vi "DL-SMART-MS-Modify-05-25-6.0.vi"() -> ()   [LabVIEW 2013]
uses:
  <vilib>/Utility/file.llb/Read From Spreadsheet File (DBL).vi
  <userlib>/caLab/Private/CaLabEvent_PV-1D.vi
  <vilib>/Utility/file.llb/Write To Spreadsheet File (DBL).vi
  <userlib>/caLab/Private/Put_DBL-1D_PV.vi
  <userlib>/caLab/Private/Put_I32_PV.vi
  cal_p.vi
  <userlib>/caLab/Private/Get_PV.vi
  <vilib>/vision/driver/NI_Vision_Acquisition_Software.lvlib
  <resource>/objmgr/imaqdx.rc
  <vilib>/Analysis/NI_AALPro.lvlib
panel:
  out "idn status":string
  out "MS":cluster{dbl[], "filtered data":dbl[]}(graph)
  out "std sample":T1(array[cluster])
  in  "Set Laser":bool
  out "Image":T2(plugin-control)
  out "selected id":i32
  out "selected row":i32
  out "currentNO":string
  out "commet":string
  out "sampleID":string
  in  "Shots/Point":i32=100
  in  "chamber in":bool caption="TakeMS"
  in  "chamber out":bool caption="TakeMS"
  in  "Laser parameter":T4
  in  "ADC parameter":T5
  in  "ShutDownSystem":bool
  in  "ADC reference":refnum<vi>
  in  "SetLaserEnergy":dbl(slide) min=0.0 max=50.0 scale=0.0..10.0
  in  "LaserHV":u8=50 min=1 max=100
  in  "频率/Hz":u8=60
  out "Pul.HV-Real":dbl
  out "Identify Spcetrum":cluster{"ID1:X":dbl[], "ID1:Y":dbl[]}[](graph)
  in  "测试记录":i32(listbox)=6
  in  "Identification Results (单靶鉴定结果)":i32(listbox)=2
  in  "HVEnable":bool
  out "GateClose":bool
  out "LaserOK":bool
  out "HV-OK":bool
  out "Vacuum-OK":bool
  in  "Tab Control":T6(tab)
  in  "helix-Zeta-Step":dbl=100.0
  in  "helix-b":dbl=0.2
  in  "AcquireMS-Methods":u8(ring) items=["SinglePoint", "Multipoints", "MultiTar"]
  in  "Thresh":dbl=-0.005 format="%#_13g"
  in  "right rank":i32=2
  in  "left rank":i32=2
  in  "deBaseline":bool
  in  "MCPHV-Set":dbl=1400.0 min=0.0 max=1600.0
  in  "LensHV-Set":dbl=8000.0 min=0.0 max=10000.0
  in  "Tar.HV-Set":dbl=18010.0 min=0.0 max=20000.0
  in  "Pul.HV-Set":dbl=1400.0 min=0.0 max=2000.0
  in  "PulseDelay":dbl
  in  "ADCFreq":dbl
  in  "CH1_Coupling":u64(ring)=2 items=["Volt DC"=1, "Volt AC"=2, "Ampere DC"=4, "Ampere AC"=8, "Ohm"=16]
  in  "Channel 1_Range":dbl(ring)=4.0 items=["80 V"=80.0, "40 V"=40.0, "20 V"=20.0, "8 V"=8.0, "4 V"=4.0, "2 V"=2.0, "800 mV"=0.8, "400 mV"=0.4, "200 mV"=0.2]
  in  "Anal. Setting File":string="High Mass"
  in  "SettingFileSave":bool caption="TakeMS"
  in  "SettingFileAppl":bool caption="TakeMS"
  in  "SettingDel":bool caption="TakeMS"
  in  "RunADC":bool caption="TakeMS"
  out "ADCstatus":bool
  in  "Vac_Prot.":bool
  in  "Turbo_Fore":bool
  in  "Main_Samp":bool
  in  "Samp_Atmos":bool
  in  "Fore_Samp":bool
  in  "StartPump":bool
  in  "SopPump":bool
  out "TurboSpeed":dbl(knob) scale=0.0..100.0
  out "PumpKW":dbl
  out "PumpAmps":dbl
  out "PumpTemp":u16
  out "PumpVolts":dbl
  in  "laser OFF":bool
  in  "laser ON":bool
  out "cluster":T7
  out "A1-position-Y":dbl=45.0 caption="Y" min=0.0 max=55.0
  out "A1-position-X":dbl=53.4 caption="X" min=0.0 max=55.0
  in  "GO":bool
  in  "Y":dbl min=0.0 max=55.0
  in  "X":dbl min=0.0 max=55.0
  in  "A1-Position":bool caption="X-"
  in  "Plat_To_Zero":bool caption="TakeMS"
  in  "Plat_Cal":bool caption="TakeMS"
  out "Y当前":dbl
  out "X当前":dbl
  out "移动":bool
  out "Y满":bool
  out "Y标":bool
  out "X满":bool
  out "Y0":bool
  out "X0":bool
  out "靶位In/Out":bool
  out "仓门":bool
  out "Y过热":bool
  out "X过热":bool
  out "通讯":bool
  in  "Operation Record":i32(listbox)
  in  "OptionRecordLoad 2":bool caption="TakeMS"
  in  "OptionRecordClear":bool caption="TakeMS"
  out "c:":dbl
  out "b:":dbl
  out "a:":dbl
  in  "cancel cal":bool
  in  "cal save":bool
  in  "peak cal":bool
  in  "peak detect":bool
  in  "标准样品":u16(ring) items=["肺炎克雷伯菌", "铜绿假单胞菌"]
  in  "定标参数":i32(listbox)
  out "Tar.HV-Real":dbl
  out "LensHV-Real":dbl
  out "MCPHV-Real":dbl
  out "Lvaccum":dbl=0.83 format="%#_2e"
  out "Hvaccum":dbl=3.4e-05 format="%#_2e"
  in  "H12":bool
  in  "G12":bool
  in  "F12":bool
  in  "E12":bool
  in  "D12":bool
  in  "C12":bool
  in  "B12":bool
  in  "A12":bool
  in  "H11":bool
  in  "G11":bool
  in  "F11":bool
  in  "E11":bool
  in  "D11":bool
  in  "C11":bool
  in  "B11":bool
  in  "A11":bool
  in  "H10":bool
  in  "G10":bool
  in  "F10":bool
  in  "E10":bool
  in  "D10":bool
  in  "C10":bool
  in  "B10":bool
  in  "A10":bool
  in  "H9":bool
  in  "G9":bool
  in  "F9":bool
  in  "E9":bool
  in  "D9":bool
  in  "C9":bool
  in  "B9":bool
  in  "A9":bool
  in  "H8":bool
  in  "G8":bool
  in  "F8":bool
  in  "E8":bool
  in  "D8":bool
  in  "C8":bool
  in  "B8":bool
  in  "A8":bool
  in  "H7":bool
  in  "G7":bool
  in  "F7":bool
  in  "E7":bool
  in  "D7":bool
  in  "C7":bool
  in  "B7":bool
  in  "A7":bool
  in  "H6":bool
  in  "G6":bool
  in  "F6":bool
  in  "E6":bool
  in  "D6":bool
  in  "C6":bool
  in  "B6":bool
  in  "A6":bool
  in  "H5":bool
  in  "G5":bool
  in  "F5":bool
  in  "E5":bool
  in  "D5":bool
  in  "C5":bool
  in  "B5":bool
  in  "A5":bool
  in  "H4":bool
  in  "G4":bool
  in  "F4":bool
  in  "E4":bool
  in  "D4":bool
  in  "C4":bool
  in  "B4":bool
  in  "A4":bool
  in  "H3":bool
  in  "G3":bool
  in  "F3":bool
  in  "E3":bool
  in  "D3":bool
  in  "C3":bool
  in  "B3":bool
  in  "A3":bool
  in  "H2":bool
  in  "G2":bool
  in  "F2":bool
  in  "E2":bool
  in  "D2":bool
  in  "C2":bool
  in  "B2":bool
  in  "A2":bool
  in  "H1":bool
  in  "G1":bool
  in  "F1":bool
  in  "E1":bool
  in  "D1":bool
  in  "C1":bool
  in  "B1":bool
  in  "A1":bool
  in  "Clear":bool caption="TakeMS"
  in  "Add":bool caption="TakeMS"
  in  "TakeMS-Stop":bool caption="TakeMS"
  in  "TakeMS-Run":bool caption="TakeMS"
  # "Laser (激光)"
  # "Acq.(采谱)"
  # "Vacuum(真空)"
  # "Pa"
  # "High"
  # "1"
  # "2"
  # "3"
  # "4"
  # "5"
  # "6"
  # "7"
  # "8"
  # "9"
  # "10"
  # "11"
  # "12"
  # "A"
  # "Low"
  # "Pa"
  # "B"
  # "H.V.(高压)"
  # "C"
  # "D"
  # "MCP"
  # "V"
  # "E"
  # "Tar."
  # "V"
  # "F"
  # "Pul."
  # "V"
  # "G"
  # "Lens"
  # "V"
  # "H"
  # "Vauum (真空)"
  # "H.V. (高压)"
  # "Laser (激光)"
  # "Gate (仓门)"
  # "mm"
  # "Radian"
  # "H.V. (高压参数)"
  # "ADC(采集卡设置)"
  # "ADCFreq(采样)"
  # "MCP (探测器)"
  # "V"
  # "Hz"
  # "Tar. (靶)"
  # "V"
  # "Setting File(设置文件)"
  # "Coupling"
  # "Pulse (脉冲)"
  # "V"
  # "IntRange"
  # "V"
  # "Lens (透镜)"
  # "Delay (延时)"
  # "ns"
  # "Sole. Valves"
  # "Turbo Pump"
  # "自锁保护"
  # "机械/分子"
  # "主仓/样仓"
  # "样仓/大气"
  # "机械/样仓"
  # "激光器状态"
  # "mm"
  # "mm"
  # "mm"
  # "mm"
  # "mm"
  # "mm"
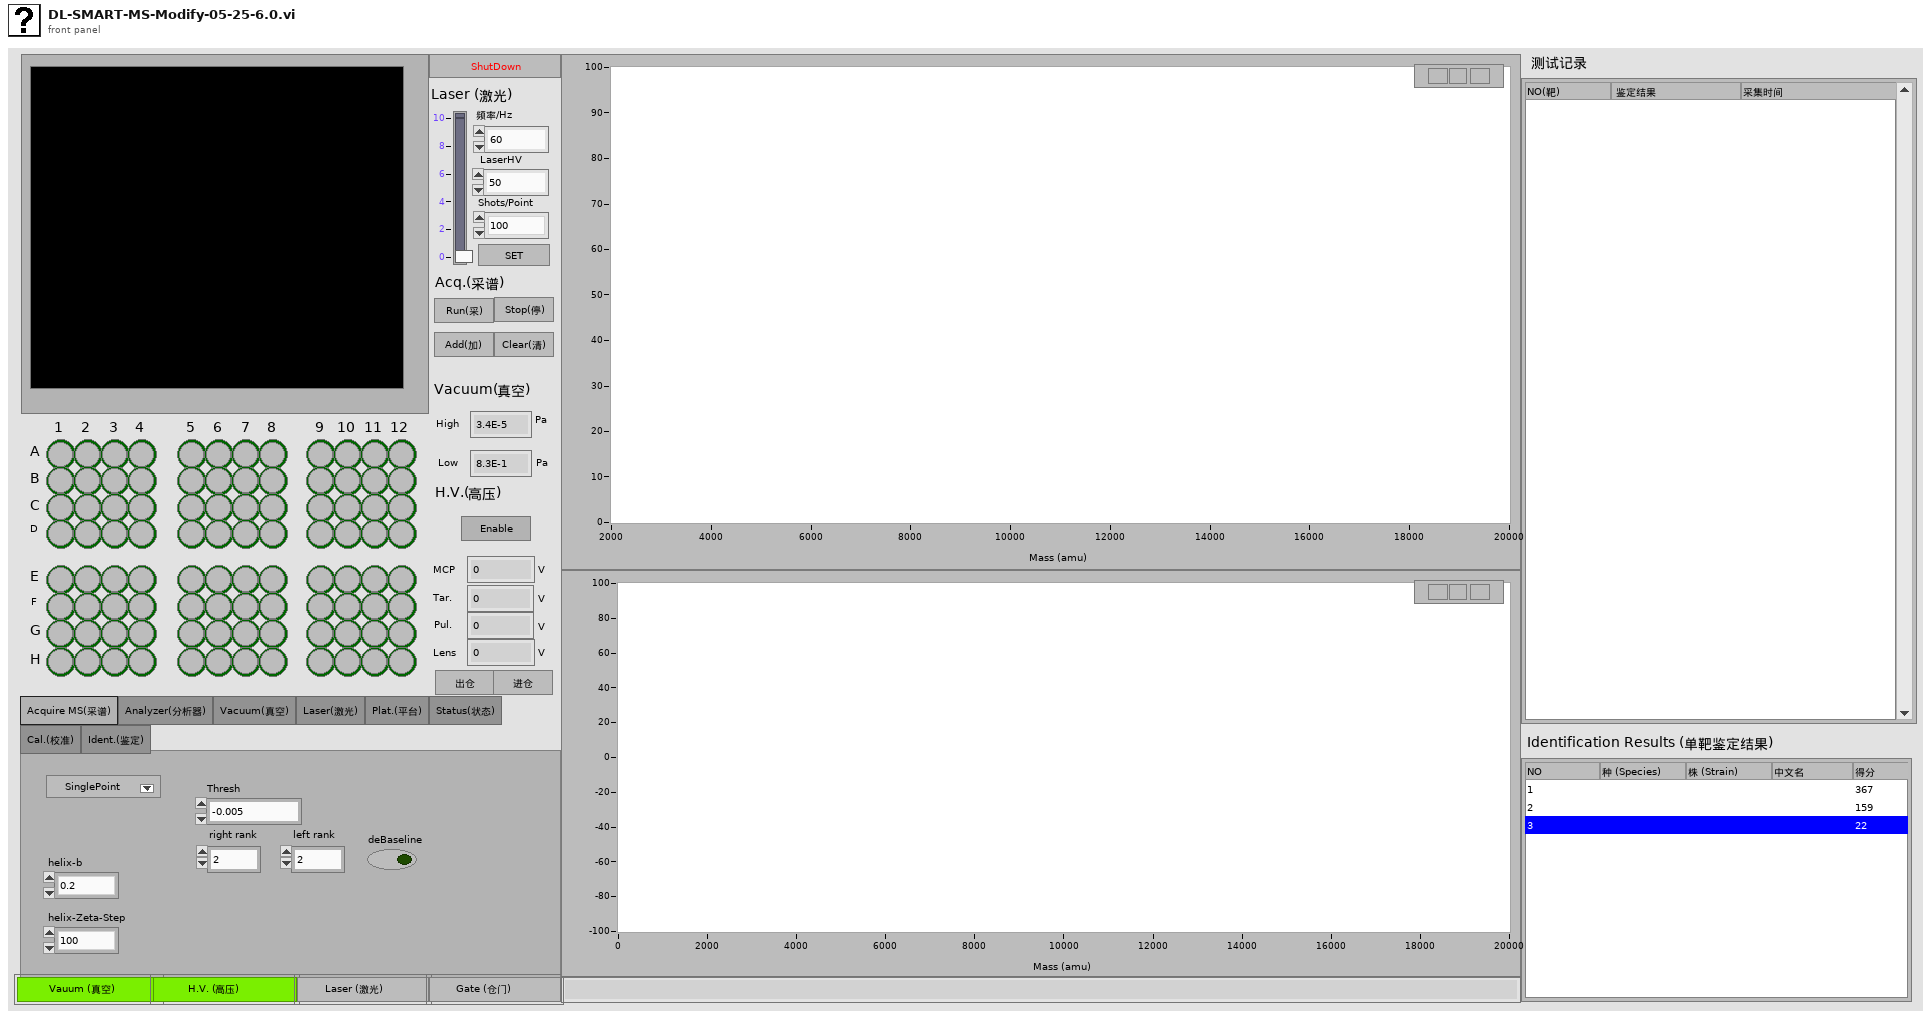
[diagram p1: front panel]
types:
  T1 = cluster{"name":string, "mz":dbl[], "time":dbl[]}[]
  T2 = typedef "IMAQ Image.ctl" = refnum<image>
  T3 = typedef "Semaphore RefNum" = refnum<k1>
  T4 = cluster{"VISA resource name":refnum<visa-resource-name>, "standby":bool, "semaphore in":T3, "SetLaserEnergy":dbl}
  T5 = cluster{"TpDeviceHandle_t":u32, "Record Length/Samples":u64, "ShotsPerPoint":u16}
  T6 = enum32{"Acquire MS(采谱)", "Analyzer(分析器)", "Vacuum(真空)", "Laser(激光)", "Plat.(平台)", "Status(状态)", "Cal.(校准)", "Ident.(鉴定)"}
  T7 = cluster{"链接":bool, "待机":bool, "发射":bool, "[3]":bool, "内存":bool, "测能":bool, "温警":bool, "静态":bool, "操作":bool}
  T8 = cluster{"tag1":string, "tag2":string, "x":dbl[], "y":dbl[], "ID1:X":dbl[], "ID1:Y":dbl[], "ID1:REF:X":dbl[], "ID1:REF:Y":dbl[], "ID2:X":dbl[], "ID2:Y":dbl[], "ID2:REF:X":dbl[], "ID2:REF:Y":dbl[], "ID3:X":dbl[], "ID3:Y":dbl[], "ID3:REF:X":dbl[], "ID3:REF:Y":dbl[], "ID1:TAG1":string, "ID1:TAG2":string, "ID2:TAG1":string, "ID2:TAG2":string, "ID3:TAG1":string, "ID3:TAG2":string, "ID1:NAME":string, "ID2:NAME":string, "ID3:NAME":string, "ID1:SCORE":string, "ID2:SCORE":string, "ID3:SCORE":string, "NO":string}[]
  T9 = cluster{"laser semaphore":T3, "pump semaphore":T3}
  T10 = enum8{"Enabled", "Disabled", "Disabled and Grayed Out"}
  T11 = cluster{"tag1":string, "tag2":string, "x":dbl[], "y":dbl[], "ID1:X":dbl[], "ID1:Y":dbl[], "ID1:REF:X":dbl[], "ID1:REF:Y":dbl[], "ID2:X":dbl[], "ID2:Y":dbl[], "ID2:REF:X":dbl[], "ID2:REF:Y":dbl[], "ID3:X":dbl[], "ID3:Y":dbl[], "ID3:REF:X":dbl[], "ID3:REF:Y":dbl[], "ID1:TAG1":string, "ID1:TAG2":string, "ID2:TAG1":string, "ID2:TAG2":string, "ID3:TAG1":string, "ID3:TAG2":string, "ID1:NAME":string, "ID2:NAME":string, "ID3:NAME":string, "ID1:SCORE":string, "ID2:SCORE":string, "ID3:SCORE":string, "NO":string}
  T12 = cluster{"monitor":refnum<user-event>, "motor status":refnum<user-event>, "motor":refnum<user-event>, "notifier out":refnum<notifier>, "queue out":refnum<queue>, "AI":T3, "DI":T3, "CX":T3, "CY":T3}
  T13 = cluster{"AI Task":refnum<k21>, "AO Task":refnum<k21>, "DO Task":refnum<k21>, "DI Task":refnum<k21>, "PWM x":refnum<k21>, "PWM y":refnum<k21>, "counter x":refnum<k21>, "counter y":refnum<k21>}
  T14 = cluster{"tasks":cluster{"AI Task":refnum<k21>, "AO Task":refnum<k21>, "DO Task":refnum<k21>, "DI Task":refnum<k21>, "PWM x":refnum<k21>, "PWM y":refnum<k21>, "counter x":refnum<k21>, "counter y":refnum<k21>}, "interface":cluster{"monitor":refnum<user-event>, "motor status":refnum<user-event>, "motor":refnum<user-event>, "notifier out":refnum<notifier>, "queue out":refnum<queue>, "AI":T3, "DI":T3, "CX":T3, "CY":T3}, "error out":errorcluster}
  T15 = cluster{"ConfiguredPumpCom":refnum<visa-resource-name>, "ConfiguredLaserCom":refnum<visa-resource-name>}
  T16 = typedef "LVPoint32TypeDef.ctl" = cluster{"Horizontal":i32, "Vertical":i32}
  T17 = typedef "LVRowAndColumnTypeDef.ctl" = cluster{"Row":i32, "Column":i32}
  T18 = cluster{"Type":u32, "Version":u32, "Flags":u32, "SerialNumberHigh":u32, "SerialNumberLow":u32, "BusType":u32, "InterfaceName":string, "VendorName":string, "ModelName":string, "CameraFileName":string, "CameraAttributeURL":string}[]
  T19 = cluster{"Type":u32, "Version":u32, "Flags":u32, "SerialNumberHigh":u32, "SerialNumberLow":u32, "BusType":u32, "InterfaceName":string, "VendorName":string, "ModelName":string, "CameraFileName":string, "CameraAttributeURL":string}
  T20 = typedef "IMAQdx.ctl" = refnum<k21>
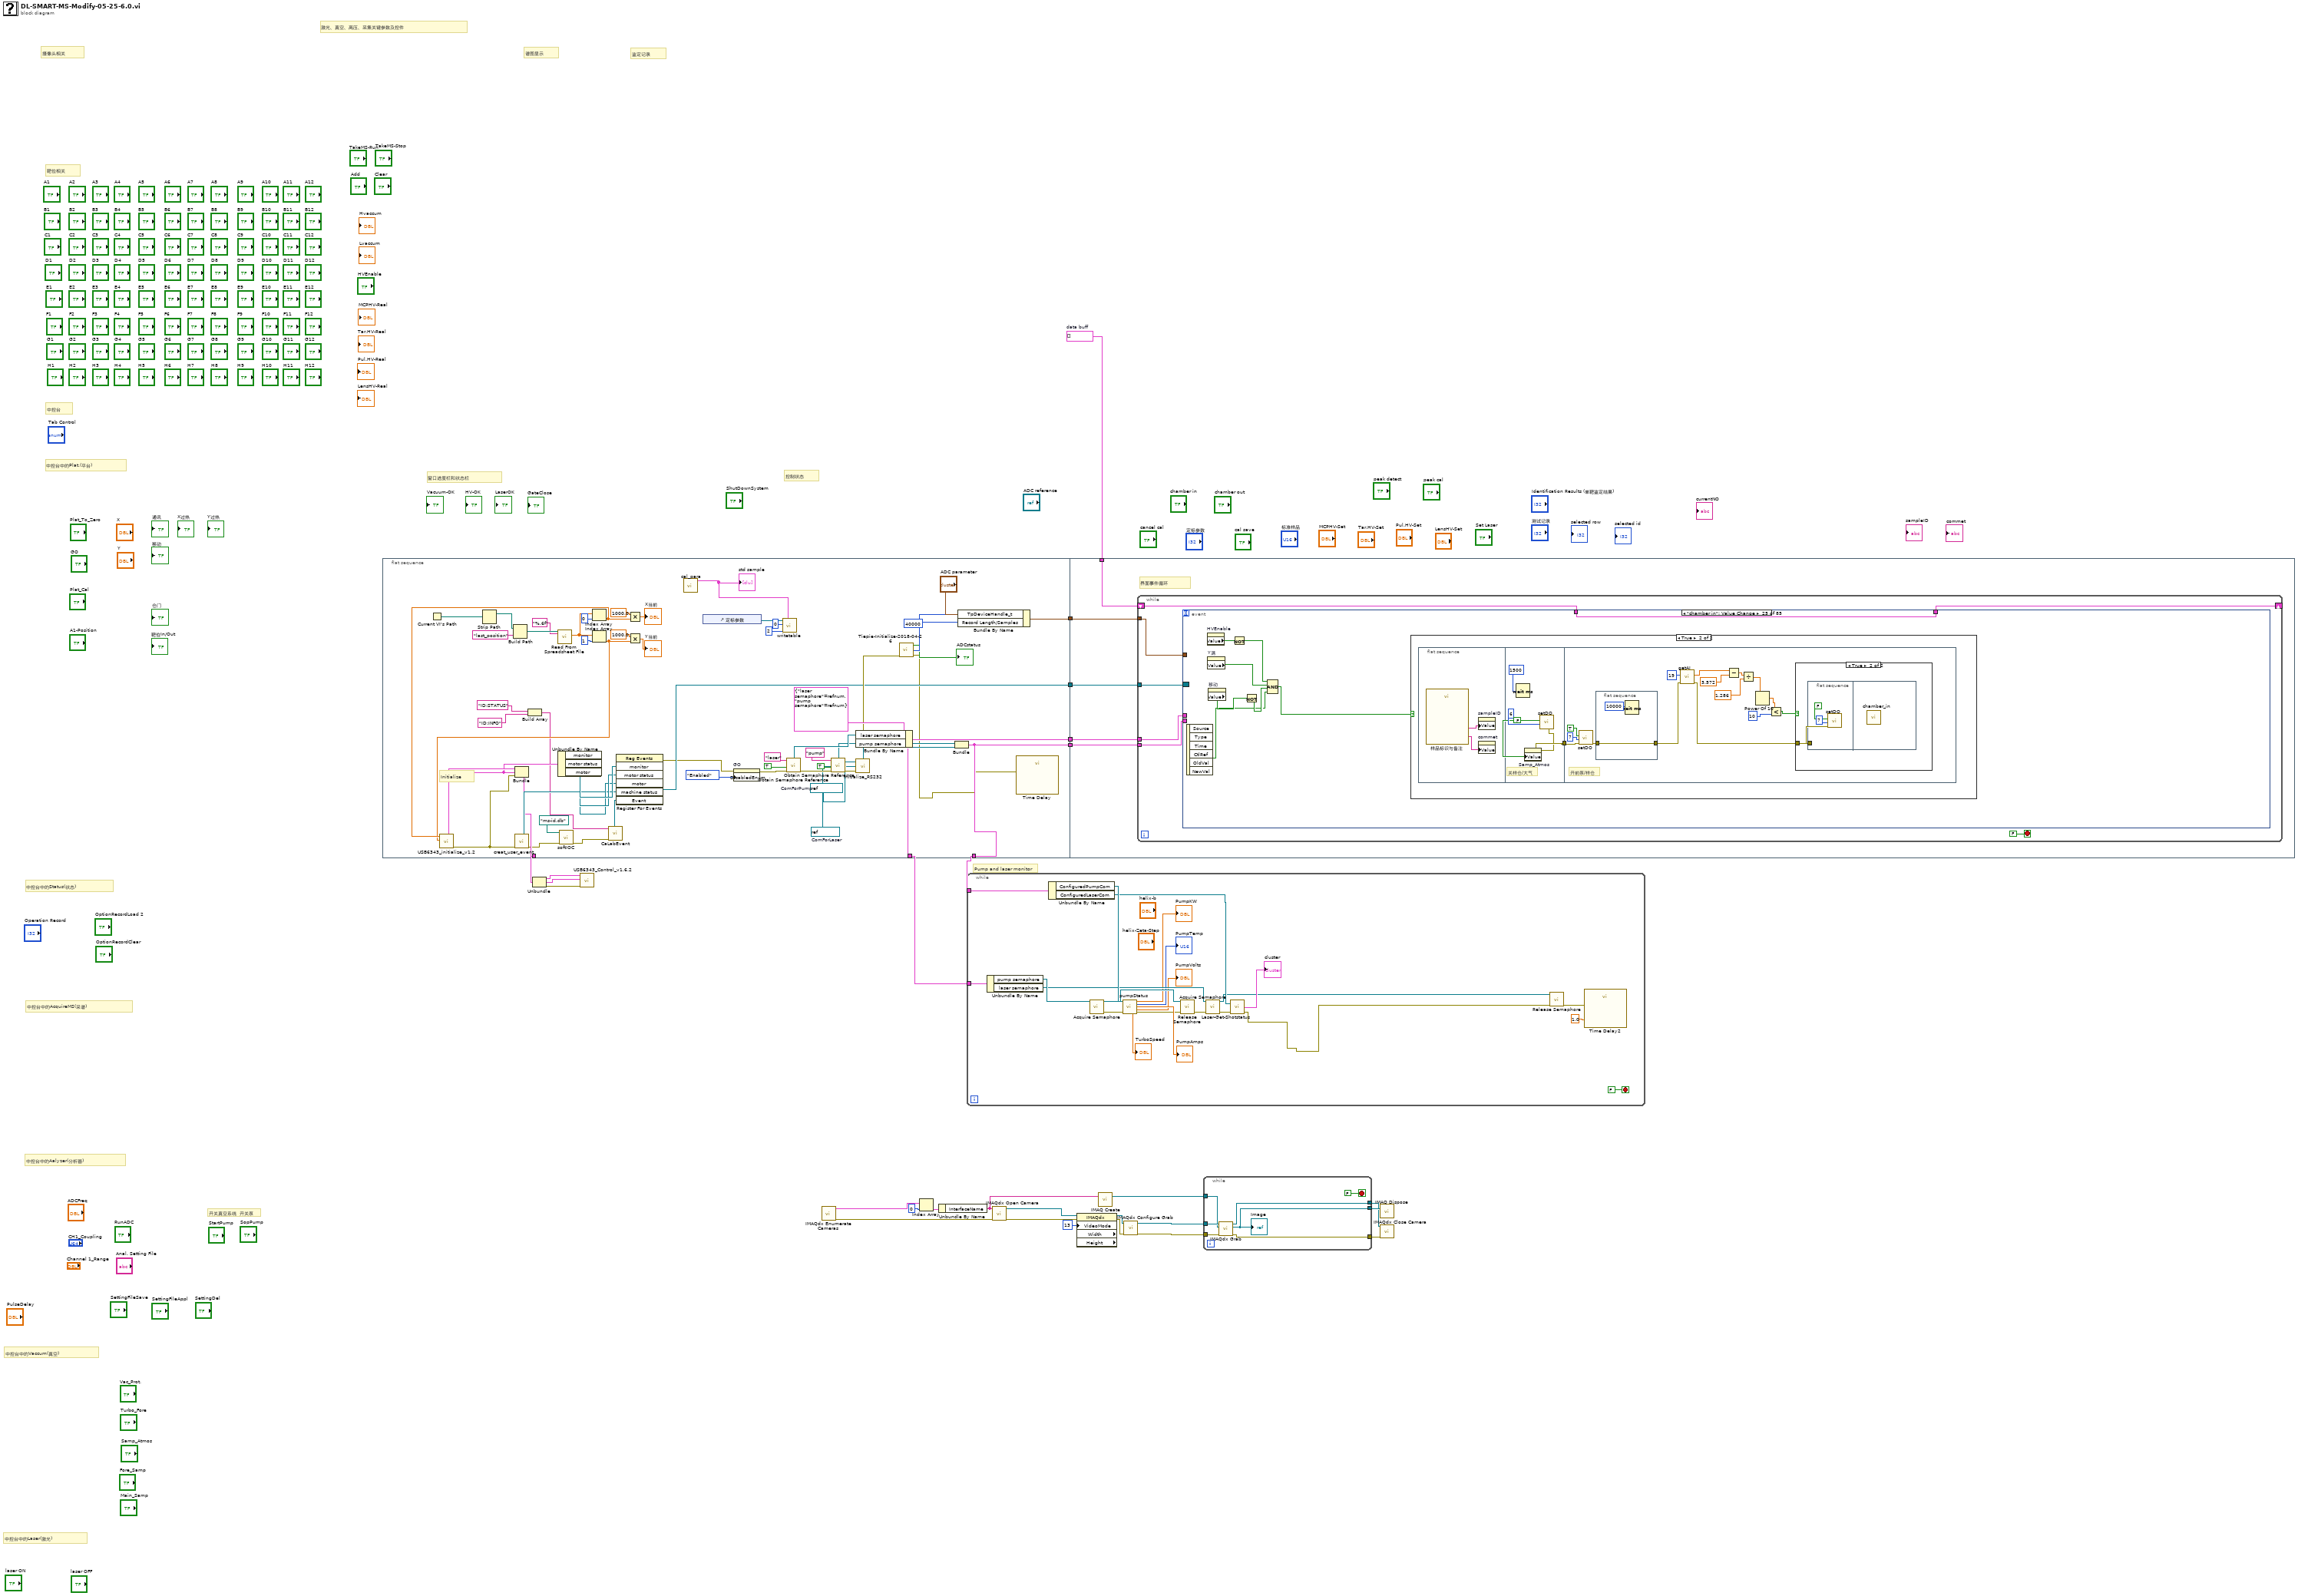
[diagram p0: block diagram]
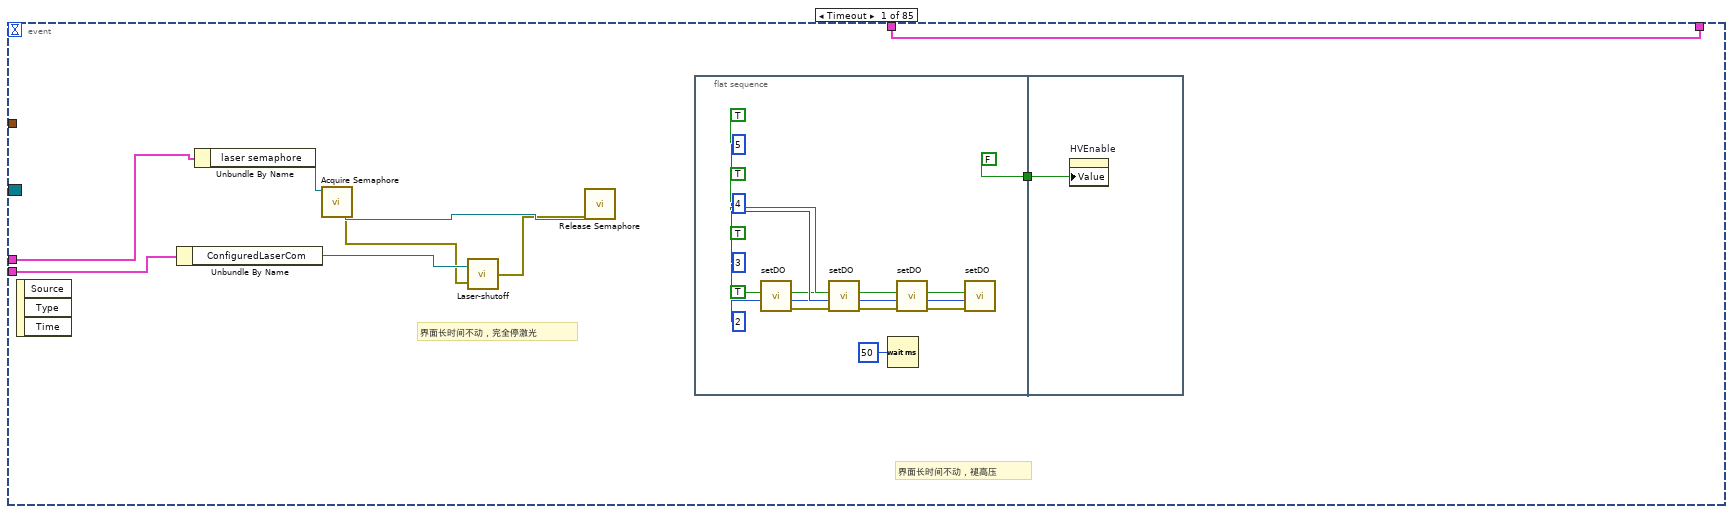
[diagram p2: hidden frame]
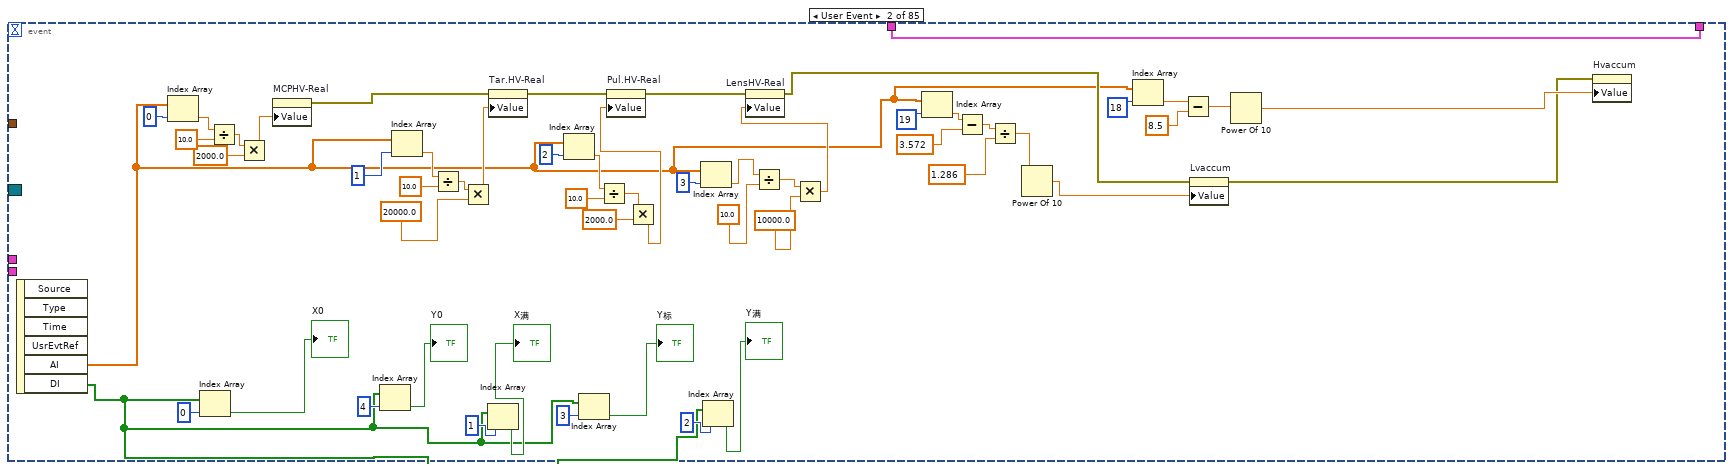
[diagram p3: hidden frame]
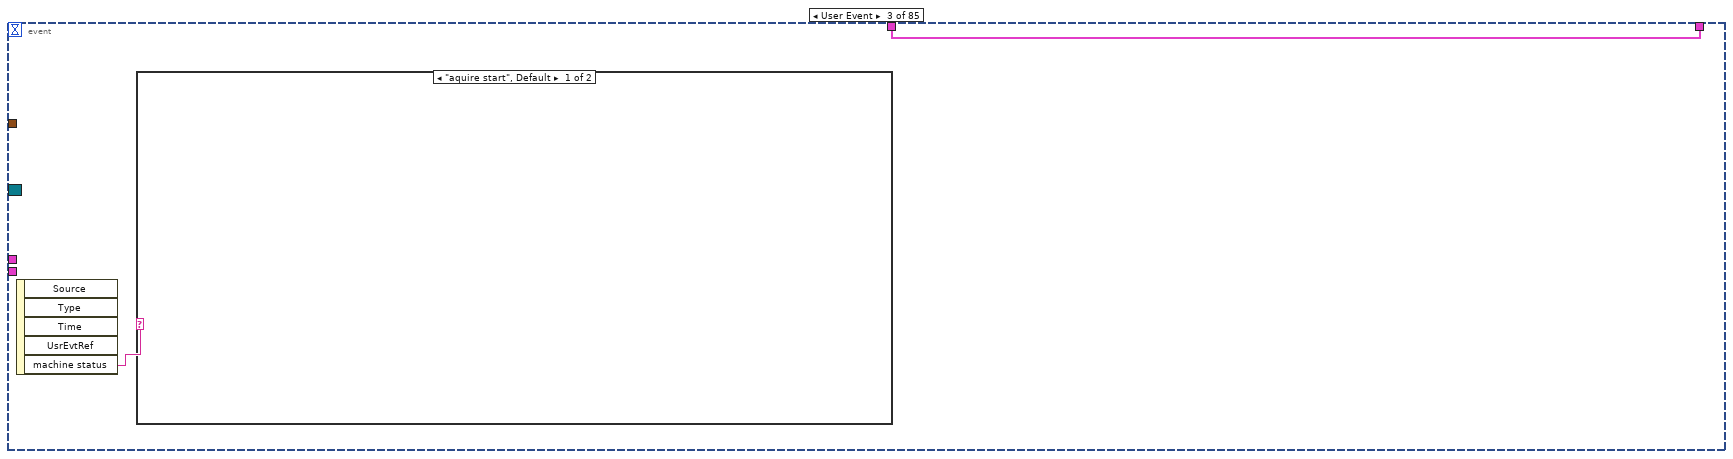
[diagram p4: hidden frame]
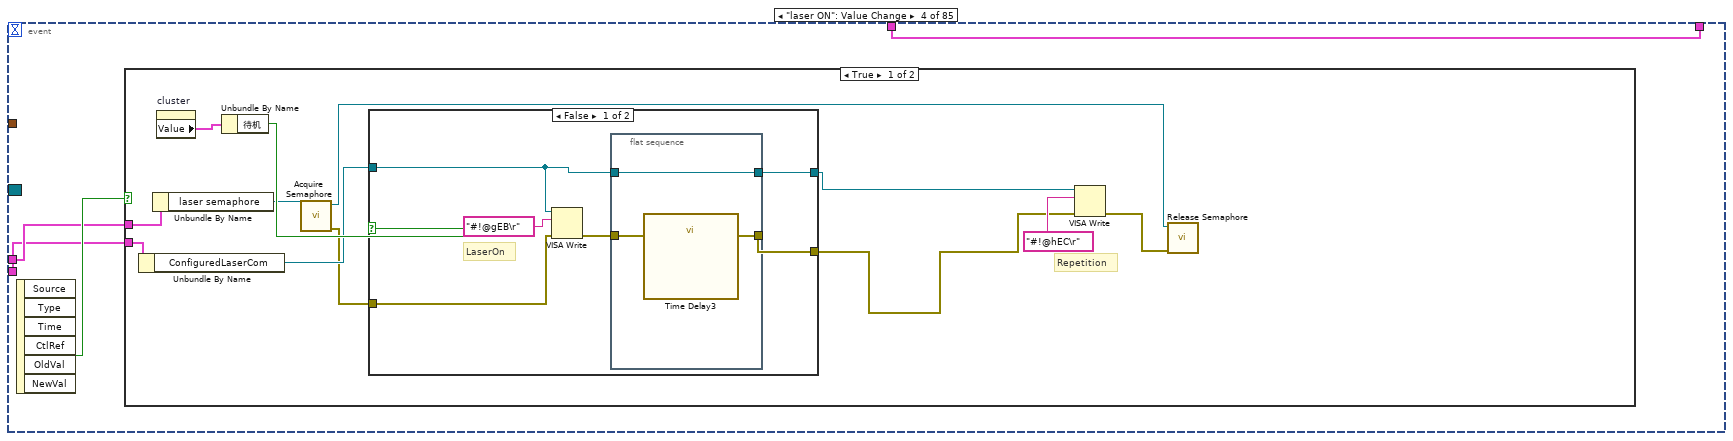
[diagram p6: hidden frame]
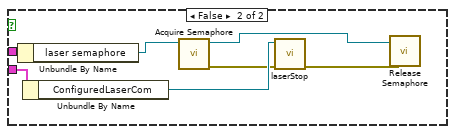
[diagram p8: hidden frame]
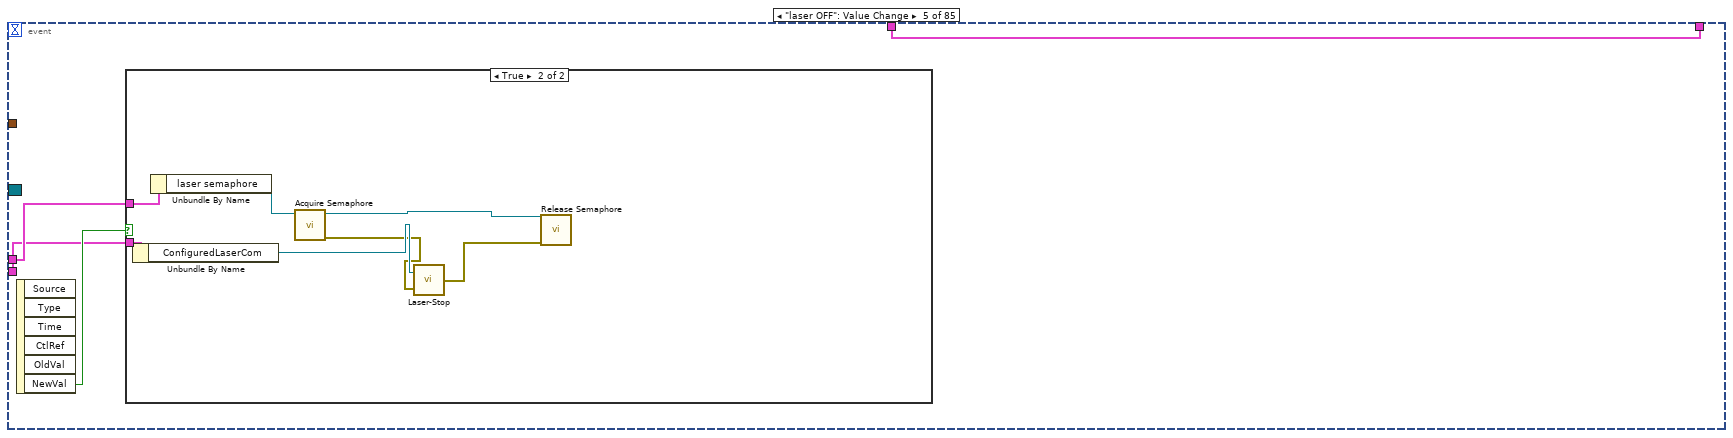
[diagram p9: hidden frame]
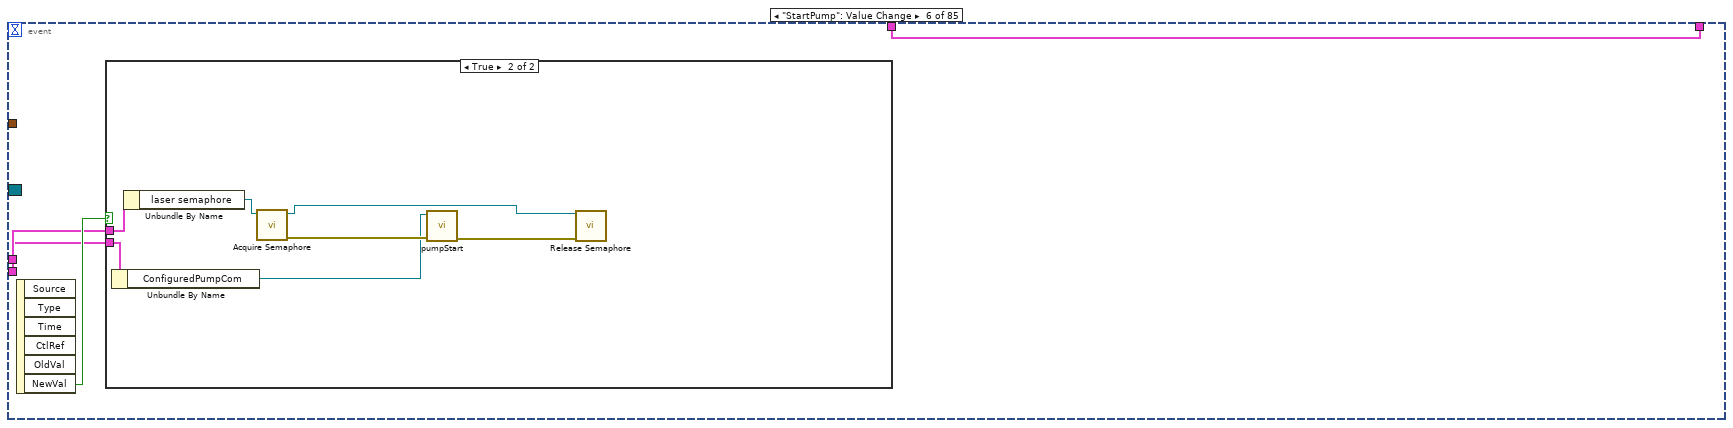
[diagram p11: hidden frame]
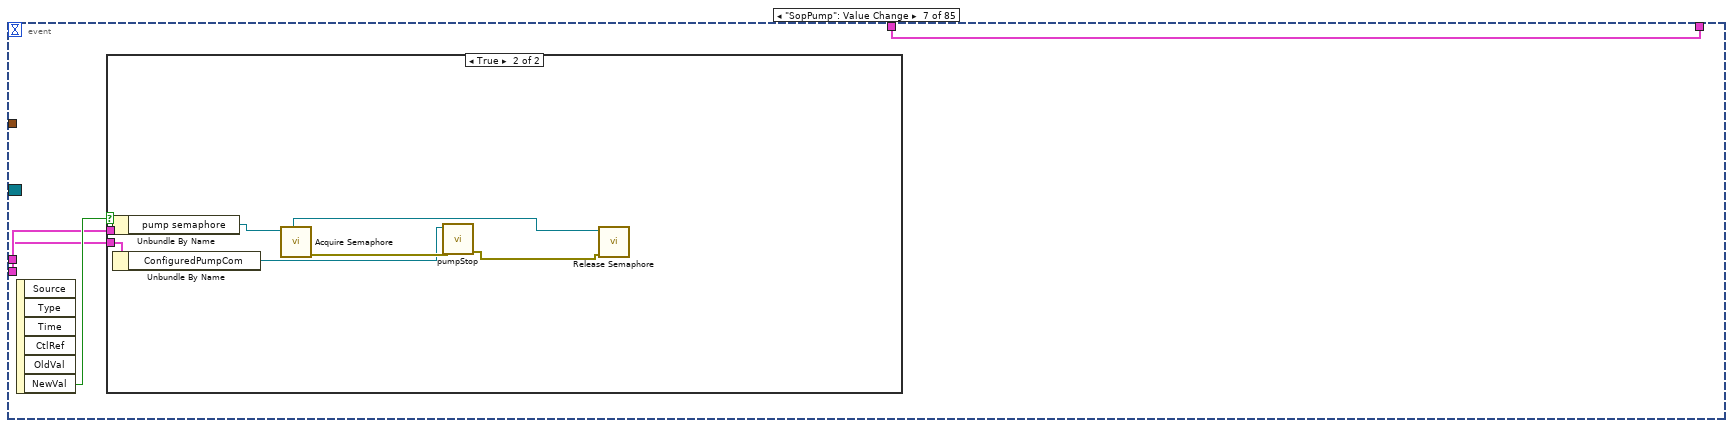
[diagram p13: hidden frame]
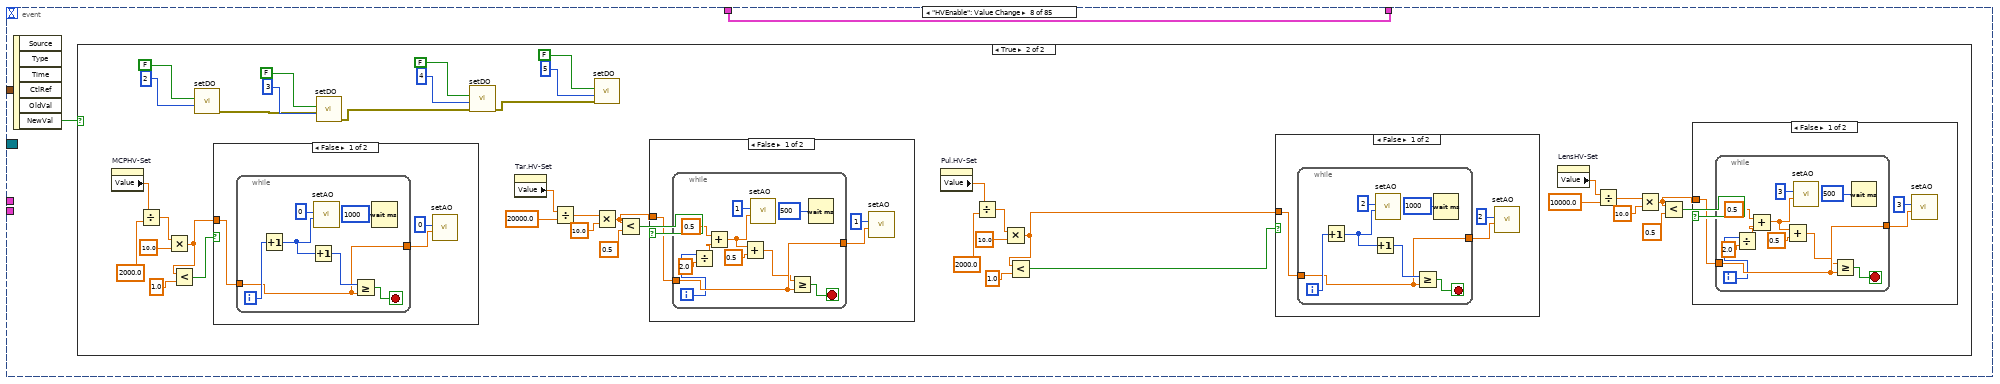
[diagram p15: hidden frame]
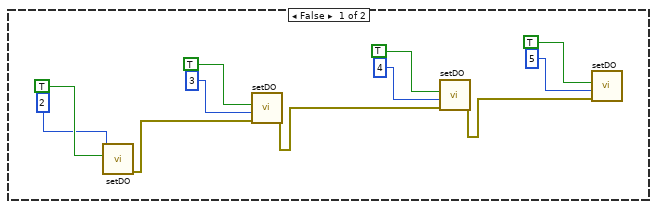
[diagram p16: hidden frame]
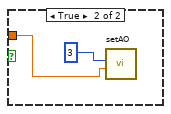
[diagram p17: hidden frame]
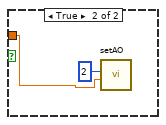
[diagram p18: hidden frame]
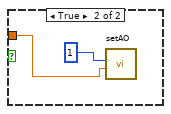
[diagram p19: hidden frame]
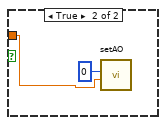
[diagram p20: hidden frame]
diagram:
  w20 = T8 []  # data buff
  # "Pump and laser monitor"
  # "开关真空系统  开关泵"
  # "控制状态"
  # "鉴定记录"
  # "谱图显示"
  # "激光、真空、高压、采集关键参数及控件"
  # "窗口进度栏和状态栏"
  # "中控台中的Laser(激光)"
  # "中控台中的Vaccum(真空)"
  # "中控台中的Aalyzer(分析器)"
  # "中控台中的AcquireMS(采谱)"
  # "中控台中的Status(状态)"
  # "中控台中的Plat.(平台)"
  # "中控台"
  # "靶位相关"
  # "摄像头相关"
  n1 = flat-sequence {
    tunnel: [w40] -> w27
    tunnel: [w65] -> w26
    tunnel: [w65] -> w24
    tunnel: [w64] -> w25
    tunnel: [w64] -> w23
    tunnel: [w68] -> w22
    tunnel: [w57] -> w21
    tunnel: w27 -> [w91]
    tunnel: w26 -> [w90]
    tunnel: w25 -> [w89]
    tunnel: w21 -> [w88]
    tunnel: w20 -> [w87]
    frame #0 {
      w62 = refnum<visa-resource-name> "COM9"  # ComForLaser
      w63 = refnum<visa-resource-name> "COM10"  # ComForPump
      # "Initialize"
      n2 = Current VI's Path() -> (path=w55:path)
      n3 = Strip Path(path=w55) -> (stripped path=w54:path)  [unwired: 1 out]
      n4 = Build Path(base path=w54, name or relative path="last_position") -> (appended path=w52:path)
      n5 = Build Array("ID:STATUS", "ID:INFO") -> (w28:string[])
      n6 = call-poly <vilib>:"Read From Spreadsheet File.vi"("format (%.3f)"="%.6f", "file path (dialog if empty)"=w52) -> ("first row"=w50:dbl[])  [unwired: 5 in, 4 out]
      n7 = Index Array(array=w50, index=0) -> (element=w47:dbl)
      n8 = Index Array(array=w50, index=1) -> (element=w44:dbl)
      n9 = call "USB6343_initialize_v1.2.vi"("Y initial position"=w44, "X initial position"=w47) -> ("error out"=w69:errorcluster, "interface"=w70:T12, "tasks"=w71:T13)  [unwired: 7 in]
      n10 = Bundle("tasks"=w71, "interface"=w70, "error out"=w69) -> (w68:T14)  [unwired: 1 in]
      n11 = call "creat_user_event.vi"("error in (no error)"=w69) -> ("error out"=w36:errorcluster, "machine status"=w79:refnum<user-event>)  [unwired: 9 in]
      n12 = Unbundle By Name(w70) -> ("monitor"=w86:refnum<user-event>, "motor status"=w85:refnum<user-event>, "motor"=w84:refnum<user-event>)
      n13 = call "softIOC.vi"("error in (no error)"=w36, "路径"=path "ms-id.db") -> ("error out"=w37:errorcluster)  [unwired: 8 in, 1 out]
      n14 = call-poly <userlib>:"CaLabEvent.vi"("error in (no error)"=w37, "PV Names"=w28) -> ("Event"=w39:refnum<user-event>)  [unwired: 7 in, 2 out]
      n15 = register-events(w86, w85, w84, w79, w39) -> (reference out=w40:refnum<event-registration>, error out=w35:errorcluster)  [unwired: 2 in]
      n16 = Multiply(x=1000.0, y=w47) -> (x*y=→"X当前":dbl)
      n17 = Multiply(x=1000.0, y=w44) -> (x*y=→"Y当前":dbl)
      n18 = call "cal_para.vi"() -> ("std sample"=w32:T1)  [unwired: 11 in]
      "std sample" <- w32
      n19 = control-ref of="定标参数"() -> (w34:refnum<vi>)
      n20 = property on="GO" class="Bool (strict)"(error in=w35, "DisabledEnum"=T10."Enabled" ("Disabled")) -> (error out=w80:errorcluster)  [unwired: 1 in, 1 out]
      n21 = call "writetable.vi"("std sample"=w32, "col"=2, "type"=0, "reference"=w34) -> ()  [unwired: 8 in]
      n22 = call <vilib>:"Obtain Semaphore Reference.vi"("error in (no error)"=w80, "create if not found (T)"=TRUE, "name (unnamed)"="laser") -> ("error out"=w75:errorcluster, "semaphore"=w72:T3)  [unwired: 2 in, 1 out]
      n23 = call <vilib>:"Obtain Semaphore Reference.vi"("error in (no error)"=w75, "create if not found (T)"=TRUE, "name (unnamed)"="pump") -> ("error out"=w74:errorcluster, "semaphore"=w66:T3)  [unwired: 2 in, 1 out]
      n24 = Bundle By Name(cluster=T9 {"laser semaphore"=refnum, "pump semaphore"=refnum}, "laser semaphore"=w72, "pump semaphore"=w66) -> (w65:T9)
      n25 = call "Initialize_RS232.vi"("error in (no error)"=w74, "ComForLaser"=w62, "ComForPump"=w63) -> ("error out"=w61:errorcluster, "ConfiguredLaserCom"=w77:refnum<visa-resource-name>, "ConfiguredPumpCom"=w78:refnum<visa-resource-name>)
      n26 = call "Tiepie-Initialize-2018-04-26.vi"("error in (no error)"=w61) -> ("error out"=w38:errorcluster, "TpDeviceHandle_t"=w59:u32, "Card-OK"=→"ADCstatus":bool)  [unwired: 3 in]
      n27 = Bundle("ConfiguredPumpCom"=w78, "ConfiguredLaserCom"=w77) -> (w64:T15)  [unwired: 1 in]
      n28 = Bundle By Name(cluster="ADC parameter", "TpDeviceHandle_t"=w59, "Record Length/Samples"=u64 40000) -> (w57:T5)
      n29 = call "Time Delay"("error in (no error)"=w38) -> ()  [unwired: 10 in, 1 out]
    }
    frame #1 {
      # "界面事件循环"
      n30 = while {
        tunnel: w91 -> [w98]
        tunnel: w89 -> [w97]
        tunnel: w90 -> [w96]
        tunnel: w88 -> [w94]
        shift-right: [w92] -> _
        shift-left: w87 -> [w93]
        stop <- FALSE stop-if-true
        n31 = event shown="[24] \"chamber in\": Value Change" {
          selector: w98 -> [_ _ _ _ _ _ _ _ _ _ _ _ _ _ _ _ _ _ _ _ _ _ _ _ _ _ _ _ _ _ _ _ _ _ _ _ _ _ _ _ _ _ _ _ _ _ _ _ _ _ _ _ _ _ _ _ _ _ _ _ _ _ _ _ _ _ _ _ _ _ _ _ _ _ _ _ _ _ _ _ _ _ _ _ _]
          dyn-events: _ -> [_ _ _ _ _ _ _ _ _ _ _ _ _ _ _ _ _ _ _ _ _ _ _ _ _ _ _ _ _ _ _ _ _ _ _ _ _ _ _ _ _ _ _ _ _ _ _ _ _ _ _ _ _ _ _ _ _ _ _ _ _ _ _ _ _ _ _ _ _ _ _ _ _ _ _ _ _ _ _ _ _ _ _ _ _]
          timeout: _ -> [_ _ _ _ _ _ _ _ _ _ _ _ _ _ _ _ _ _ _ _ _ _ _ _ _ _ _ _ _ _ _ _ _ _ _ _ _ _ _ _ _ _ _ _ _ _ _ _ _ _ _ _ _ _ _ _ _ _ _ _ _ _ _ _ _ _ _ _ _ _ _ _ _ _ _ _ _ _ _ _ _ _ _ _ _]
          tunnel: w97 -> [w101 _ _ w179 w212 w223 w234 _ _ _ _ _ _ _ _ _ _ w460 w511 _ _ _ _ _ _ _ _ _ _ _ _ _ _ _ _ _ _ _ _ _ _ _ _ _ _ _ _ _ _ _ _ _ _ _ _ _ _ _ _ _ _ _ _ _ _ _ _ _ _ _ _ _ _ _ _ _ _ _ _ _ _ _ _ _ w1759]
          tunnel: w96 -> [w102 _ _ w180 w213 w224 w235 _ _ _ _ _ _ _ _ _ _ w461 w512 _ _ _ _ _ _ _ _ _ _ _ _ _ _ _ _ _ _ _ _ _ _ _ _ _ _ _ _ _ _ _ _ _ _ _ _ _ _ _ _ _ _ _ _ _ _ _ _ _ _ _ _ _ _ _ _ _ _ _ _ _ _ _ _ _ _]
          tunnel: w94 -> [_ _ _ _ _ _ _ _ _ _ _ _ _ _ _ _ _ w462 _ _ _ _ _ _ _ _ _ _ _ _ _ _ _ _ _ _ _ _ _ _ _ _ _ _ _ _ _ _ _ _ _ _ _ _ _ _ _ _ _ _ _ _ _ _ _ _ _ _ _ _ _ _ _ _ _ _ _ _ _ _ _ _ _ _ _]
          tunnel: w93 -> [w99 w122 w176 w178 w211 w222 w233 w244 w352 w367 w382 w389 w396 w403 w410 w418 w443 w459 w514 w526 w556 w591 w630 w632 w646 w686 w720 w722 w761 w766 w782 w800 w817 w834 w851 w868 w887 w912 w929 w946 w963 w980 w997 w1016 w1035 w1054 w1073 w1092 w1110 w1128 w1146 w1164 w1182 w1200 w1218 w1236 w1254 w1272 w1290 w1308 w1326 w1344 w1362 w1380 w1398 w1416 w1434 w1452 w1470 w1488 w1506 w1524 w1542 w1564 w1582 w1600 w1618 w1636 w1654 w1672 w1690 w1708 w1726 w1744 w1758]
          tunnel: [w99 w122 w176 w178 w211 w222 w233 w244 w352 w367 w382 w389 w396 w403 w410 w418 w443 w458 w514 w525 w556 w591 w630 w632 w646 w686 w720 w722 w761 w766 w782 w800 w817 w834 w851 w868 w886 w912 w929 w946 w963 w980 w997 w1016 w1035 w1054 w1073 w1092 w1110 w1128 w1146 w1164 w1182 w1200 w1218 w1236 w1254 w1272 w1290 w1308 w1326 w1344 w1362 w1380 w1398 w1416 w1434 w1452 w1470 w1488 w1506 w1524 w1542 w1564 w1582 w1600 w1618 w1636 w1654 w1672 w1690 w1708 w1726 w1744 w1758] -> w92
          event Timeout {
            # "界面长时间不动，褪高压"
            # "界面长时间不动，完全停激光"
            n32 = event-data() -> ()  [unwired: 1 in, 3 out]
            n33 = Unbundle By Name(w101) -> ("ConfiguredLaserCom"=w105:refnum<visa-resource-name>)
            n34 = Unbundle By Name(w102) -> ("laser semaphore"=w107:T3)
            n35 = call <vilib>:"Acquire Semaphore.vi"("semaphore"=w107) -> ("error out"=w104:errorcluster, "semaphore out"=w106:T3)  [unwired: 4 in, 1 out]
            n36 = call "Laser-shutoff.vi"("error in (no error)"=w104, "VISA resource name"=w105) -> ("error out"=w103:errorcluster)
            n37 = call <vilib>:"Release Semaphore.vi"("error in (no error)"=w103, "semaphore"=w106) -> ()  [unwired: 4 in, 2 out]
            n38 = flat-sequence {
              tunnel: [FALSE ("HVEnable")] -> w100
              tunnel: w100 -> [w121]
              frame #0 {
                n39 = call "setDO.vi"("channel"=2, "on/off"=TRUE) -> ("错误输出"=w118:errorcluster)  [unwired: 9 in]
                n40 = call "setDO.vi"("错误输入（无错误）"=w118, "channel"=3, "on/off"=TRUE) -> ("错误输出"=w119:errorcluster)  [unwired: 8 in]
                n41 = Wait (ms)(milliseconds to wait=u32 50) -> ()  [unwired: 1 out]
                n42 = call "setDO.vi"("错误输入（无错误）"=w119, "channel"=4, "on/off"=TRUE) -> ("错误输出"=w120:errorcluster)  [unwired: 8 in]
                n43 = call "setDO.vi"("错误输入（无错误）"=w120, "channel"=5, "on/off"=TRUE) -> ()  [unwired: 8 in, 1 out]
              }
              frame #1 {
                n44 = property on="HVEnable" class="Bool (strict)"("Value"=w121) -> ()  [unwired: 2 in, 2 out]
              }
            }
          }
          event User Event {
            n45 = event-data() -> ("AI"=w134:dbl[], "DI"=w159:bool[])  [unwired: 1 in, 4 out]
            n46 = Index Array(array=w134, index=0) -> (element=w157:dbl)
            n47 = Index Array(array=w159, index=0) -> (element=→"X0":bool)
            n48 = Divide(x=w157, y=10.0) -> (x/y=w155:dbl)
            n49 = Multiply(x=w155, y=2000.0) -> (x*y=w153:dbl)
            n50 = property on="MCPHV-Real" class="DigNum (strict)"("Value"=w153) -> (error out=w175:errorcluster)  [unwired: 2 in, 1 out]
            n51 = Index Array(array=w159, index=4) -> (element=→"Y0":bool)
            n52 = Index Array(array=w134, index=1) -> (element=w152:dbl)
            n53 = Divide(x=w152, y=10.0) -> (x/y=w150:dbl)
            n54 = Multiply(x=w150, y=20000.0) -> (x*y=w148:dbl)
            n55 = Index Array(array=w159, index=1) -> (element=→"X满":bool)
            n56 = property on="Tar.HV-Real" class="DigNum (strict)"(error in=w175, "Value"=w148) -> (error out=w174:errorcluster)  [unwired: 1 in, 1 out]
            n57 = Index Array(array=w134, index=2) -> (element=w147:dbl)
            n58 = Index Array(array=w159, index=3) -> (element=→"Y标":bool)
            n59 = Divide(x=w147, y=10.0) -> (x/y=w145:dbl)
            n60 = Multiply(x=w145, y=2000.0) -> (x*y=w143:dbl)
            n61 = property on="Pul.HV-Real" class="DigNum (strict)"(error in=w174, "Value"=w143) -> (error out=w173:errorcluster)  [unwired: 1 in, 1 out]
            n62 = Index Array(array=w134, index=3) -> (element=w142:dbl)
            n63 = Index Array(array=w159, index=2) -> (element=→"Y满":bool)
            n64 = Divide(x=w142, y=10.0) -> (x/y=w140:dbl)
            n65 = Multiply(x=w140, y=10000.0) -> (x*y=w138:dbl)
            n66 = property on="LensHV-Real" class="DigNum (strict)"(error in=w173, "Value"=w138) -> (error out=w136:errorcluster)  [unwired: 1 in, 1 out]
            n67 = Index Array(array=w134, index=19) -> (element=w133:dbl)
            n68 = Subtract(x=w133, y=3.572) -> (x-y=w131:dbl)
            n69 = Divide(x=w131, y=1.286) -> (x/y=w129:dbl)
            n70 = Power Of 10(x=w129) -> (10^x=w128:dbl)
            n71 = Index Array(array=w134, index=18) -> (element=w127:dbl)
            n72 = Subtract(x=w127, y=8.5) -> (x-y=w125:dbl)
            n73 = property on="Lvaccum" class="DigNum (strict)"(error in=w136, "Value"=w128) -> (error out=w123:errorcluster)  [unwired: 1 in, 1 out]
            n74 = Power Of 10(x=w125) -> (10^x=w124:dbl)
            n75 = property on="Hvaccum" class="DigNum (strict)"(error in=w123, "Value"=w124) -> ()  [unwired: 1 in, 2 out]
          }
          event User Event {
            n76 = event-data() -> ("machine status"=w177:string)  [unwired: 1 in, 4 out]
            n77 = case shown="\"aquire start\", Default" w177 {
              frame "aquire start", Default {
              }
              frame "aquire stop" {
              }
            }
          }
          event "laser ON": Value Change {
            n78 = event-data() -> ("NewVal"=w181:bool)  [unwired: 1 in, 5 out]
            n79 = case shown="True" w181 {
              tunnel: w180 -> [w193 w210]
              tunnel: w179 -> [w192 w208]
              frame True {
                # "Repetition"
                n80 = Unbundle By Name(w192) -> ("ConfiguredLaserCom"=w189:refnum<visa-resource-name>)
                n81 = Unbundle By Name(w193) -> ("laser semaphore"=w184:T3)
                n82 = property on="cluster" class="Clust (strict)"() -> ("Value"=w191:T7)  [unwired: 2 in, 2 out]
                n83 = Unbundle By Name(w191) -> ("待机"=w190:bool)
                n84 = call <vilib>:"Acquire Semaphore.vi"("semaphore"=w184) -> ("error out"=w182:errorcluster, "semaphore out"=w183:T3)  [unwired: 4 in, 1 out]
                n85 = case shown="False" w190 {
                  tunnel: w189 -> [w198 w203]
                  tunnel: [w197 w203] -> w186
                  tunnel: [w195 w202] -> w185
                  tunnel: w182 -> [w194 w202]
                  frame False {
                    # "LaserOn"
                    n86 = VISA Write(VISA resource name=w198, write buffer="#!@gEB\r", error in (no error)=w194) -> (error out=w196:errorcluster)  [unwired: 2 out]
                    n87 = flat-sequence {
                      tunnel: w196 -> [w201]
                      tunnel: [w201] -> w195
                      tunnel: w198 -> [w200]
                      tunnel: [w200] -> w197
                      frame #0 {
                        n88 = call "Time Delay3"() -> ()  [unwired: 11 in, 1 out]
                      }
                    }
                  }
                  frame True {
                  }
                }
                n89 = VISA Write(VISA resource name=w186, write buffer="#!@hEC\r", error in (no error)=w185) -> (error out=w187:errorcluster)  [unwired: 2 out]
                n90 = call <vilib>:"Release Semaphore.vi"("error in (no error)"=w187, "semaphore"=w183) -> ()  [unwired: 4 in, 2 out]
              }
              frame False {
                n91 = Unbundle By Name(w210) -> ("laser semaphore"=w209:T3)
                n92 = Unbundle By Name(w208) -> ("ConfiguredLaserCom"=w207:refnum<visa-resource-name>)
                n93 = call <vilib>:"Acquire Semaphore.vi"("semaphore"=w209) -> ("error out"=w206:errorcluster, "semaphore out"=w204:T3)  [unwired: 4 in, 1 out]
                n94 = call "laserStop.vi"("error in (no error)"=w206, "VISA resource name"=w207) -> ("error out"=w205:errorcluster)  [unwired: 9 in]
                n95 = call <vilib>:"Release Semaphore.vi"("error in (no error)"=w205, "semaphore"=w204) -> ()  [unwired: 4 in, 2 out]
              }
            }
          }
          event "laser OFF": Value Change {
            n96 = event-data() -> ("NewVal"=w214:bool)  [unwired: 1 in, 5 out]
            n97 = case shown="True" w214 {
              tunnel: w213 -> [_ w221]
              tunnel: w212 -> [_ w219]
              frame False {
              }
              frame True {
                n98 = Unbundle By Name(w219) -> ("ConfiguredLaserCom"=w217:refnum<visa-resource-name>)
                n99 = Unbundle By Name(w221) -> ("laser semaphore"=w220:T3)
                n100 = call <vilib>:"Acquire Semaphore.vi"("semaphore"=w220) -> ("error out"=w216:errorcluster, "semaphore out"=w218:T3)  [unwired: 4 in, 1 out]
                n101 = call "Laser-Stop.vi"("error in (no error)"=w216, "VISA resource name"=w217) -> ("error out"=w215:errorcluster)
                n102 = call <vilib>:"Release Semaphore.vi"("error in (no error)"=w215, "semaphore"=w218) -> ()  [unwired: 4 in, 2 out]
              }
            }
          }
          event "StartPump": Value Change {
            n103 = event-data() -> ("NewVal"=w225:bool)  [unwired: 1 in, 5 out]
            n104 = case shown="True" w225 {
              tunnel: w224 -> [_ w230]
              tunnel: w223 -> [_ w229]
              frame False {
              }
              frame True {
                n105 = Unbundle By Name(w229) -> ("ConfiguredPumpCom"=w228:refnum<visa-resource-name>)
                n106 = Unbundle By Name(w230) -> ("laser semaphore"=w227:T3)
                n107 = call <vilib>:"Acquire Semaphore.vi"("semaphore"=w227) -> ("error out"=w232:errorcluster, "semaphore out"=w226:T3)  [unwired: 4 in, 1 out]
                n108 = call "pumpStart.vi"("error in (no error)"=w232, "VISA resource name"=w228) -> ("error out"=w231:errorcluster)  [unwired: 9 in]
                n109 = call <vilib>:"Release Semaphore.vi"("error in (no error)"=w231, "semaphore"=w226) -> ()  [unwired: 4 in, 2 out]
              }
            }
          }
          event "SopPump": Value Change {
            n110 = event-data() -> ("NewVal"=w236:bool)  [unwired: 1 in, 5 out]
            n111 = case shown="True" w236 {
              tunnel: w235 -> [_ w240]
              tunnel: w234 -> [_ w238]
              frame False {
              }
              frame True {
                n112 = Unbundle By Name(w240) -> ("pump semaphore"=w239:T3)
                n113 = Unbundle By Name(w238) -> ("ConfiguredPumpCom"=w237:refnum<visa-resource-name>)
                n114 = call <vilib>:"Acquire Semaphore.vi"("semaphore"=w239) -> ("error out"=w243:errorcluster, "semaphore out"=w241:T3)  [unwired: 4 in, 1 out]
                n115 = call "pumpStop.vi"("error in (no error)"=w243, "VISA resource name"=w237) -> ("error out"=w242:errorcluster)  [unwired: 9 in]
                n116 = call <vilib>:"Release Semaphore.vi"("error in (no error)"=w242, "semaphore"=w241) -> ()  [unwired: 4 in, 2 out]
              }
            }
          }
          event "HVEnable": Value Change {
            n117 = event-data() -> ("NewVal"=w245:bool)  [unwired: 1 in, 5 out]
            n118 = case shown="True" w245 {
              frame False {
                n119 = call "setDO.vi"("channel"=2, "on/off"=TRUE) -> ("错误输出"=w248:errorcluster)  [unwired: 9 in]
                n120 = call "setDO.vi"("错误输入（无错误）"=w248, "channel"=3, "on/off"=TRUE) -> ("错误输出"=w247:errorcluster)  [unwired: 8 in]
                n121 = call "setDO.vi"("错误输入（无错误）"=w247, "channel"=4, "on/off"=TRUE) -> ("错误输出"=w246:errorcluster)  [unwired: 8 in]
                n122 = call "setDO.vi"("错误输入（无错误）"=w246, "channel"=5, "on/off"=TRUE) -> ()  [unwired: 8 in, 1 out]
              }
              frame True {
                n123 = property on="MCPHV-Set" class="DigNum (strict)"() -> ("Value"=w281:dbl)  [unwired: 2 in, 2 out]
                n124 = Divide(x=w281, y=2000.0) -> (x/y=w283:dbl)
                n125 = Multiply(x=w283, y=10.0) -> (x*y=w274:dbl)
                n126 = Less?(x=w274, y=1.0) -> (x < y?=w275:bool)
                n127 = call "setDO.vi"("channel"=2, "on/off"=FALSE) -> ("错误输出"=w287:errorcluster)  [unwired: 9 in]
                n128 = case shown="False" w275 {
                  tunnel: w274 -> [w342 w350]
                  frame False {
                    n129 = while {
                      tunnel: w342 -> [w344]
                      tunnel: [w344] -> w340
                      i -> [w348]
                      stop <- w345 stop-if-true
                      n130 = Increment(x=w348) -> (x+1=w347:i32)
                      n131 = Increment(x=w347) -> (x+1=w346:i32)
                      n132 = call "setAO.vi"("value"=w347, "channel"=0) -> ()  [unwired: 9 in, 1 out]
                      n133 = Greater Or Equal?(x=w346, y=w344) -> (x >= y?=w345:bool)
                      n134 = Wait (ms)(milliseconds to wait=1000) -> ()  [unwired: 1 out]
                    }
                    n135 = call "setAO.vi"("value"=w340, "channel"=0) -> ()  [unwired: 9 in, 1 out]
                  }
                  frame True {
                    n136 = call "setAO.vi"("value"=w350, "channel"=0) -> ()  [unwired: 9 in, 1 out]
                  }
                }
                n137 = call "setDO.vi"("错误输入（无错误）"=w287, "channel"=3, "on/off"=FALSE) -> ("错误输出"=w286:errorcluster)  [unwired: 8 in]
                n138 = call "setDO.vi"("错误输入（无错误）"=w286, "channel"=4, "on/off"=FALSE) -> ("错误输出"=w285:errorcluster)  [unwired: 8 in]
                n139 = property on="Tar.HV-Set" class="DigNum (strict)"() -> ("Value"=w277:dbl)  [unwired: 2 in, 2 out]
                n140 = Divide(x=w277, y=20000.0) -> (x/y=w279:dbl)
                n141 = call "setDO.vi"("错误输入（无错误）"=w285, "channel"=5, "on/off"=FALSE) -> ()  [unwired: 8 in, 1 out]
                n142 = Multiply(x=w279, y=10.0) -> (x*y=w271:dbl)
                n143 = Less?(x=w271, y=0.5) -> (x < y?=w272:bool)
                n144 = case shown="False" w272 {
                  tunnel: w271 -> [w326 w338]
                  frame False {
                    n145 = while {
                      tunnel: w326 -> [w335]
                      tunnel: [w335] -> w324
                      i -> [w331]
                      stop <- w336 stop-if-true
                      n146 = Divide(x=w331, y=2.0) -> (x/y=w332:dbl)
                      n147 = Add(x=0.5, y=w332) -> (x+y=w329:dbl)
                      n148 = Add(x=w329, y=0.5) -> (x+y=w327:dbl)
                      n149 = call "setAO.vi"("value"=w329, "channel"=1) -> ()  [unwired: 9 in, 1 out]
                      n150 = Greater Or Equal?(x=w327, y=w335) -> (x >= y?=w336:bool)
                      n151 = Wait (ms)(milliseconds to wait=500) -> ()  [unwired: 1 out]
                    }
                    n152 = call "setAO.vi"("value"=w324, "channel"=1) -> ()  [unwired: 9 in, 1 out]
                  }
                  frame True {
                    n153 = call "setAO.vi"("value"=w338, "channel"=1) -> ()  [unwired: 9 in, 1 out]
                  }
                }
                n154 = property on="Pul.HV-Set" class="DigNum (strict)"() -> ("Value"=w270:dbl)  [unwired: 2 in, 2 out]
                n155 = Divide(x=w270, y=2000.0) -> (x/y=w265:dbl)
                n156 = Multiply(x=w265, y=10.0) -> (x*y=w269:dbl)
                n157 = Less?(x=w269, y=1.0) -> (x < y?=w268:bool)
                n158 = case shown="False" w268 {
                  tunnel: w269 -> [w314 w322]
                  frame False {
                    n159 = while {
                      tunnel: w314 -> [w316]
                      tunnel: [w316] -> w312
                      i -> [w320]
                      stop <- w317 stop-if-true
                      n160 = Increment(x=w320) -> (x+1=w319:i32)
                      n161 = Increment(x=w319) -> (x+1=w318:i32)
                      n162 = call "setAO.vi"("value"=w319, "channel"=2) -> ()  [unwired: 9 in, 1 out]
                      n163 = Greater Or Equal?(x=w318, y=w316) -> (x >= y?=w317:bool)
                      n164 = Wait (ms)(milliseconds to wait=1000) -> ()  [unwired: 1 out]
                    }
                    n165 = call "setAO.vi"("value"=w312, "channel"=2) -> ()  [unwired: 9 in, 1 out]
                  }
                  frame True {
                    n166 = call "setAO.vi"("value"=w322, "channel"=2) -> ()  [unwired: 9 in, 1 out]
                  }
                }
                n167 = property on="LensHV-Set" class="DigNum (strict)"() -> ("Value"=w263:dbl)  [unwired: 2 in, 2 out]
                n168 = Divide(x=w263, y=10000.0) -> (x/y=w258:dbl)
                n169 = Multiply(x=w258, y=10.0) -> (x*y=w262:dbl)
                n170 = Less?(x=w262, y=0.5) -> (x < y?=w261:bool)
                n171 = case shown="False" w261 {
                  tunnel: w262 -> [w298 w310]
                  frame False {
                    n172 = while {
                      tunnel: w298 -> [w307]
                      tunnel: [w307] -> w296
                      i -> [w303]
                      stop <- w308 stop-if-true
                      n173 = Divide(x=w303, y=2.0) -> (x/y=w304:dbl)
                      n174 = Add(x=0.5, y=w304) -> (x+y=w301:dbl)
                      n175 = Add(x=w301, y=0.5) -> (x+y=w299:dbl)
                      n176 = call "setAO.vi"("value"=w301, "channel"=3) -> ()  [unwired: 9 in, 1 out]
                      n177 = Greater Or Equal?(x=w299, y=w307) -> (x >= y?=w308:bool)
                      n178 = Wait (ms)(milliseconds to wait=500) -> ()  [unwired: 1 out]
                    }
                    n179 = call "setAO.vi"("value"=w296, "channel"=3) -> ()  [unwired: 9 in, 1 out]
                  }
                  frame True {
                    n180 = call "setAO.vi"("value"=w310, "channel"=3) -> ()  [unwired: 9 in, 1 out]
                  }
                }
              }
            }
          }
          event "Samp_Atmos": Value Change {
            n181 = event-data() -> ("OldVal"=w353:bool, "NewVal"=w357:bool)  [unwired: 1 in, 4 out]
            n182 = property on="Fore_Samp" class="Bool (strict)"() -> ("Value"=w356:bool)  [unwired: 2 in, 2 out]
            n183 = And(x=w357, y=w356) -> (x .and. y?=w355:bool)
            n184 = Not(x=w355) -> (.not. x?=w354:bool)
            n185 = case shown="True" w354 {
              tunnel: w357 -> [_ w360]
              tunnel: w353 -> [w359 _]
              frame False {
                n186 = property on="Samp_Atmos" class="Bool (strict)"("Value"=w359) -> (error out=w358:errorcluster)  [unwired: 2 in, 1 out]
                n187 = call "Display Message to User7"("error in (no error)"=w358) -> ()  [unwired: 9 in, 2 out]
              }
              frame True {
                n188 = case shown="False" w360 {
                  frame False {
                    n189 = call "setDO.vi"("channel"=6, "on/off"=FALSE) -> ()  [unwired: 9 in, 1 out]
                  }
                  frame True {
                    n190 = property on="Y满" class="Bool (strict)"() -> ("Value"=w364:bool)  [unwired: 2 in, 2 out]
                    n191 = Not(x=w364) -> (.not. x?=w363:bool)
                    n192 = case shown="False" w363 {
                      frame False {
                        n193 = call "setDO.vi"("channel"=6, "on/off"=TRUE) -> ()  [unwired: 9 in, 1 out]
                      }
                      frame True {
                        n194 = call "Display Message to User6"() -> ()  [unwired: 10 in, 2 out]
                      }
                    }
                  }
                }
              }
            }
          }
          event "Fore_Samp": Value Change {
            n195 = event-data() -> ("OldVal"=w368:bool, "NewVal"=w372:bool)  [unwired: 1 in, 4 out]
            n196 = property on="Samp_Atmos" class="Bool (strict)"() -> ("Value"=w371:bool)  [unwired: 2 in, 2 out]
            n197 = And(x=w372, y=w371) -> (x .and. y?=w370:bool)
            n198 = Not(x=w370) -> (.not. x?=w369:bool)
            n199 = case shown="True" w369 {
              tunnel: w372 -> [_ w375]
              tunnel: w368 -> [w374 _]
              frame False {
                n200 = property on="Fore_Samp" class="Bool (strict)"("Value"=w374) -> (error out=w373:errorcluster)  [unwired: 2 in, 1 out]
                n201 = call "Display Message to User8"("error in (no error)"=w373) -> ()  [unwired: 9 in, 2 out]
              }
              frame True {
                n202 = case shown="True" w375 {
                  frame False {
                    n203 = call "setDO.vi"("channel"=7, "on/off"=FALSE) -> ()  [unwired: 9 in, 1 out]
                  }
                  frame True {
                    n204 = property on="Y满" class="Bool (strict)"() -> ("Value"=w379:bool)  [unwired: 2 in, 2 out]
                    n205 = Not(x=w379) -> (.not. x?=w378:bool)
                    n206 = case shown="True" w378 {
                      frame False {
                        n207 = call "setDO.vi"("channel"=7, "on/off"=TRUE) -> ()  [unwired: 9 in, 1 out]
                      }
                      frame True {
                        n208 = call "Display Message to User"() -> ()  [unwired: 10 in, 2 out]
                      }
                    }
                  }
                }
              }
            }
          }
          event "MCPHV-Set": Value Change {
            n209 = event-data() -> ("NewVal"=w383:dbl)  [unwired: 1 in, 5 out]
            n210 = Divide(x=w383, y=2000.0) -> (x/y=w386:dbl)
            n211 = Multiply(x=w386, y=10.0) -> (x*y=w384:dbl)
            n212 = call "setAO.vi"("value"=w384, "channel"=0) -> ()  [unwired: 9 in, 1 out]
          }
          event "Tar.HV-Set": Value Change {
            n213 = event-data() -> ("NewVal"=w395:dbl)  [unwired: 1 in, 5 out]
            n214 = Divide(x=w395, y=20000.0) -> (x/y=w392:dbl)
            n215 = Multiply(x=w392, y=10.0) -> (x*y=w390:dbl)
            n216 = call "setAO.vi"("value"=w390, "channel"=1) -> ()  [unwired: 9 in, 1 out]
          }
          event "Pul.HV-Set": Value Change {
            n217 = event-data() -> ("NewVal"=w402:dbl)  [unwired: 1 in, 5 out]
            n218 = Divide(x=w402, y=2000.0) -> (x/y=w399:dbl)
            n219 = Multiply(x=w399, y=10.0) -> (x*y=w397:dbl)
            n220 = call "setAO.vi"("value"=w397, "channel"=2) -> ()  [unwired: 9 in, 1 out]
          }
          event "LensHV-Set": Value Change {
            n221 = event-data() -> ("NewVal"=w409:dbl)  [unwired: 1 in, 5 out]
            n222 = Divide(x=w409, y=10000.0) -> (x/y=w406:dbl)
            n223 = Multiply(x=w406, y=10.0) -> (x*y=w405:dbl)
            n224 = call "setAO.vi"("value"=w405, "channel"=3) -> ()  [unwired: 9 in, 1 out]
          }
          event User Event {
            n225 = event-data() -> ("status"=w411:string)  [unwired: 1 in, 5 out]
            n226 = case shown="\"stop\", Default" w411 {
              frame "stop", Default {
                n227 = property on="GO" class="Bool (strict)"("DisabledEnum"=T10."Enabled" ("Disabled")) -> (error out=w413:errorcluster)  [unwired: 2 in, 1 out]
                n228 = property on="移动" class="Bool (strict)"(error in=w413, "Value"=FALSE ("移动")) -> ()  [unwired: 1 in, 2 out]
              }
              frame "moving" {
                n229 = property on="GO" class="Bool (strict)"("DisabledEnum"=T10."Disabled and Grayed Out" ("Disabled")) -> (error out=w416:errorcluster)  [unwired: 2 in, 1 out]
                n230 = property on="移动" class="Bool (strict)"(error in=w416, "Value"=TRUE ("移动")) -> ()  [unwired: 1 in, 2 out]
              }
            }
          }
          event User Event {
            n231 = event-data() -> ("source"=w426:string, "value"=w425:dbl)  [unwired: 1 in, 4 out]
            n232 = case shown="\"X\"" w426 {
              tunnel: w425 -> [w427 w435]
              tunnel: [w429 w436] -> w419
              frame "Y", Default {
                n233 = property on="X当前" class="DigNum (strict)"() -> ("Value"=w431:dbl)  [unwired: 2 in, 2 out]
                n234 = Multiply(x=w427, y=1000.0) -> (x*y=w432:dbl)
                n235 = Divide(x=w431, y=1000.0) -> (x/y=w428:dbl)
                n236 = Build Array "Build Array"(w428, w427) -> (w429:dbl[])
                n237 = property on="Y当前" class="DigNum (strict)"("Value"=w432) -> ()  [unwired: 2 in, 2 out]
              }
              frame "X" {
                n238 = property on="Y当前" class="DigNum (strict)"() -> ("Value"=w438:dbl)  [unwired: 2 in, 2 out]
                n239 = Multiply(x=w435, y=1000.0) -> (x*y=w439:dbl)
                n240 = Divide(x=w438, y=1000.0) -> (x/y=w434:dbl)
                n241 = property on="X当前" class="DigNum (strict)"("Value"=w439) -> ()  [unwired: 2 in, 2 out]
                n242 = Build Array(w435, w434) -> (w436:dbl[])
              }
            }
            n243 = Current VI's Path() -> (path=w422:path)
            n244 = Strip Path(path=w422) -> (stripped path=w421:path)  [unwired: 1 out]
            n245 = Build Path(base path=w421, name or relative path="last_position") -> (appended path=w423:path)
            n246 = call-poly <vilib>:"Write To Spreadsheet File.vi"("format (%.3f)"="%.9f", "1D data"=w419, "file path (dialog if empty)"=w423) -> ()  [unwired: 5 in, 1 out]
          }
          event "Image": Mouse Down {
            n247 = event-data() -> ("Coords"=w441:T16)  [unwired: 1 in, 7 out]
            n248 = property on="移动" class="Bool (strict)"() -> ("Value"=w442:bool)  [unwired: 2 in, 2 out]
            n249 = case shown="False" w442 {
              tunnel: w441 -> [w453 _]
              frame False {
                w450 = -0.008 ("x")
                n250 = Unbundle(w453) -> ("Horizontal"=w452:i32, "Vertical"=w451:i32)
                n251 = property on="X当前" class="DigNum (strict)"() -> ("Value"=w449:dbl)  [unwired: 2 in, 2 out]
                n252 = property on="Y当前" class="DigNum (strict)"() -> ("Value"=w445:dbl)  [unwired: 2 in, 2 out]
                n253 = Subtract(x=w452, y=210.0) -> (x-y=w455:dbl)
                n254 = Subtract(x=w451, y=198.0) -> (x-y=w454:dbl)
                n255 = Multiply(x=w450, y=w455) -> (x*y=w448:dbl)
                n256 = Multiply(x=w450, y=w454) -> (x*y=w446:dbl)
                n257 = Add(x=w449, y=w448) -> (x+y=w447:dbl)
                n258 = Add(x=w446, y=w445) -> (x+y=w444:dbl)
                n259 = call "goto.vi"("Y(mm)"=w444, "X(mm)"=w447) -> ()  [unwired: 9 in, 1 out]
              }
              frame True {
              }
            }
          }
          event "TakeMS-Run": Value Change {
            n260 = event-data() -> ("NewVal"=w463:bool)  [unwired: 1 in, 5 out]
            n261 = case shown="True" w463 {
              tunnel: w462 -> [_ w479]
              tunnel: w461 -> [_ w476]
              tunnel: w460 -> [_ w475]
              tunnel: w459 -> [w464 w466]
              tunnel: [w464 w465] -> w458
              frame False {
              }
              frame True {
                n262 = Unbundle By Name(w475) -> ("ConfiguredLaserCom"=w472:refnum<visa-resource-name>)
                n263 = Unbundle By Name(w476) -> ("laser semaphore"=w470:T3)
                n264 = property on="cluster" class="Clust (strict)"() -> ("Value"=w474:T7)  [unwired: 2 in, 2 out]
                n265 = Bundle By Name(cluster=w479, "ShotsPerPoint"="Shots/Point") -> (w477:T5)
                n266 = Unbundle By Name(w474) -> ("待机"=w471:bool)
                n267 = property on="SetLaserEnergy" class="Slide (strict)"() -> ("Value"=w469:dbl)  [unwired: 2 in, 2 out]
                n268 = Bundle By Name(cluster="Laser parameter", "VISA resource name"=w472, "standby"=w471, "semaphore in"=w470, "SetLaserEnergy"=w469) -> (w468:T4)
                n269 = case shown="0, Default" "AcquireMS-Methods" {
                  tunnel: w477 -> [w499 _ _]
                  tunnel: w468 -> [w500 _ _]
                  tunnel: w466 -> [w498 w509 w510]
                  tunnel: [w489 w509 w510] -> w465
                  frame 0, Default {
                    n270 = Get Date/Time String() -> (date string=w496:string, time string=w495:string)  [unwired: 3 in]
                    n271 = Concatenate Strings(w496, " " ("字符串"), w495) -> (w490:string)
                    n272 = call "Tiepie-takeData-2018-06-01.vi"("left rank"="left rank", "right rank"="right rank", "deBaseline"="deBaseline", "Thresh"="Thresh", "Laser parameter"=w500, "ADC parameter"=w499) -> ("output cluster"=w481:cluster{dbl[], "filtered data":dbl[]})  [unwired: 1 in, 1 out]
                    "MS" <- w481
                    n273 = Unbundle(w481) -> (w482:dbl[], "filtered data"=w497:dbl[])
                    n274 = property on="currentNO" class="Str"() -> ("Value"=w492:string)  [unwired: 2 in, 2 out]
                    n275 = Bundle By Name(cluster=T11 {"tag1"="", "tag2"="", "x"=[], "y"=[], "ID1:X"=[], "ID1:Y"=[], "ID1:REF:X"=[], "ID1:REF:Y"=[], "ID2:X"=[], "ID2:Y"=[], "ID2:REF:X"=[], "ID2:REF:Y"=[], "ID3:X"=[], "ID3:Y"=[], "ID3:REF:X"=[], "ID3:REF:Y"=[], "ID1:TAG1"="", "ID1:TAG2"="", "ID2:TAG1"="", "ID2:TAG2"="", "ID3:TAG1"="", "ID3:TAG2"="", "ID1:NAME"="", "ID2:NAME"="", "ID3:NAME"="", "ID1:SCORE"="", "ID2:SCORE"="", "ID3:SCORE"="", "NO"=""}, "y"=w497, "x"=w482, "tag1"="未鉴定", "tag2"=w490, "NO"=w492) -> (w491:T11)
                    n276 = Build Array (concatenate)(w498, w491) -> (w489:T8)
                    n277 = for {
                      tunnel: w489 -> [w508] mode=indexing
                      shift-right: [w501] -> w487
                      shift-left: string[][] [] ("Item Names") -> [w503]
                      i -> [w504]
                      n278 = Unbundle By Name(w508) -> ("NO"=w507:string, "tag1"=w506:string, "tag2"=w505:string)
                      n279 = Build Array(w507, w506, w505) -> (w502:string[])
                      n280 = Insert Into Array "Insert Into Array"(array=w503, index (row)=w504, new element=w502) -> (w501:string[][])  [unwired: 1 in]
                    }
                    n281 = property on="测试记录" class="MCListbox (strict)"("ItemNames"=w487) -> ()  [unwired: 2 in, 2 out]
                  }
                  frame 1 {
                  }
                  frame 2 {
                  }
                }
              }
            }
          }
          event "Set Laser": Value Change {
            n282 = event-data() -> ("NewVal"=w513:bool)  [unwired: 1 in, 5 out]
            n283 = case shown="True" w513 {
              tunnel: w512 -> [_ w521]
              tunnel: w511 -> [_ w516]
              frame False {
              }
              frame True {
                n284 = Unbundle By Name(w516) -> ("ConfiguredLaserCom"=w515:refnum<visa-resource-name>)
                n285 = Unbundle By Name(w521) -> ("laser semaphore"=w520:T3)
                n286 = call <vilib>:"Acquire Semaphore.vi"("semaphore"=w520) -> ("error out"=w519:errorcluster, "semaphore out"=w517:T3)  [unwired: 4 in, 1 out]
                n287 = call "Laser-Set-Parmeter.vi"("error in (no error)"=w519, "LaserHV"="LaserHV", "LaserFreq"="频率/Hz", "SetLaserEnergy"="SetLaserEnergy", "VISA resource name"=w515) -> ("error out"=w518:errorcluster)  [unwired: 1 in, 1 out]
                n288 = call <vilib>:"Release Semaphore.vi"("error in (no error)"=w518, "semaphore"=w517) -> ()  [unwired: 4 in, 2 out]
              }
            }
          }
          event "测试记录": Shortcut Menu Selection (User) {
            n289 = event-data() -> ("ItemTag"=w527:string)  [unwired: 1 in, 7 out]
            n290 = case shown="\"鉴定\"" w527 {
              tunnel: w526 -> [w528 w535 w542 w547]
              tunnel: [w528 w535 w542 w543] -> w525
              frame "假", Default {
              }
              frame "鉴定" {
                n291 = property on="selected row" class="DigNum (strict)"() -> ("Value"=w531:i32)  [unwired: 2 in, 2 out]
                n292 = Index Array(array=w535, index=w531) -> (element=w541:T11)
                n293 = Unbundle By Name(w541) -> ("x"=w540:dbl[], "y"=w536:dbl[])
                n294 = call-poly <userlib>:"CaLabPut.vi"("Values"=w540, "PV Names"="MS:X") -> ("Error out"=w538:errorcluster)  [unwired: 6 in, 3 out]
                n295 = call-poly <userlib>:"CaLabPut.vi"("Error in (no error)"=w538, "Values"=w536, "PV Names"="MS:Y") -> ("Error out"=w534:errorcluster)  [unwired: 5 in, 3 out]
                n296 = call-poly <userlib>:"CaLabPut.vi"("Error in (no error)"=w534, "Value"=w531, "PV Name"="MS:NUM") -> ("Error out"=w533:errorcluster)  [unwired: 5 in, 3 out]
                n297 = call-poly <userlib>:"CaLabPut.vi"("Error in (no error)"=w533, "Value"=1, "PV Name"="MS:START") -> ()  [unwired: 5 in, 4 out]
              }
              frame "参数" {
              }
              frame "删除" {
                n298 = property on="selected row" class="DigNum (strict)"() -> ("Value"=w546:i32)  [unwired: 2 in, 2 out]
                n299 = Delete From Array "Delete From Array"(array=w547, index=w546) -> (array with subset deleted=w543:T8)  [unwired: 1 in, 1 out]
                n300 = for {
                  tunnel: w543 -> [w555] mode=indexing
                  shift-right: [w548] -> w544
                  shift-left: string[][] [] ("Item Names") -> [w550]
                  i -> [w551]
                  n301 = Unbundle By Name(w555) -> ("NO"=w554:string, "tag1"=w553:string, "tag2"=w552:string)
                  n302 = Build Array(w554, w553, w552) -> (w549:string[])
                  n303 = Insert Into Array "Insert Into Array"(array=w550, index (row)=w551, new element=w549) -> (w548:string[][])  [unwired: 1 in]
                }
                n304 = property on="测试记录" class="MCListbox (strict)"("ItemNames"=w544) -> ()  [unwired: 2 in, 2 out]
              }
            }
          }
          event "测试记录": Mouse Down {
            n305 = event-data() -> ("Coords"=w561:T16)  [unwired: 1 in, 7 out]
            n306 = invoke on="测试记录" class="MCListbox (严格)" method="Point To Row Column"("Point"=w561) -> ("CellPosition"=w560:T17)  [unwired: 6 in, 6 out]
            n307 = Unbundle By Name(w560) -> ("Row"=w557:i32)
            n308 = Array Size(array=w556) -> (size(s)=w559:i32)
            n309 = Greater Or Equal?(x=w559, y=w557) -> (x >= y?=w558:bool)
            n310 = case shown="True" w558 {
              tunnel: w557 -> [_ w588]
              tunnel: w556 -> [_ w589]
              frame False {
              }
              frame True {
                n311 = property on="selected row" class="DigNum (strict)"("Value"=w588) -> ()  [unwired: 2 in, 2 out]
                n312 = Index Array(array=w589, index=w588) -> (element=w587:T11)
                n313 = Unbundle By Name(w587) -> ("ID1:TAG1"=w570:string, "ID1:TAG2"=w584:string, "ID1:NAME"=w583:string, "ID1:SCORE"=w574:string, "ID2:TAG1"=w568:string, "ID2:TAG2"=w581:string, "ID2:NAME"=w580:string, "ID2:SCORE"=w573:string, "ID3:TAG1"=w566:string, "ID3:TAG2"=w565:string, "ID3:NAME"=w564:string, "ID3:SCORE"=w563:string)
                n314 = Build Array("1" ("element"), w570, w584, w583, w574) -> (w582:string[])
                n315 = Build Array("2" ("element"), w568, w581, w580, w573) -> (w577:string[])
                n316 = Build Array("3" ("element"), w566, w565, w564, w563) -> (w572:string[])
                n317 = Insert Into Array(array=string[][] [] ("项名"), index (row)=0 ("索引 (行)"), new element=w582) -> (w579:string[][])  [unwired: 1 in]
                n318 = Insert Into Array(array=w579, index (row)=1 ("索引 (行)"), new element=w577) -> (w576:string[][])  [unwired: 1 in]
                n319 = Insert Into Array(array=w576, index (row)=2 ("索引 (行)"), new element=w572) -> (w571:string[][])  [unwired: 1 in]
                n320 = property on="Identification Results (单靶鉴定结果)" class="MCListbox (strict)"("ItemNames"=w571) -> ()  [unwired: 2 in, 2 out]
              }
            }
          }
          event "Identification Results (单靶鉴定结果)": Mouse Down {
            n321 = event-data() -> ("Coords"=w595:T16)  [unwired: 1 in, 7 out]
            n322 = invoke on="Identification Results (单靶鉴定结果)" class="MCListbox (严格)" method="Point To Row Column"("Point"=w595) -> ("CellPosition"=w594:T17)  [unwired: 6 in, 6 out]
            n323 = Unbundle By Name(w594) -> ("Row"=w590:i32)
            n324 = Less Or Equal?(x=w590, y=2) -> (x <= y?=w592:bool)
            n325 = case shown="True" w592 {
              tunnel: w591 -> [_ w602]
              tunnel: w590 -> [_ w596]
              frame False {
              }
              frame True {
                n326 = property on="selected row" class="DigNum (strict)"() -> ("Value"=w601:i32)  [unwired: 2 in, 2 out]
                n327 = Index Array(array=w602, index=w601) -> (element=w600:T11)
                n328 = case shown="2" w596 {
                  tunnel: w600 -> [w608 w620 w629]
                  tunnel: [w607 w616 w625] -> w599
                  tunnel: [w606 w615 w624] -> w597
                  frame 0, Default {
                    n329 = Unbundle By Name(w608) -> ("x"=w610:dbl[], "y"=w609:dbl[], "ID1:REF:X"=w611:dbl[], "ID1:REF:Y"=w605:dbl[])
                    n330 = Multiply(x=w605, y=-1.0) -> (x*y=w603:dbl[])
                    n331 = Bundle("x"=w610, "y"=w609) -> (w607:cluster{"x":dbl[], "y":dbl[]})  [unwired: 1 in]
                    n332 = Bundle("ID1:REF:X"=w611, w603) -> (w606:cluster{"ID1:REF:X":dbl[], dbl[]})  [unwired: 1 in]
                  }
                  frame 1 {
                    n333 = Unbundle By Name(w620) -> ("x"=w618:dbl[], "y"=w617:dbl[], "ID2:REF:X"=w619:dbl[], "ID2:REF:Y"=w614:dbl[])
                    n334 = Multiply(x=w614, y=-1.0) -> (x*y=w612:dbl[])
                    n335 = Bundle("x"=w618, "y"=w617) -> (w616:cluster{"x":dbl[], "y":dbl[]})  [unwired: 1 in]
                    n336 = Bundle("ID2:REF:X"=w619, w612) -> (w615:cluster{"ID2:REF:X":dbl[], dbl[]})  [unwired: 1 in]
                  }
                  frame 2 {
                    n337 = Unbundle By Name(w629) -> ("x"=w627:dbl[], "y"=w626:dbl[], "ID3:REF:X"=w628:dbl[], "ID3:REF:Y"=w623:dbl[])
                    n338 = Multiply(x=w623, y=-1.0) -> (x*y=w621:dbl[])
                    n339 = Bundle("x"=w627, "y"=w626) -> (w625:cluster{"x":dbl[], "y":dbl[]})  [unwired: 1 in]
                    n340 = Bundle("ID3:REF:X"=w628, w621) -> (w624:cluster{"ID3:REF:X":dbl[], dbl[]})  [unwired: 1 in]
                  }
                }
                n341 = Build Array(w599, w597) -> (→"Identify Spcetrum":cluster{"ID3:REF:X":dbl[], "y":dbl[]}[])
              }
            }
          }
          event "Plat_To_Zero": Value Change {
            n342 = event-data() -> ("NewVal"=w631:bool)  [unwired: 1 in, 5 out]
            n343 = case shown="True" w631 {
              frame False {
              }
              frame True {
                (unwired) TRUE ("plat zeroed")
                n344 = call "plate_cal.vi"() -> ()  [unwired: 11 in, 1 out]
              }
            }
          }
          event "GO": Value Change {
            n345 = event-data() -> ("NewVal"=w634:bool)  [unwired: 1 in, 5 out]
            n346 = property on="移动" class="Bool (strict)"() -> ("Value"=w636:bool)  [unwired: 2 in, 2 out]
            n347 = Not(x=w636) -> (.not. x?=w635:bool)
            n348 = And(x=w635, y=w634) -> (x .and. y?=w633:bool)
            n349 = case shown="True" w633 {
              frame False {
              }
              frame True {
                n350 = property on="X" class="DigNum (strict)"() -> (error out=w641:errorcluster, "Value"=w639:dbl)  [unwired: 2 in, 1 out]
                n351 = property on="Y" class="DigNum (strict)"(error in=w641) -> (error out=w640:errorcluster, "Value"=w638:dbl)  [unwired: 1 in, 1 out]
                n352 = vi-ref "goto.vi"() -> (w645:refnum<vi>)
                n353 = property class="VI"(reference=w645, error in=w640) -> ("Name"=w644:string)  [unwired: 2 out]
                n354 = Open VI Reference(type specifier VI Refnum (for type only)=refnum<vi> refnum, vi path=w644, options=128) -> (vi reference=w642:refnum<vi>)  [unwired: 3 in, 1 out]
                n355 = call-by-ref "Start Asynchronous Call"(reference=w642, "Y(mm)"=w638, "X(mm)"=w639) -> ()  [unwired: 10 in, 3 out]
              }
            }
          }
          event "chamber in": Value Change {
            n356 = event-data() -> ("NewVal"=w648:bool)  [unwired: 1 in, 5 out]
            n357 = property on="HVEnable" class="Bool (strict)"() -> ("Value"=w653:bool)  [unwired: 2 in, 2 out]
            n358 = property on="Y满" class="Bool (strict)"() -> ("Value"=w649:bool)  [unwired: 2 in, 2 out]
            n359 = property on="移动" class="Bool (strict)"() -> ("Value"=w652:bool)  [unwired: 2 in, 2 out]
            n360 = Not(x=w653) -> (.not. x?=w650:bool)
            n361 = Not(x=w652) -> (.not. x?=w651:bool)
            n362 = Compound Arithmetic op=AND(w650, w649, w651, w648) -> (w647:bool)
            n363 = case shown="True" w647 {
              frame False {
              }
              frame True {
                n364 = flat-sequence {
                  tunnel: [w658] -> w654
                  tunnel: w654 -> [w674]
                  frame #0 {
                    n365 = call "样品标识与备注"() -> ("备注"=w655:string, "样品名称"=w656:string)  [unwired: 16 in, 2 out]
                    n366 = property on="sampleID" class="Str"("Value"=w656) -> ()  [unwired: 2 in, 2 out]
                    n367 = property on="commet" class="Str"("Value"=w655) -> ()  [unwired: 2 in, 2 out]
                  }
                  frame #1 {
                    w659 = FALSE ("on/off")
                    # "关样仓/大气"
                    n368 = Wait (ms)(milliseconds to wait=1500) -> ()  [unwired: 1 out]
                    n369 = call "setDO.vi"("channel"=6, "on/off"=w659) -> ("错误输出"=w657:errorcluster)  [unwired: 9 in]
                    n370 = property on="Samp_Atmos" class="Bool (strict)"(error in=w657, "Value"=w659) -> (error out=w658:errorcluster)  [unwired: 1 in, 1 out]
                  }
                  frame #2 {
                    # "开前泵/样仓"
                    n371 = call "setDO.vi"("错误输入（无错误）"=w674, "channel"=7, "on/off"=TRUE) -> ("错误输出"=w673:errorcluster)  [unwired: 8 in]
                    n372 = flat-sequence {
                      tunnel: w673 -> [w684]
                      tunnel: [w684] -> w669
                      frame #0 {
                        n373 = Wait (ms)(milliseconds to wait=10000) -> ()  [unwired: 1 out]
                      }
                    }
                    n374 = call "getAI.vi"("错误输入（无错误）"=w669, "channel"=19) -> ("错误输出"=w668:errorcluster, "result"=w663:dbl)  [unwired: 8 in]
                    n375 = Subtract(x=w663, y=3.572) -> (x-y=w666:dbl)
                    n376 = Divide(x=w666, y=1.286) -> (x/y=w664:dbl)
                    n377 = Power Of 10(x=w664) -> (10^x=w662:dbl)
                    n378 = Less?(x=w662, y=10) -> (x < y?=w671:bool)
                    n379 = case shown="True" w671 {
                      tunnel: w668 -> [w678 w680]
                      frame False {
                        (unwired) 7
                        n380 = call "setDO.vi"("错误输入（无错误）"=w678, "on/off"=FALSE) -> ("错误输出"=w677:errorcluster)  [unwired: 9 in]
                        n381 = call "Display Message to User4"("error in (no error)"=w677) -> ()  [unwired: 9 in, 2 out]
                      }
                      frame True {
                        n382 = flat-sequence {
                          tunnel: w680 -> [w681]
                          frame #0 {
                            n383 = call "setDO.vi"("错误输入（无错误）"=w681, "channel"=7, "on/off"=FALSE) -> ()  [unwired: 8 in, 1 out]
                          }
                          frame #1 {
                            n384 = call "chamber_in.vi"() -> ()  [unwired: 12 in]
                          }
                        }
                      }
                    }
                  }
                }
              }
            }
          }
          event "chamber out": Value Change {
            n385 = event-data() -> ("NewVal"=w689:bool)  [unwired: 1 in, 5 out]
            n386 = property on="Y满" class="Bool (strict)"() -> ("Value"=w693:bool)  [unwired: 2 in, 2 out]
            n387 = property on="移动" class="Bool (strict)"() -> ("Value"=w692:bool)  [unwired: 2 in, 2 out]
            n388 = property on="HVEnable" class="Bool (strict)"() -> ("Value"=w694:bool)  [unwired: 2 in, 2 out]
            n389 = Not(x=w694) -> (.not. x?=w687:bool)
            n390 = Not(x=w692) -> (.not. x?=w690:bool)
            n391 = Not(x=w693) -> (.not. x?=w691:bool)
            n392 = Compound Arithmetic op=AND(w687, w691, w690, w689) -> (w688:bool)
            n393 = case shown="True" w688 {
              frame False {
                n394 = call "Display Message to User3"() -> ()  [unwired: 10 in, 2 out]
              }
              frame True {
                n395 = flat-sequence {
                  tunnel: [w698] -> w696
                  tunnel: w696 -> [w705]
                  tunnel: [w706] -> w695
                  tunnel: w695 -> [w714]
                  frame #0 {
                    n396 = call "chamber_out.vi"() -> ()  [unwired: 12 in]
                  }
                  frame #1 {
                    w699 = FALSE ("on/off")
                    # "关前泵/样仓"
                    n397 = Wait (ms)(milliseconds to wait=1500) -> ()  [unwired: 1 out]
                    n398 = call "setDO.vi"("channel"=7, "on/off"=w699) -> ("错误输出"=w697:errorcluster)  [unwired: 9 in]
                    n399 = property on="Fore_Samp" class="Bool (strict)"(error in=w697, "Value"=w699) -> (error out=w698:errorcluster)  [unwired: 1 in, 1 out]
                  }
                  frame #2 {
                    # "开样仓/大气"
                    n400 = call "getDI.vi"("错误输入（无错误）"=w705, "channel"=2) -> ("错误输出"=w702:errorcluster, "result"=w703:bool)  [unwired: 8 in]
                    n401 = Wait (ms)(milliseconds to wait=3000) -> ()  [unwired: 1 out]
                    n402 = case shown="False" w703 {
                      tunnel: w702 -> [w709 w711]
                      tunnel: [w708 w710] -> w706
                      frame False {
                        n403 = call "Display Message to User2"("error in (no error)"=w709) -> ("error out"=w708:errorcluster)  [unwired: 9 in, 1 out]
                      }
                      frame True {
                        n404 = call "setDO.vi"("错误输入（无错误）"=w711, "channel"=6, "on/off"=TRUE) -> ("错误输出"=w710:errorcluster)  [unwired: 8 in]
                      }
                    }
                  }
                  frame #3 {
                    n405 = call "setDO.vi"("错误输入（无错误）"=w714, "channel"=6, "on/off"=FALSE) -> ()  [unwired: 8 in, 1 out]
                  }
                }
              }
            }
          }
          event "标准样品": Value Change {
            n406 = event-data() -> ("NewVal"=w718:u16)  [unwired: 1 in, 5 out]
            n407 = control-ref of="定标参数"() -> (w719:refnum<vi>)
            n408 = local read "std sample"() -> (w717:T1)
            n409 = call "writetable.vi"("std sample"=w717, "type"=w718, "reference"=w719) -> ()  [unwired: 9 in]
          }
          event "peak cal": Value Change {
            n410 = event-data() -> ("NewVal"=w721:bool)  [unwired: 1 in, 5 out]
            n411 = case shown="True" w721 {
              frame False {
              }
              frame True {
                n412 = property on="定标参数" class="MCListbox (strict)"() -> ("ItemNames"=w741:string[][])  [unwired: 2 in, 2 out]
                n413 = Index Array(array=w741, index (col)=1 ("disabled index (col)")) -> (element=w742:string[])  [unwired: 1 in]
                n414 = Index Array(array=w741, index (col)=3 ("disabled index (col)")) -> (element=w739:string[])  [unwired: 1 in]
                n415 = Fract/Exp String To Number(string=w742) -> (number=w731:dbl[])  [unwired: 3 in, 1 out]
                n416 = Fract/Exp String To Number(string=w739) -> (number=w733:dbl[])  [unwired: 3 in, 1 out]
                n417 = call <vilib>:"General Polynomial Fit.vi"("Y"=w731, "polynomial order"=2, "X"=w733) -> ("Polynomial Coefficients"=w735:dbl[])  [unwired: 9 in, 3 out]
                n418 = Index Array(array=w735, index=2) -> (element=w723:dbl)
                "a:" <- w723
                n419 = Index Array(array=w735, index=1) -> (element=w724:dbl)
                "b:" <- w724
                n420 = Index Array(array=w735, index=0) -> (element=w725:dbl)
                "c:" <- w725
                n421 = global write "cal_p.vi" "a"(w723) -> ()
                n422 = global write "cal_p.vi" "b"(w724) -> ()
                n423 = for {
                  tunnel: w733 -> [w756] mode=indexing
                  tunnel: [w760] -> w732 mode=indexing
                  tunnel: w725 -> [w757]
                  tunnel: w724 -> [w758]
                  tunnel: w723 -> [w759]
                  n424 = formula code="m=a*x*x+b*x+c;"("a"=w759, "b"=w758, "c"=w757, "x"=w756) -> ("m"=w760:dbl)
                }
                n425 = global write "cal_p.vi" "c"(w725) -> ()
                n426 = for {
                  tunnel: w732 -> [w754] mode=indexing
                  tunnel: w731 -> [w755] mode=indexing
                  tunnel: [w753] -> w726 mode=indexing
                  n427 = formula code="delta=100*(m-m0)/m0;"("m0"=w755, "m"=w754) -> ("delta"=w753:dbl)
                }
                n428 = control-ref of="定标参数"() -> (w730:refnum<vi>)
                n429 = property on="Property Node" class="MCListbox (strict)"(reference=w730) -> (reference out=w729:refnum<vi>, "ItemNames"=w728:string[][])  [unwired: 1 in, 1 out]
                n430 = for {
                  shift-right: [w749] -> w727
                  shift-left: w728 -> [w752]
                  tunnel: w726 -> [w750] mode=indexing
                  i -> [w751]
                  n431 = Number To Fractional String(number=w750, precision (6)=i16 2) -> (F-format string=w747:string)  [unwired: 2 in]
                  n432 = Concatenate Strings(w747, "%" ("string")) -> (w745:string)
                  n433 = Replace Array Subset(array=w752, new element=w745, index (row)=w751, index (col)=4 ("disabled index (col)")) -> (w749:string[][])
                }
                n434 = property on="Property Node" class="MCListbox (strict)"(reference=w729, "ItemNames"=w727) -> ()  [unwired: 1 in, 2 out]
              }
            }
          }
          event "A1-Position": Value Change {
            n435 = event-data() -> ("NewVal"=w762:bool)  [unwired: 1 in, 5 out]
            n436 = case shown="True" w762 {
              frame False {
              }
              frame True {
                n437 = property on="X当前" class="DigNum (strict)"() -> ("Value"=→"A1-position-X":dbl)  [unwired: 2 in, 2 out]
                n438 = property on="Y当前" class="DigNum (strict)"() -> ("Value"=→"A1-position-Y":dbl)  [unwired: 2 in, 2 out]
              }
            }
          }
          event "A1": Value Change {
            n439 = event-data() -> ("NewVal"=w768:bool)  [unwired: 1 in, 5 out]
            n440 = property on="移动" class="Bool (strict)"() -> ("Value"=w770:bool)  [unwired: 2 in, 2 out]
            n441 = Not(x=w770) -> (.not. x?=w769:bool)
            n442 = And(x=w769, y=w768) -> (x .and. y?=w767:bool)
            n443 = case shown="True" w767 {
              frame False {
              }
              frame True {
                n444 = property on="A1-position-X" class="DigNum (strict)"() -> (error out=w775:errorcluster, "Value"=w773:dbl)  [unwired: 2 in, 1 out]
                n445 = property on="A1-position-Y" class="DigNum (strict)"(error in=w775) -> (error out=w774:errorcluster, "Value"=w772:dbl)  [unwired: 1 in, 1 out]
                n446 = vi-ref "goto.vi"() -> (w779:refnum<vi>)
                n447 = property class="VI"(reference=w779, error in=w774) -> ("Name"=w778:string)  [unwired: 2 out]
                n448 = Open VI Reference(type specifier VI Refnum (for type only)=refnum<vi> refnum, vi path=w778, options=128) -> (vi reference=w776:refnum<vi>)  [unwired: 3 in, 1 out]
                n449 = call-by-ref "Start Asynchronous Call"(reference=w776, "Y(mm)"=w772, "X(mm)"=w773) -> ()  [unwired: 10 in, 3 out]
              }
            }
            n450 = property on="currentNO" class="Str"("Value"="A1") -> ()  [unwired: 2 in, 2 out]
          }
          event "A2": Value Change {
            n451 = event-data() -> ("NewVal"=w783:bool)  [unwired: 1 in, 5 out]
            n452 = property on="移动" class="Bool (strict)"() -> ("Value"=w786:bool)  [unwired: 2 in, 2 out]
            n453 = Not(x=w786) -> (.not. x?=w785:bool)
            n454 = And(x=w785, y=w783) -> (x .and. y?=w784:bool)
            n455 = case shown="True" w784 {
              frame False {
              }
              frame True {
                n456 = property on="A1-position-X" class="DigNum (strict)"() -> (error out=w790:errorcluster, "Value"=w797:dbl)  [unwired: 2 in, 1 out]
                n457 = property on="A1-position-Y" class="DigNum (strict)"(error in=w790) -> (error out=w789:errorcluster, "Value"=w787:dbl)  [unwired: 1 in, 1 out]
                n458 = Subtract(x=w797, y=4.5) -> (x-y=w788:dbl)
                n459 = vi-ref "goto.vi"() -> (w795:refnum<vi>)
                n460 = property class="VI"(reference=w795, error in=w789) -> ("Name"=w794:string)  [unwired: 2 out]
                n461 = Open VI Reference(type specifier VI Refnum (for type only)=refnum<vi> refnum, vi path=w794, options=128) -> (vi reference=w792:refnum<vi>)  [unwired: 3 in, 1 out]
                n462 = call-by-ref "Start Asynchronous Call"(reference=w792, "Y(mm)"=w787, "X(mm)"=w788) -> ()  [unwired: 10 in, 3 out]
              }
            }
            n463 = control-ref of="currentNO"() -> (w780:refnum<vi>)
            n464 = property on="属性节点" class="Str"(reference=w780, "Value"="A2") -> ()  [unwired: 1 in, 2 out]
          }
          event "A3": Value Change {
            n465 = event-data() -> ("NewVal"=w801:bool)  [unwired: 1 in, 5 out]
            n466 = property on="移动" class="Bool (strict)"() -> ("Value"=w804:bool)  [unwired: 2 in, 2 out]
            n467 = Not(x=w804) -> (.not. x?=w803:bool)
            n468 = And(x=w803, y=w801) -> (x .and. y?=w802:bool)
            n469 = case shown="True" w802 {
              frame False {
              }
              frame True {
                n470 = property on="A1-position-X" class="DigNum (strict)"() -> (error out=w808:errorcluster, "Value"=w815:dbl)  [unwired: 2 in, 1 out]
                n471 = property on="A1-position-Y" class="DigNum (strict)"(error in=w808) -> (error out=w807:errorcluster, "Value"=w805:dbl)  [unwired: 1 in, 1 out]
                n472 = Subtract(x=w815, y=9.0) -> (x-y=w806:dbl)
                n473 = vi-ref "goto.vi"() -> (w813:refnum<vi>)
                n474 = property class="VI"(reference=w813, error in=w807) -> ("Name"=w812:string)  [unwired: 2 out]
                n475 = Open VI Reference(type specifier VI Refnum (for type only)=refnum<vi> refnum, vi path=w812, options=128) -> (vi reference=w810:refnum<vi>)  [unwired: 3 in, 1 out]
                n476 = call-by-ref "Start Asynchronous Call"(reference=w810, "Y(mm)"=w805, "X(mm)"=w806) -> ()  [unwired: 10 in, 3 out]
              }
            }
            n477 = control-ref of="currentNO"() -> (w798:refnum<vi>)
            n478 = property on="属性节点" class="Str"(reference=w798, "Value"="A3") -> ()  [unwired: 1 in, 2 out]
          }
          event "A4": Value Change {
            n479 = event-data() -> ("NewVal"=w818:bool)  [unwired: 1 in, 5 out]
            n480 = property on="移动" class="Bool (strict)"() -> ("Value"=w821:bool)  [unwired: 2 in, 2 out]
            n481 = Not(x=w821) -> (.not. x?=w820:bool)
            n482 = And(x=w820, y=w818) -> (x .and. y?=w819:bool)
            n483 = case shown="True" w819 {
              frame False {
              }
              frame True {
                n484 = property on="A1-position-X" class="DigNum (strict)"() -> (error out=w825:errorcluster, "Value"=w832:dbl)  [unwired: 2 in, 1 out]
                n485 = property on="A1-position-Y" class="DigNum (strict)"(error in=w825) -> (error out=w824:errorcluster, "Value"=w822:dbl)  [unwired: 1 in, 1 out]
                n486 = Subtract(x=w832, y=13.5) -> (x-y=w823:dbl)
                n487 = vi-ref "goto.vi"() -> (w830:refnum<vi>)
                n488 = property class="VI"(reference=w830, error in=w824) -> ("Name"=w829:string)  [unwired: 2 out]
                n489 = Open VI Reference(type specifier VI Refnum (for type only)=refnum<vi> refnum, vi path=w829, options=128) -> (vi reference=w827:refnum<vi>)  [unwired: 3 in, 1 out]
                n490 = call-by-ref "Start Asynchronous Call"(reference=w827, "Y(mm)"=w822, "X(mm)"=w823) -> ()  [unwired: 10 in, 3 out]
              }
            }
            n491 = property on="currentNO" class="Str"("Value"="A4") -> ()  [unwired: 2 in, 2 out]
          }
          event "A5": Value Change {
            n492 = event-data() -> ("NewVal"=w835:bool)  [unwired: 1 in, 5 out]
            n493 = property on="移动" class="Bool (strict)"() -> ("Value"=w838:bool)  [unwired: 2 in, 2 out]
            n494 = Not(x=w838) -> (.not. x?=w837:bool)
            n495 = And(x=w837, y=w835) -> (x .and. y?=w836:bool)
            n496 = case shown="True" w836 {
              frame False {
              }
              frame True {
                n497 = property on="A1-position-X" class="DigNum (strict)"() -> (error out=w842:errorcluster, "Value"=w849:dbl)  [unwired: 2 in, 1 out]
                n498 = property on="A1-position-Y" class="DigNum (strict)"(error in=w842) -> (error out=w841:errorcluster, "Value"=w839:dbl)  [unwired: 1 in, 1 out]
                n499 = Subtract(x=w849, y=18) -> (x-y=w840:dbl)
                n500 = vi-ref "goto.vi"() -> (w847:refnum<vi>)
                n501 = property class="VI"(reference=w847, error in=w841) -> ("Name"=w846:string)  [unwired: 2 out]
                n502 = Open VI Reference(type specifier VI Refnum (for type only)=refnum<vi> refnum, vi path=w846, options=128) -> (vi reference=w844:refnum<vi>)  [unwired: 3 in, 1 out]
                n503 = call-by-ref "Start Asynchronous Call"(reference=w844, "Y(mm)"=w839, "X(mm)"=w840) -> ()  [unwired: 10 in, 3 out]
              }
            }
            n504 = property on="currentNO" class="Str"("Value"="A5") -> ()  [unwired: 2 in, 2 out]
          }
          event "A6": Value Change {
            n505 = event-data() -> ("NewVal"=w852:bool)  [unwired: 1 in, 5 out]
            n506 = property on="移动" class="Bool (strict)"() -> ("Value"=w855:bool)  [unwired: 2 in, 2 out]
            n507 = Not(x=w855) -> (.not. x?=w854:bool)
            n508 = And(x=w854, y=w852) -> (x .and. y?=w853:bool)
            n509 = case shown="True" w853 {
              frame False {
              }
              frame True {
                n510 = property on="A1-position-X" class="DigNum (strict)"() -> (error out=w859:errorcluster, "Value"=w866:dbl)  [unwired: 2 in, 1 out]
                n511 = property on="A1-position-Y" class="DigNum (strict)"(error in=w859) -> (error out=w858:errorcluster, "Value"=w856:dbl)  [unwired: 1 in, 1 out]
                n512 = Subtract(x=w866, y=22.5) -> (x-y=w857:dbl)
                n513 = vi-ref "goto.vi"() -> (w864:refnum<vi>)
                n514 = property class="VI"(reference=w864, error in=w858) -> ("Name"=w863:string)  [unwired: 2 out]
                n515 = Open VI Reference(type specifier VI Refnum (for type only)=refnum<vi> refnum, vi path=w863, options=128) -> (vi reference=w861:refnum<vi>)  [unwired: 3 in, 1 out]
                n516 = call-by-ref "Start Asynchronous Call"(reference=w861, "Y(mm)"=w856, "X(mm)"=w857) -> ()  [unwired: 10 in, 3 out]
              }
            }
            n517 = property on="currentNO" class="Str"("Value"="A6") -> ()  [unwired: 2 in, 2 out]
          }
          event "A7": Value Change {
            n518 = event-data() -> ("NewVal"=w869:bool)  [unwired: 1 in, 5 out]
            n519 = property on="移动" class="Bool (strict)"() -> ("Value"=w872:bool)  [unwired: 2 in, 2 out]
            n520 = Not(x=w872) -> (.not. x?=w871:bool)
            n521 = And(x=w871, y=w869) -> (x .and. y?=w870:bool)
            n522 = case shown="True" w870 {
              frame False {
              }
              frame True {
                n523 = property on="A1-position-X" class="DigNum (strict)"() -> (error out=w876:errorcluster, "Value"=w883:dbl)  [unwired: 2 in, 1 out]
                n524 = property on="A1-position-Y" class="DigNum (strict)"(error in=w876) -> (error out=w875:errorcluster, "Value"=w873:dbl)  [unwired: 1 in, 1 out]
                n525 = Subtract(x=w883, y=27) -> (x-y=w874:dbl)
                n526 = vi-ref "goto.vi"() -> (w881:refnum<vi>)
                n527 = property class="VI"(reference=w881, error in=w875) -> ("Name"=w880:string)  [unwired: 2 out]
                n528 = Open VI Reference(type specifier VI Refnum (for type only)=refnum<vi> refnum, vi path=w880, options=128) -> (vi reference=w878:refnum<vi>)  [unwired: 3 in, 1 out]
                n529 = call-by-ref "Start Asynchronous Call"(reference=w878, "Y(mm)"=w873, "X(mm)"=w874) -> ()  [unwired: 10 in, 3 out]
              }
            }
            n530 = property on="currentNO" class="Str"("Value"="A7") -> ()  [unwired: 2 in, 2 out]
          }
          event User Event {
            n531 = event-data() -> ("PV name"=w885:string, "value array (string)"=w884:string[])  [unwired: 1 in, 9 out]
            n532 = case shown="\"ID:STATUS\"" w885 {
              tunnel: w887 -> [w891 w897]
              tunnel: [w891 w900] -> w886
              tunnel: w884 -> [w890 _]
              frame "ID:INFO", Default {
                n533 = Index Array(array=w890, index=0) -> (element=→"idn status":string)
              }
              frame "ID:STATUS" {
                n534 = call "getIOCdata.vi"() -> ("输出簇"=w898:T11)  [unwired: 11 in]
                n535 = call-poly <userlib>:"CaLabGet.vi"("PV Name"="MS:NUM") -> ("1rst Value (number)"=w896:dbl)  [unwired: 8 in, 6 out]
                n536 = Index Array(array=w897, index=w896) -> (element=w895:T11)
                n537 = Unbundle By Name(w895) -> ("NO"=w894:string, "tag2"=w893:string)
                n538 = Bundle By Name(cluster=w898, "NO"=w894, "tag2"=w893) -> (w892:T11)
                n539 = Replace Array Subset "Replace Array Subset"(array=w897, new element=w892, index=w896) -> (w900:T8)
                n540 = for {
                  tunnel: w900 -> [w910] mode=indexing
                  shift-right: [w903] -> w899
                  shift-left: string[][] [] ("Item Names") -> [w905]
                  i -> [w906]
                  n541 = Unbundle By Name(w910) -> ("NO"=w909:string, "tag1"=w908:string, "tag2"=w907:string)
                  n542 = Build Array(w909, w908, w907) -> (w904:string[])
                  n543 = Insert Into Array "Insert Into Array"(array=w905, index (row)=w906, new element=w904) -> (w903:string[][])  [unwired: 1 in]
                }
                n544 = property on="测试记录" class="MCListbox (strict)"("ItemNames"=w899) -> ()  [unwired: 2 in, 2 out]
              }
            }
          }
          event "A8": Value Change {
            n545 = event-data() -> ("NewVal"=w913:bool)  [unwired: 1 in, 5 out]
            n546 = property on="移动" class="Bool (strict)"() -> ("Value"=w916:bool)  [unwired: 2 in, 2 out]
            n547 = Not(x=w916) -> (.not. x?=w915:bool)
            n548 = And(x=w915, y=w913) -> (x .and. y?=w914:bool)
            n549 = case shown="True" w914 {
              frame False {
              }
              frame True {
                n550 = property on="A1-position-X" class="DigNum (strict)"() -> (error out=w920:errorcluster, "Value"=w927:dbl)  [unwired: 2 in, 1 out]
                n551 = property on="A1-position-Y" class="DigNum (strict)"(error in=w920) -> (error out=w919:errorcluster, "Value"=w917:dbl)  [unwired: 1 in, 1 out]
                n552 = Subtract(x=w927, y=31.5) -> (x-y=w918:dbl)
                n553 = vi-ref "goto.vi"() -> (w925:refnum<vi>)
                n554 = property class="VI"(reference=w925, error in=w919) -> ("Name"=w924:string)  [unwired: 2 out]
                n555 = Open VI Reference(type specifier VI Refnum (for type only)=refnum<vi> refnum, vi path=w924, options=128) -> (vi reference=w922:refnum<vi>)  [unwired: 3 in, 1 out]
                n556 = call-by-ref "Start Asynchronous Call"(reference=w922, "Y(mm)"=w917, "X(mm)"=w918) -> ()  [unwired: 10 in, 3 out]
              }
            }
            n557 = property on="currentNO" class="Str"("Value"="A8") -> ()  [unwired: 2 in, 2 out]
          }
          event "A9": Value Change {
            n558 = event-data() -> ("NewVal"=w930:bool)  [unwired: 1 in, 5 out]
            n559 = property on="移动" class="Bool (strict)"() -> ("Value"=w933:bool)  [unwired: 2 in, 2 out]
            n560 = Not(x=w933) -> (.not. x?=w932:bool)
            n561 = And(x=w932, y=w930) -> (x .and. y?=w931:bool)
            n562 = case shown="True" w931 {
              frame False {
              }
              frame True {
                n563 = property on="A1-position-X" class="DigNum (strict)"() -> (error out=w937:errorcluster, "Value"=w944:dbl)  [unwired: 2 in, 1 out]
                n564 = property on="A1-position-Y" class="DigNum (strict)"(error in=w937) -> (error out=w936:errorcluster, "Value"=w934:dbl)  [unwired: 1 in, 1 out]
                n565 = Subtract(x=w944, y=36) -> (x-y=w935:dbl)
                n566 = vi-ref "goto.vi"() -> (w942:refnum<vi>)
                n567 = property class="VI"(reference=w942, error in=w936) -> ("Name"=w941:string)  [unwired: 2 out]
                n568 = Open VI Reference(type specifier VI Refnum (for type only)=refnum<vi> refnum, vi path=w941, options=128) -> (vi reference=w939:refnum<vi>)  [unwired: 3 in, 1 out]
                n569 = call-by-ref "Start Asynchronous Call"(reference=w939, "Y(mm)"=w934, "X(mm)"=w935) -> ()  [unwired: 10 in, 3 out]
              }
            }
            n570 = property on="currentNO" class="Str"("Value"="A9") -> ()  [unwired: 2 in, 2 out]
          }
          event "A10": Value Change {
            n571 = event-data() -> ("NewVal"=w947:bool)  [unwired: 1 in, 5 out]
            n572 = property on="移动" class="Bool (strict)"() -> ("Value"=w950:bool)  [unwired: 2 in, 2 out]
            n573 = Not(x=w950) -> (.not. x?=w949:bool)
            n574 = And(x=w949, y=w947) -> (x .and. y?=w948:bool)
            n575 = case shown="True" w948 {
              frame False {
              }
              frame True {
                n576 = property on="A1-position-X" class="DigNum (strict)"() -> (error out=w954:errorcluster, "Value"=w961:dbl)  [unwired: 2 in, 1 out]
                n577 = property on="A1-position-Y" class="DigNum (strict)"(error in=w954) -> (error out=w953:errorcluster, "Value"=w951:dbl)  [unwired: 1 in, 1 out]
                n578 = Subtract(x=w961, y=40.5) -> (x-y=w952:dbl)
                n579 = vi-ref "goto.vi"() -> (w959:refnum<vi>)
                n580 = property class="VI"(reference=w959, error in=w953) -> ("Name"=w958:string)  [unwired: 2 out]
                n581 = Open VI Reference(type specifier VI Refnum (for type only)=refnum<vi> refnum, vi path=w958, options=128) -> (vi reference=w956:refnum<vi>)  [unwired: 3 in, 1 out]
                n582 = call-by-ref "Start Asynchronous Call"(reference=w956, "Y(mm)"=w951, "X(mm)"=w952) -> ()  [unwired: 10 in, 3 out]
              }
            }
            n583 = property on="currentNO" class="Str"("Value"="A10") -> ()  [unwired: 2 in, 2 out]
          }
          event "A11": Value Change {
            n584 = event-data() -> ("NewVal"=w964:bool)  [unwired: 1 in, 5 out]
            n585 = property on="移动" class="Bool (strict)"() -> ("Value"=w967:bool)  [unwired: 2 in, 2 out]
            n586 = Not(x=w967) -> (.not. x?=w966:bool)
            n587 = And(x=w966, y=w964) -> (x .and. y?=w965:bool)
            n588 = case shown="True" w965 {
              frame False {
              }
              frame True {
                n589 = property on="A1-position-X" class="DigNum (strict)"() -> (error out=w971:errorcluster, "Value"=w978:dbl)  [unwired: 2 in, 1 out]
                n590 = property on="A1-position-Y" class="DigNum (strict)"(error in=w971) -> (error out=w970:errorcluster, "Value"=w968:dbl)  [unwired: 1 in, 1 out]
                n591 = Subtract(x=w978, y=45) -> (x-y=w969:dbl)
                n592 = vi-ref "goto.vi"() -> (w976:refnum<vi>)
                n593 = property class="VI"(reference=w976, error in=w970) -> ("Name"=w975:string)  [unwired: 2 out]
                n594 = Open VI Reference(type specifier VI Refnum (for type only)=refnum<vi> refnum, vi path=w975, options=128) -> (vi reference=w973:refnum<vi>)  [unwired: 3 in, 1 out]
                n595 = call-by-ref "Start Asynchronous Call"(reference=w973, "Y(mm)"=w968, "X(mm)"=w969) -> ()  [unwired: 10 in, 3 out]
              }
            }
            n596 = property on="currentNO" class="Str"("Value"="A11") -> ()  [unwired: 2 in, 2 out]
          }
          event "A12": Value Change {
            n597 = event-data() -> ("NewVal"=w981:bool)  [unwired: 1 in, 5 out]
            n598 = property on="移动" class="Bool (strict)"() -> ("Value"=w984:bool)  [unwired: 2 in, 2 out]
            n599 = Not(x=w984) -> (.not. x?=w983:bool)
            n600 = And(x=w983, y=w981) -> (x .and. y?=w982:bool)
            n601 = case shown="True" w982 {
              frame False {
              }
              frame True {
                n602 = property on="A1-position-X" class="DigNum (strict)"() -> (error out=w988:errorcluster, "Value"=w995:dbl)  [unwired: 2 in, 1 out]
                n603 = property on="A1-position-Y" class="DigNum (strict)"(error in=w988) -> (error out=w987:errorcluster, "Value"=w985:dbl)  [unwired: 1 in, 1 out]
                n604 = Subtract(x=w995, y=49.5) -> (x-y=w986:dbl)
                n605 = vi-ref "goto.vi"() -> (w993:refnum<vi>)
                n606 = property class="VI"(reference=w993, error in=w987) -> ("Name"=w992:string)  [unwired: 2 out]
                n607 = Open VI Reference(type specifier VI Refnum (for type only)=refnum<vi> refnum, vi path=w992, options=128) -> (vi reference=w990:refnum<vi>)  [unwired: 3 in, 1 out]
                n608 = call-by-ref "Start Asynchronous Call"(reference=w990, "Y(mm)"=w985, "X(mm)"=w986) -> ()  [unwired: 10 in, 3 out]
              }
            }
            n609 = property on="currentNO" class="Str"("Value"="A12") -> ()  [unwired: 2 in, 2 out]
          }
          event "B1": Value Change {
            n610 = event-data() -> ("NewVal"=w998:bool)  [unwired: 1 in, 5 out]
            n611 = property on="移动" class="Bool (strict)"() -> ("Value"=w1001:bool)  [unwired: 2 in, 2 out]
            n612 = Not(x=w1001) -> (.not. x?=w1000:bool)
            n613 = And(x=w1000, y=w998) -> (x .and. y?=w999:bool)
            n614 = case shown="True" w999 {
              frame False {
              }
              frame True {
                n615 = property on="A1-position-X" class="DigNum (strict)"() -> (error out=w1007:errorcluster, "Value"=w1014:dbl)  [unwired: 2 in, 1 out]
                n616 = property on="A1-position-Y" class="DigNum (strict)"(error in=w1007) -> (error out=w1006:errorcluster, "Value"=w1003:dbl)  [unwired: 1 in, 1 out]
                n617 = Subtract(x=w1003, y=4.5) -> (x-y=w1002:dbl)
                n618 = Subtract(x=w1014, y=0) -> (x-y=w1005:dbl)
                n619 = vi-ref "goto.vi"() -> (w1012:refnum<vi>)
                n620 = property class="VI"(reference=w1012, error in=w1006) -> ("Name"=w1011:string)  [unwired: 2 out]
                n621 = Open VI Reference(type specifier VI Refnum (for type only)=refnum<vi> refnum, vi path=w1011, options=128) -> (vi reference=w1009:refnum<vi>)  [unwired: 3 in, 1 out]
                n622 = call-by-ref "Start Asynchronous Call"(reference=w1009, "Y(mm)"=w1002, "X(mm)"=w1005) -> ()  [unwired: 10 in, 3 out]
              }
            }
            n623 = property on="currentNO" class="Str"("Value"="B1") -> ()  [unwired: 2 in, 2 out]
          }
          event "B2": Value Change {
            n624 = event-data() -> ("NewVal"=w1017:bool)  [unwired: 1 in, 5 out]
            n625 = property on="移动" class="Bool (strict)"() -> ("Value"=w1020:bool)  [unwired: 2 in, 2 out]
            n626 = Not(x=w1020) -> (.not. x?=w1019:bool)
            n627 = And(x=w1019, y=w1017) -> (x .and. y?=w1018:bool)
            n628 = case shown="True" w1018 {
              frame False {
              }
              frame True {
                n629 = property on="A1-position-X" class="DigNum (strict)"() -> (error out=w1026:errorcluster, "Value"=w1033:dbl)  [unwired: 2 in, 1 out]
                n630 = property on="A1-position-Y" class="DigNum (strict)"(error in=w1026) -> (error out=w1025:errorcluster, "Value"=w1022:dbl)  [unwired: 1 in, 1 out]
                n631 = Subtract(x=w1022, y=4.5) -> (x-y=w1021:dbl)
                n632 = Subtract(x=w1033, y=4.5) -> (x-y=w1024:dbl)
                n633 = vi-ref "goto.vi"() -> (w1031:refnum<vi>)
                n634 = property class="VI"(reference=w1031, error in=w1025) -> ("Name"=w1030:string)  [unwired: 2 out]
                n635 = Open VI Reference(type specifier VI Refnum (for type only)=refnum<vi> refnum, vi path=w1030, options=128) -> (vi reference=w1028:refnum<vi>)  [unwired: 3 in, 1 out]
                n636 = call-by-ref "Start Asynchronous Call"(reference=w1028, "Y(mm)"=w1021, "X(mm)"=w1024) -> ()  [unwired: 10 in, 3 out]
              }
            }
            n637 = property on="currentNO" class="Str"("Value"="B2") -> ()  [unwired: 2 in, 2 out]
          }
          event "B3": Value Change {
            n638 = event-data() -> ("NewVal"=w1036:bool)  [unwired: 1 in, 5 out]
            n639 = property on="移动" class="Bool (strict)"() -> ("Value"=w1039:bool)  [unwired: 2 in, 2 out]
            n640 = Not(x=w1039) -> (.not. x?=w1038:bool)
            n641 = And(x=w1038, y=w1036) -> (x .and. y?=w1037:bool)
            n642 = case shown="True" w1037 {
              frame False {
              }
              frame True {
                n643 = property on="A1-position-X" class="DigNum (strict)"() -> (error out=w1045:errorcluster, "Value"=w1052:dbl)  [unwired: 2 in, 1 out]
                n644 = property on="A1-position-Y" class="DigNum (strict)"(error in=w1045) -> (error out=w1044:errorcluster, "Value"=w1041:dbl)  [unwired: 1 in, 1 out]
                n645 = Subtract(x=w1041, y=4.5) -> (x-y=w1040:dbl)
                n646 = Subtract(x=w1052, y=9) -> (x-y=w1043:dbl)
                n647 = vi-ref "goto.vi"() -> (w1050:refnum<vi>)
                n648 = property class="VI"(reference=w1050, error in=w1044) -> ("Name"=w1049:string)  [unwired: 2 out]
                n649 = Open VI Reference(type specifier VI Refnum (for type only)=refnum<vi> refnum, vi path=w1049, options=128) -> (vi reference=w1047:refnum<vi>)  [unwired: 3 in, 1 out]
                n650 = call-by-ref "Start Asynchronous Call"(reference=w1047, "Y(mm)"=w1040, "X(mm)"=w1043) -> ()  [unwired: 10 in, 3 out]
              }
            }
            n651 = property on="currentNO" class="Str"("Value"="B3") -> ()  [unwired: 2 in, 2 out]
          }
          event "B4": Value Change {
            n652 = event-data() -> ("NewVal"=w1055:bool)  [unwired: 1 in, 5 out]
            n653 = property on="移动" class="Bool (strict)"() -> ("Value"=w1058:bool)  [unwired: 2 in, 2 out]
            n654 = Not(x=w1058) -> (.not. x?=w1057:bool)
            n655 = And(x=w1057, y=w1055) -> (x .and. y?=w1056:bool)
            n656 = case shown="True" w1056 {
              frame False {
              }
              frame True {
                n657 = property on="A1-position-X" class="DigNum (strict)"() -> (error out=w1064:errorcluster, "Value"=w1071:dbl)  [unwired: 2 in, 1 out]
                n658 = property on="A1-position-Y" class="DigNum (strict)"(error in=w1064) -> (error out=w1063:errorcluster, "Value"=w1060:dbl)  [unwired: 1 in, 1 out]
                n659 = Subtract(x=w1060, y=4.5) -> (x-y=w1059:dbl)
                n660 = Subtract(x=w1071, y=13.5) -> (x-y=w1062:dbl)
                n661 = vi-ref "goto.vi"() -> (w1069:refnum<vi>)
                n662 = property class="VI"(reference=w1069, error in=w1063) -> ("Name"=w1068:string)  [unwired: 2 out]
                n663 = Open VI Reference(type specifier VI Refnum (for type only)=refnum<vi> refnum, vi path=w1068, options=128) -> (vi reference=w1066:refnum<vi>)  [unwired: 3 in, 1 out]
                n664 = call-by-ref "Start Asynchronous Call"(reference=w1066, "Y(mm)"=w1059, "X(mm)"=w1062) -> ()  [unwired: 10 in, 3 out]
              }
            }
            n665 = property on="currentNO" class="Str"("Value"="B4") -> ()  [unwired: 2 in, 2 out]
          }
          event "B5": Value Change {
            n666 = event-data() -> ("NewVal"=w1074:bool)  [unwired: 1 in, 5 out]
            n667 = property on="移动" class="Bool (strict)"() -> ("Value"=w1077:bool)  [unwired: 2 in, 2 out]
            n668 = Not(x=w1077) -> (.not. x?=w1076:bool)
            n669 = And(x=w1076, y=w1074) -> (x .and. y?=w1075:bool)
            n670 = case shown="True" w1075 {
              frame False {
              }
              frame True {
                n671 = property on="A1-position-X" class="DigNum (strict)"() -> (error out=w1083:errorcluster, "Value"=w1090:dbl)  [unwired: 2 in, 1 out]
                n672 = property on="A1-position-Y" class="DigNum (strict)"(error in=w1083) -> (error out=w1082:errorcluster, "Value"=w1079:dbl)  [unwired: 1 in, 1 out]
                n673 = Subtract(x=w1079, y=4.5) -> (x-y=w1078:dbl)
                n674 = Subtract(x=w1090, y=18) -> (x-y=w1081:dbl)
                n675 = vi-ref "goto.vi"() -> (w1088:refnum<vi>)
                n676 = property class="VI"(reference=w1088, error in=w1082) -> ("Name"=w1087:string)  [unwired: 2 out]
                n677 = Open VI Reference(type specifier VI Refnum (for type only)=refnum<vi> refnum, vi path=w1087, options=128) -> (vi reference=w1085:refnum<vi>)  [unwired: 3 in, 1 out]
                n678 = call-by-ref "Start Asynchronous Call"(reference=w1085, "Y(mm)"=w1078, "X(mm)"=w1081) -> ()  [unwired: 10 in, 3 out]
              }
            }
            n679 = property on="currentNO" class="Str"("Value"="B5") -> ()  [unwired: 2 in, 2 out]
          }
          event "B6": Value Change {
            n680 = event-data() -> ("NewVal"=w1093:bool)  [unwired: 1 in, 5 out]
            n681 = property on="移动" class="Bool (strict)"() -> ("Value"=w1096:bool)  [unwired: 2 in, 2 out]
            n682 = Not(x=w1096) -> (.not. x?=w1095:bool)
            n683 = And(x=w1095, y=w1093) -> (x .and. y?=w1094:bool)
            n684 = case shown="True" w1094 {
              frame False {
              }
              frame True {
                n685 = property on="A1-position-X" class="DigNum (strict)"() -> (error out=w1102:errorcluster, "Value"=w1109:dbl)  [unwired: 2 in, 1 out]
                n686 = property on="A1-position-Y" class="DigNum (strict)"(error in=w1102) -> (error out=w1101:errorcluster, "Value"=w1098:dbl)  [unwired: 1 in, 1 out]
                n687 = Subtract(x=w1098, y=4.5) -> (x-y=w1097:dbl)
                n688 = Subtract(x=w1109, y=22.5) -> (x-y=w1100:dbl)
                n689 = vi-ref "goto.vi"() -> (w1107:refnum<vi>)
                n690 = property class="VI"(reference=w1107, error in=w1101) -> ("Name"=w1106:string)  [unwired: 2 out]
                n691 = Open VI Reference(type specifier VI Refnum (for type only)=refnum<vi> refnum, vi path=w1106, options=128) -> (vi reference=w1104:refnum<vi>)  [unwired: 3 in, 1 out]
                n692 = call-by-ref "Start Asynchronous Call"(reference=w1104, "Y(mm)"=w1097, "X(mm)"=w1100) -> ()  [unwired: 10 in, 3 out]
              }
            }
            n693 = property on="currentNO" class="Str"("Value"="B6") -> ()  [unwired: 2 in, 2 out]
          }
          event "B7": Value Change {
            n694 = event-data() -> ("NewVal"=w1111:bool)  [unwired: 1 in, 5 out]
            n695 = property on="移动" class="Bool (strict)"() -> ("Value"=w1114:bool)  [unwired: 2 in, 2 out]
            n696 = Not(x=w1114) -> (.not. x?=w1113:bool)
            n697 = And(x=w1113, y=w1111) -> (x .and. y?=w1112:bool)
            n698 = case shown="True" w1112 {
              frame False {
              }
              frame True {
                n699 = property on="A1-position-X" class="DigNum (strict)"() -> (error out=w1120:errorcluster, "Value"=w1127:dbl)  [unwired: 2 in, 1 out]
                n700 = property on="A1-position-Y" class="DigNum (strict)"(error in=w1120) -> (error out=w1119:errorcluster, "Value"=w1116:dbl)  [unwired: 1 in, 1 out]
                n701 = Subtract(x=w1116, y=4.5) -> (x-y=w1115:dbl)
                n702 = Subtract(x=w1127, y=27) -> (x-y=w1118:dbl)
                n703 = vi-ref "goto.vi"() -> (w1125:refnum<vi>)
                n704 = property class="VI"(reference=w1125, error in=w1119) -> ("Name"=w1124:string)  [unwired: 2 out]
                n705 = Open VI Reference(type specifier VI Refnum (for type only)=refnum<vi> refnum, vi path=w1124, options=128) -> (vi reference=w1122:refnum<vi>)  [unwired: 3 in, 1 out]
                n706 = call-by-ref "Start Asynchronous Call"(reference=w1122, "Y(mm)"=w1115, "X(mm)"=w1118) -> ()  [unwired: 10 in, 3 out]
              }
            }
          }
          event "B8": Value Change {
            n707 = event-data() -> ("NewVal"=w1129:bool)  [unwired: 1 in, 5 out]
            n708 = property on="移动" class="Bool (strict)"() -> ("Value"=w1132:bool)  [unwired: 2 in, 2 out]
            n709 = Not(x=w1132) -> (.not. x?=w1131:bool)
            n710 = And(x=w1131, y=w1129) -> (x .and. y?=w1130:bool)
            n711 = case shown="True" w1130 {
              frame False {
              }
              frame True {
                n712 = property on="A1-position-X" class="DigNum (strict)"() -> (error out=w1138:errorcluster, "Value"=w1145:dbl)  [unwired: 2 in, 1 out]
                n713 = property on="A1-position-Y" class="DigNum (strict)"(error in=w1138) -> (error out=w1137:errorcluster, "Value"=w1134:dbl)  [unwired: 1 in, 1 out]
                n714 = Subtract(x=w1134, y=4.5) -> (x-y=w1133:dbl)
                n715 = Subtract(x=w1145, y=31.5) -> (x-y=w1136:dbl)
                n716 = vi-ref "goto.vi"() -> (w1143:refnum<vi>)
                n717 = property class="VI"(reference=w1143, error in=w1137) -> ("Name"=w1142:string)  [unwired: 2 out]
                n718 = Open VI Reference(type specifier VI Refnum (for type only)=refnum<vi> refnum, vi path=w1142, options=128) -> (vi reference=w1140:refnum<vi>)  [unwired: 3 in, 1 out]
                n719 = call-by-ref "Start Asynchronous Call"(reference=w1140, "Y(mm)"=w1133, "X(mm)"=w1136) -> ()  [unwired: 10 in, 3 out]
              }
            }
          }
          event "B9": Value Change {
            n720 = event-data() -> ("NewVal"=w1147:bool)  [unwired: 1 in, 5 out]
            n721 = property on="移动" class="Bool (strict)"() -> ("Value"=w1150:bool)  [unwired: 2 in, 2 out]
            n722 = Not(x=w1150) -> (.not. x?=w1149:bool)
            n723 = And(x=w1149, y=w1147) -> (x .and. y?=w1148:bool)
            n724 = case shown="True" w1148 {
              frame False {
              }
              frame True {
                n725 = property on="A1-position-X" class="DigNum (strict)"() -> (error out=w1156:errorcluster, "Value"=w1163:dbl)  [unwired: 2 in, 1 out]
                n726 = property on="A1-position-Y" class="DigNum (strict)"(error in=w1156) -> (error out=w1155:errorcluster, "Value"=w1152:dbl)  [unwired: 1 in, 1 out]
                n727 = Subtract(x=w1152, y=4.5) -> (x-y=w1151:dbl)
                n728 = Subtract(x=w1163, y=36) -> (x-y=w1154:dbl)
                n729 = vi-ref "goto.vi"() -> (w1161:refnum<vi>)
                n730 = property class="VI"(reference=w1161, error in=w1155) -> ("Name"=w1160:string)  [unwired: 2 out]
                n731 = Open VI Reference(type specifier VI Refnum (for type only)=refnum<vi> refnum, vi path=w1160, options=128) -> (vi reference=w1158:refnum<vi>)  [unwired: 3 in, 1 out]
                n732 = call-by-ref "Start Asynchronous Call"(reference=w1158, "Y(mm)"=w1151, "X(mm)"=w1154) -> ()  [unwired: 10 in, 3 out]
              }
            }
          }
          event "B10": Value Change {
            n733 = event-data() -> ("NewVal"=w1165:bool)  [unwired: 1 in, 5 out]
            n734 = property on="移动" class="Bool (strict)"() -> ("Value"=w1168:bool)  [unwired: 2 in, 2 out]
            n735 = Not(x=w1168) -> (.not. x?=w1167:bool)
            n736 = And(x=w1167, y=w1165) -> (x .and. y?=w1166:bool)
            n737 = case shown="True" w1166 {
              frame False {
              }
              frame True {
                n738 = property on="A1-position-X" class="DigNum (strict)"() -> (error out=w1174:errorcluster, "Value"=w1181:dbl)  [unwired: 2 in, 1 out]
                n739 = property on="A1-position-Y" class="DigNum (strict)"(error in=w1174) -> (error out=w1173:errorcluster, "Value"=w1170:dbl)  [unwired: 1 in, 1 out]
                n740 = Subtract(x=w1170, y=4.5) -> (x-y=w1169:dbl)
                n741 = Subtract(x=w1181, y=40.5) -> (x-y=w1172:dbl)
                n742 = vi-ref "goto.vi"() -> (w1179:refnum<vi>)
                n743 = property class="VI"(reference=w1179, error in=w1173) -> ("Name"=w1178:string)  [unwired: 2 out]
                n744 = Open VI Reference(type specifier VI Refnum (for type only)=refnum<vi> refnum, vi path=w1178, options=128) -> (vi reference=w1176:refnum<vi>)  [unwired: 3 in, 1 out]
                n745 = call-by-ref "Start Asynchronous Call"(reference=w1176, "Y(mm)"=w1169, "X(mm)"=w1172) -> ()  [unwired: 10 in, 3 out]
              }
            }
          }
          event "B11": Value Change {
            n746 = event-data() -> ("NewVal"=w1183:bool)  [unwired: 1 in, 5 out]
            n747 = property on="移动" class="Bool (strict)"() -> ("Value"=w1186:bool)  [unwired: 2 in, 2 out]
            n748 = Not(x=w1186) -> (.not. x?=w1185:bool)
            n749 = And(x=w1185, y=w1183) -> (x .and. y?=w1184:bool)
            n750 = case shown="True" w1184 {
              frame False {
              }
              frame True {
                n751 = property on="A1-position-X" class="DigNum (strict)"() -> (error out=w1192:errorcluster, "Value"=w1199:dbl)  [unwired: 2 in, 1 out]
                n752 = property on="A1-position-Y" class="DigNum (strict)"(error in=w1192) -> (error out=w1191:errorcluster, "Value"=w1188:dbl)  [unwired: 1 in, 1 out]
                n753 = Subtract(x=w1188, y=4.5) -> (x-y=w1187:dbl)
                n754 = Subtract(x=w1199, y=45) -> (x-y=w1190:dbl)
                n755 = vi-ref "goto.vi"() -> (w1197:refnum<vi>)
                n756 = property class="VI"(reference=w1197, error in=w1191) -> ("Name"=w1196:string)  [unwired: 2 out]
                n757 = Open VI Reference(type specifier VI Refnum (for type only)=refnum<vi> refnum, vi path=w1196, options=128) -> (vi reference=w1194:refnum<vi>)  [unwired: 3 in, 1 out]
                n758 = call-by-ref "Start Asynchronous Call"(reference=w1194, "Y(mm)"=w1187, "X(mm)"=w1190) -> ()  [unwired: 10 in, 3 out]
              }
            }
          }
          event "B12": Value Change {
            n759 = event-data() -> ("NewVal"=w1201:bool)  [unwired: 1 in, 5 out]
            n760 = property on="移动" class="Bool (strict)"() -> ("Value"=w1204:bool)  [unwired: 2 in, 2 out]
            n761 = Not(x=w1204) -> (.not. x?=w1203:bool)
            n762 = And(x=w1203, y=w1201) -> (x .and. y?=w1202:bool)
            n763 = case shown="True" w1202 {
              frame False {
              }
              frame True {
                n764 = property on="A1-position-X" class="DigNum (strict)"() -> (error out=w1210:errorcluster, "Value"=w1217:dbl)  [unwired: 2 in, 1 out]
                n765 = property on="A1-position-Y" class="DigNum (strict)"(error in=w1210) -> (error out=w1209:errorcluster, "Value"=w1206:dbl)  [unwired: 1 in, 1 out]
                n766 = Subtract(x=w1206, y=4.5) -> (x-y=w1205:dbl)
                n767 = Subtract(x=w1217, y=49.5) -> (x-y=w1208:dbl)
                n768 = vi-ref "goto.vi"() -> (w1215:refnum<vi>)
                n769 = property class="VI"(reference=w1215, error in=w1209) -> ("Name"=w1214:string)  [unwired: 2 out]
                n770 = Open VI Reference(type specifier VI Refnum (for type only)=refnum<vi> refnum, vi path=w1214, options=128) -> (vi reference=w1212:refnum<vi>)  [unwired: 3 in, 1 out]
                n771 = call-by-ref "Start Asynchronous Call"(reference=w1212, "Y(mm)"=w1205, "X(mm)"=w1208) -> ()  [unwired: 10 in, 3 out]
              }
            }
          }
          event "C1": Value Change {
            n772 = event-data() -> ("NewVal"=w1219:bool)  [unwired: 1 in, 5 out]
            n773 = property on="移动" class="Bool (strict)"() -> ("Value"=w1222:bool)  [unwired: 2 in, 2 out]
            n774 = Not(x=w1222) -> (.not. x?=w1221:bool)
            n775 = And(x=w1221, y=w1219) -> (x .and. y?=w1220:bool)
            n776 = case shown="True" w1220 {
              frame False {
              }
              frame True {
                n777 = property on="A1-position-X" class="DigNum (strict)"() -> (error out=w1228:errorcluster, "Value"=w1235:dbl)  [unwired: 2 in, 1 out]
                n778 = property on="A1-position-Y" class="DigNum (strict)"(error in=w1228) -> (error out=w1227:errorcluster, "Value"=w1224:dbl)  [unwired: 1 in, 1 out]
                n779 = Subtract(x=w1224, y=9) -> (x-y=w1223:dbl)
                n780 = Subtract(x=w1235, y=0) -> (x-y=w1226:dbl)
                n781 = vi-ref "goto.vi"() -> (w1233:refnum<vi>)
                n782 = property class="VI"(reference=w1233, error in=w1227) -> ("Name"=w1232:string)  [unwired: 2 out]
                n783 = Open VI Reference(type specifier VI Refnum (for type only)=refnum<vi> refnum, vi path=w1232, options=128) -> (vi reference=w1230:refnum<vi>)  [unwired: 3 in, 1 out]
                n784 = call-by-ref "Start Asynchronous Call"(reference=w1230, "Y(mm)"=w1223, "X(mm)"=w1226) -> ()  [unwired: 10 in, 3 out]
              }
            }
          }
          event "C2": Value Change {
            n785 = event-data() -> ("NewVal"=w1237:bool)  [unwired: 1 in, 5 out]
            n786 = property on="移动" class="Bool (strict)"() -> ("Value"=w1240:bool)  [unwired: 2 in, 2 out]
            n787 = Not(x=w1240) -> (.not. x?=w1239:bool)
            n788 = And(x=w1239, y=w1237) -> (x .and. y?=w1238:bool)
            n789 = case shown="True" w1238 {
              frame False {
              }
              frame True {
                n790 = property on="A1-position-X" class="DigNum (strict)"() -> (error out=w1246:errorcluster, "Value"=w1253:dbl)  [unwired: 2 in, 1 out]
                n791 = property on="A1-position-Y" class="DigNum (strict)"(error in=w1246) -> (error out=w1245:errorcluster, "Value"=w1242:dbl)  [unwired: 1 in, 1 out]
                n792 = Subtract(x=w1242, y=9) -> (x-y=w1241:dbl)
                n793 = Subtract(x=w1253, y=4.5) -> (x-y=w1244:dbl)
                n794 = vi-ref "goto.vi"() -> (w1251:refnum<vi>)
                n795 = property class="VI"(reference=w1251, error in=w1245) -> ("Name"=w1250:string)  [unwired: 2 out]
                n796 = Open VI Reference(type specifier VI Refnum (for type only)=refnum<vi> refnum, vi path=w1250, options=128) -> (vi reference=w1248:refnum<vi>)  [unwired: 3 in, 1 out]
                n797 = call-by-ref "Start Asynchronous Call"(reference=w1248, "Y(mm)"=w1241, "X(mm)"=w1244) -> ()  [unwired: 10 in, 3 out]
              }
            }
          }
          event "C3": Value Change {
            n798 = event-data() -> ("NewVal"=w1255:bool)  [unwired: 1 in, 5 out]
            n799 = property on="移动" class="Bool (strict)"() -> ("Value"=w1258:bool)  [unwired: 2 in, 2 out]
            n800 = Not(x=w1258) -> (.not. x?=w1257:bool)
            n801 = And(x=w1257, y=w1255) -> (x .and. y?=w1256:bool)
            n802 = case shown="True" w1256 {
              frame False {
              }
              frame True {
                n803 = property on="A1-position-X" class="DigNum (strict)"() -> (error out=w1264:errorcluster, "Value"=w1271:dbl)  [unwired: 2 in, 1 out]
                n804 = property on="A1-position-Y" class="DigNum (strict)"(error in=w1264) -> (error out=w1263:errorcluster, "Value"=w1260:dbl)  [unwired: 1 in, 1 out]
                n805 = Subtract(x=w1260, y=9) -> (x-y=w1259:dbl)
                n806 = Subtract(x=w1271, y=9) -> (x-y=w1262:dbl)
                n807 = vi-ref "goto.vi"() -> (w1269:refnum<vi>)
                n808 = property class="VI"(reference=w1269, error in=w1263) -> ("Name"=w1268:string)  [unwired: 2 out]
                n809 = Open VI Reference(type specifier VI Refnum (for type only)=refnum<vi> refnum, vi path=w1268, options=128) -> (vi reference=w1266:refnum<vi>)  [unwired: 3 in, 1 out]
                n810 = call-by-ref "Start Asynchronous Call"(reference=w1266, "Y(mm)"=w1259, "X(mm)"=w1262) -> ()  [unwired: 10 in, 3 out]
              }
            }
          }
          event "C4": Value Change {
            n811 = event-data() -> ("NewVal"=w1273:bool)  [unwired: 1 in, 5 out]
            n812 = property on="移动" class="Bool (strict)"() -> ("Value"=w1276:bool)  [unwired: 2 in, 2 out]
            n813 = Not(x=w1276) -> (.not. x?=w1275:bool)
            n814 = And(x=w1275, y=w1273) -> (x .and. y?=w1274:bool)
            n815 = case shown="True" w1274 {
              frame False {
              }
              frame True {
                n816 = property on="A1-position-X" class="DigNum (strict)"() -> (error out=w1282:errorcluster, "Value"=w1289:dbl)  [unwired: 2 in, 1 out]
                n817 = property on="A1-position-Y" class="DigNum (strict)"(error in=w1282) -> (error out=w1281:errorcluster, "Value"=w1278:dbl)  [unwired: 1 in, 1 out]
                n818 = Subtract(x=w1278, y=9) -> (x-y=w1277:dbl)
                n819 = Subtract(x=w1289, y=13.5) -> (x-y=w1280:dbl)
                n820 = vi-ref "goto.vi"() -> (w1287:refnum<vi>)
                n821 = property class="VI"(reference=w1287, error in=w1281) -> ("Name"=w1286:string)  [unwired: 2 out]
                n822 = Open VI Reference(type specifier VI Refnum (for type only)=refnum<vi> refnum, vi path=w1286, options=128) -> (vi reference=w1284:refnum<vi>)  [unwired: 3 in, 1 out]
                n823 = call-by-ref "Start Asynchronous Call"(reference=w1284, "Y(mm)"=w1277, "X(mm)"=w1280) -> ()  [unwired: 10 in, 3 out]
              }
            }
          }
          event "C5": Value Change {
            n824 = event-data() -> ("NewVal"=w1291:bool)  [unwired: 1 in, 5 out]
            n825 = property on="移动" class="Bool (strict)"() -> ("Value"=w1294:bool)  [unwired: 2 in, 2 out]
            n826 = Not(x=w1294) -> (.not. x?=w1293:bool)
            n827 = And(x=w1293, y=w1291) -> (x .and. y?=w1292:bool)
            n828 = case shown="True" w1292 {
              frame False {
              }
              frame True {
                n829 = property on="A1-position-X" class="DigNum (strict)"() -> (error out=w1300:errorcluster, "Value"=w1307:dbl)  [unwired: 2 in, 1 out]
                n830 = property on="A1-position-Y" class="DigNum (strict)"(error in=w1300) -> (error out=w1299:errorcluster, "Value"=w1296:dbl)  [unwired: 1 in, 1 out]
                n831 = Subtract(x=w1296, y=9) -> (x-y=w1295:dbl)
                n832 = Subtract(x=w1307, y=18) -> (x-y=w1298:dbl)
                n833 = vi-ref "goto.vi"() -> (w1305:refnum<vi>)
                n834 = property class="VI"(reference=w1305, error in=w1299) -> ("Name"=w1304:string)  [unwired: 2 out]
                n835 = Open VI Reference(type specifier VI Refnum (for type only)=refnum<vi> refnum, vi path=w1304, options=128) -> (vi reference=w1302:refnum<vi>)  [unwired: 3 in, 1 out]
                n836 = call-by-ref "Start Asynchronous Call"(reference=w1302, "Y(mm)"=w1295, "X(mm)"=w1298) -> ()  [unwired: 10 in, 3 out]
              }
            }
          }
          event "C6": Value Change {
            n837 = event-data() -> ("NewVal"=w1309:bool)  [unwired: 1 in, 5 out]
            n838 = property on="移动" class="Bool (strict)"() -> ("Value"=w1312:bool)  [unwired: 2 in, 2 out]
            n839 = Not(x=w1312) -> (.not. x?=w1311:bool)
            n840 = And(x=w1311, y=w1309) -> (x .and. y?=w1310:bool)
            n841 = case shown="True" w1310 {
              frame False {
              }
              frame True {
                n842 = property on="A1-position-X" class="DigNum (strict)"() -> (error out=w1318:errorcluster, "Value"=w1325:dbl)  [unwired: 2 in, 1 out]
                n843 = property on="A1-position-Y" class="DigNum (strict)"(error in=w1318) -> (error out=w1317:errorcluster, "Value"=w1314:dbl)  [unwired: 1 in, 1 out]
                n844 = Subtract(x=w1314, y=9) -> (x-y=w1313:dbl)
                n845 = Subtract(x=w1325, y=22.5) -> (x-y=w1316:dbl)
                n846 = vi-ref "goto.vi"() -> (w1323:refnum<vi>)
                n847 = property class="VI"(reference=w1323, error in=w1317) -> ("Name"=w1322:string)  [unwired: 2 out]
                n848 = Open VI Reference(type specifier VI Refnum (for type only)=refnum<vi> refnum, vi path=w1322, options=128) -> (vi reference=w1320:refnum<vi>)  [unwired: 3 in, 1 out]
                n849 = call-by-ref "Start Asynchronous Call"(reference=w1320, "Y(mm)"=w1313, "X(mm)"=w1316) -> ()  [unwired: 10 in, 3 out]
              }
            }
          }
          event "C7": Value Change {
            n850 = event-data() -> ("NewVal"=w1327:bool)  [unwired: 1 in, 5 out]
            n851 = property on="移动" class="Bool (strict)"() -> ("Value"=w1330:bool)  [unwired: 2 in, 2 out]
            n852 = Not(x=w1330) -> (.not. x?=w1329:bool)
            n853 = And(x=w1329, y=w1327) -> (x .and. y?=w1328:bool)
            n854 = case shown="True" w1328 {
              frame False {
              }
              frame True {
                n855 = property on="A1-position-X" class="DigNum (strict)"() -> (error out=w1336:errorcluster, "Value"=w1343:dbl)  [unwired: 2 in, 1 out]
                n856 = property on="A1-position-Y" class="DigNum (strict)"(error in=w1336) -> (error out=w1335:errorcluster, "Value"=w1332:dbl)  [unwired: 1 in, 1 out]
                n857 = Subtract(x=w1332, y=9) -> (x-y=w1331:dbl)
                n858 = Subtract(x=w1343, y=27) -> (x-y=w1334:dbl)
                n859 = vi-ref "goto.vi"() -> (w1341:refnum<vi>)
                n860 = property class="VI"(reference=w1341, error in=w1335) -> ("Name"=w1340:string)  [unwired: 2 out]
                n861 = Open VI Reference(type specifier VI Refnum (for type only)=refnum<vi> refnum, vi path=w1340, options=128) -> (vi reference=w1338:refnum<vi>)  [unwired: 3 in, 1 out]
                n862 = call-by-ref "Start Asynchronous Call"(reference=w1338, "Y(mm)"=w1331, "X(mm)"=w1334) -> ()  [unwired: 10 in, 3 out]
              }
            }
          }
          event "C8": Value Change {
            n863 = event-data() -> ("NewVal"=w1345:bool)  [unwired: 1 in, 5 out]
            n864 = property on="移动" class="Bool (strict)"() -> ("Value"=w1348:bool)  [unwired: 2 in, 2 out]
            n865 = Not(x=w1348) -> (.not. x?=w1347:bool)
            n866 = And(x=w1347, y=w1345) -> (x .and. y?=w1346:bool)
            n867 = case shown="True" w1346 {
              frame False {
              }
              frame True {
                n868 = property on="A1-position-X" class="DigNum (strict)"() -> (error out=w1354:errorcluster, "Value"=w1361:dbl)  [unwired: 2 in, 1 out]
                n869 = property on="A1-position-Y" class="DigNum (strict)"(error in=w1354) -> (error out=w1353:errorcluster, "Value"=w1350:dbl)  [unwired: 1 in, 1 out]
                n870 = Subtract(x=w1350, y=9) -> (x-y=w1349:dbl)
                n871 = Subtract(x=w1361, y=31.5) -> (x-y=w1352:dbl)
                n872 = vi-ref "goto.vi"() -> (w1359:refnum<vi>)
                n873 = property class="VI"(reference=w1359, error in=w1353) -> ("Name"=w1358:string)  [unwired: 2 out]
                n874 = Open VI Reference(type specifier VI Refnum (for type only)=refnum<vi> refnum, vi path=w1358, options=128) -> (vi reference=w1356:refnum<vi>)  [unwired: 3 in, 1 out]
                n875 = call-by-ref "Start Asynchronous Call"(reference=w1356, "Y(mm)"=w1349, "X(mm)"=w1352) -> ()  [unwired: 10 in, 3 out]
              }
            }
          }
          event "C9": Value Change {
            n876 = event-data() -> ("NewVal"=w1363:bool)  [unwired: 1 in, 5 out]
            n877 = property on="移动" class="Bool (strict)"() -> ("Value"=w1366:bool)  [unwired: 2 in, 2 out]
            n878 = Not(x=w1366) -> (.not. x?=w1365:bool)
            n879 = And(x=w1365, y=w1363) -> (x .and. y?=w1364:bool)
            n880 = case shown="True" w1364 {
              frame False {
              }
              frame True {
                n881 = property on="A1-position-X" class="DigNum (strict)"() -> (error out=w1372:errorcluster, "Value"=w1379:dbl)  [unwired: 2 in, 1 out]
                n882 = property on="A1-position-Y" class="DigNum (strict)"(error in=w1372) -> (error out=w1371:errorcluster, "Value"=w1368:dbl)  [unwired: 1 in, 1 out]
                n883 = Subtract(x=w1368, y=9) -> (x-y=w1367:dbl)
                n884 = Subtract(x=w1379, y=36) -> (x-y=w1370:dbl)
                n885 = vi-ref "goto.vi"() -> (w1377:refnum<vi>)
                n886 = property class="VI"(reference=w1377, error in=w1371) -> ("Name"=w1376:string)  [unwired: 2 out]
                n887 = Open VI Reference(type specifier VI Refnum (for type only)=refnum<vi> refnum, vi path=w1376, options=128) -> (vi reference=w1374:refnum<vi>)  [unwired: 3 in, 1 out]
                n888 = call-by-ref "Start Asynchronous Call"(reference=w1374, "Y(mm)"=w1367, "X(mm)"=w1370) -> ()  [unwired: 10 in, 3 out]
              }
            }
          }
          event "C10": Value Change {
            n889 = event-data() -> ("NewVal"=w1381:bool)  [unwired: 1 in, 5 out]
            n890 = property on="移动" class="Bool (strict)"() -> ("Value"=w1384:bool)  [unwired: 2 in, 2 out]
            n891 = Not(x=w1384) -> (.not. x?=w1383:bool)
            n892 = And(x=w1383, y=w1381) -> (x .and. y?=w1382:bool)
            n893 = case shown="True" w1382 {
              frame False {
              }
              frame True {
                n894 = property on="A1-position-X" class="DigNum (strict)"() -> (error out=w1390:errorcluster, "Value"=w1397:dbl)  [unwired: 2 in, 1 out]
                n895 = property on="A1-position-Y" class="DigNum (strict)"(error in=w1390) -> (error out=w1389:errorcluster, "Value"=w1386:dbl)  [unwired: 1 in, 1 out]
                n896 = Subtract(x=w1386, y=9) -> (x-y=w1385:dbl)
                n897 = Subtract(x=w1397, y=40.5) -> (x-y=w1388:dbl)
                n898 = vi-ref "goto.vi"() -> (w1395:refnum<vi>)
                n899 = property class="VI"(reference=w1395, error in=w1389) -> ("Name"=w1394:string)  [unwired: 2 out]
                n900 = Open VI Reference(type specifier VI Refnum (for type only)=refnum<vi> refnum, vi path=w1394, options=128) -> (vi reference=w1392:refnum<vi>)  [unwired: 3 in, 1 out]
                n901 = call-by-ref "Start Asynchronous Call"(reference=w1392, "Y(mm)"=w1385, "X(mm)"=w1388) -> ()  [unwired: 10 in, 3 out]
              }
            }
          }
          event "C11": Value Change {
            n902 = event-data() -> ("NewVal"=w1399:bool)  [unwired: 1 in, 5 out]
            n903 = property on="移动" class="Bool (strict)"() -> ("Value"=w1402:bool)  [unwired: 2 in, 2 out]
            n904 = Not(x=w1402) -> (.not. x?=w1401:bool)
            n905 = And(x=w1401, y=w1399) -> (x .and. y?=w1400:bool)
            n906 = case shown="True" w1400 {
              frame False {
              }
              frame True {
                n907 = property on="A1-position-X" class="DigNum (strict)"() -> (error out=w1408:errorcluster, "Value"=w1415:dbl)  [unwired: 2 in, 1 out]
                n908 = property on="A1-position-Y" class="DigNum (strict)"(error in=w1408) -> (error out=w1407:errorcluster, "Value"=w1404:dbl)  [unwired: 1 in, 1 out]
                n909 = Subtract(x=w1404, y=9) -> (x-y=w1403:dbl)
                n910 = Subtract(x=w1415, y=45) -> (x-y=w1406:dbl)
                n911 = vi-ref "goto.vi"() -> (w1413:refnum<vi>)
                n912 = property class="VI"(reference=w1413, error in=w1407) -> ("Name"=w1412:string)  [unwired: 2 out]
                n913 = Open VI Reference(type specifier VI Refnum (for type only)=refnum<vi> refnum, vi path=w1412, options=128) -> (vi reference=w1410:refnum<vi>)  [unwired: 3 in, 1 out]
                n914 = call-by-ref "Start Asynchronous Call"(reference=w1410, "Y(mm)"=w1403, "X(mm)"=w1406) -> ()  [unwired: 10 in, 3 out]
              }
            }
          }
          event "C12": Value Change {
            n915 = event-data() -> ("NewVal"=w1417:bool)  [unwired: 1 in, 5 out]
            n916 = property on="移动" class="Bool (strict)"() -> ("Value"=w1420:bool)  [unwired: 2 in, 2 out]
            n917 = Not(x=w1420) -> (.not. x?=w1419:bool)
            n918 = And(x=w1419, y=w1417) -> (x .and. y?=w1418:bool)
            n919 = case shown="True" w1418 {
              frame False {
              }
              frame True {
                n920 = property on="A1-position-X" class="DigNum (strict)"() -> (error out=w1426:errorcluster, "Value"=w1433:dbl)  [unwired: 2 in, 1 out]
                n921 = property on="A1-position-Y" class="DigNum (strict)"(error in=w1426) -> (error out=w1425:errorcluster, "Value"=w1422:dbl)  [unwired: 1 in, 1 out]
                n922 = Subtract(x=w1422, y=9) -> (x-y=w1421:dbl)
                n923 = Subtract(x=w1433, y=49.5) -> (x-y=w1424:dbl)
                n924 = vi-ref "goto.vi"() -> (w1431:refnum<vi>)
                n925 = property class="VI"(reference=w1431, error in=w1425) -> ("Name"=w1430:string)  [unwired: 2 out]
                n926 = Open VI Reference(type specifier VI Refnum (for type only)=refnum<vi> refnum, vi path=w1430, options=128) -> (vi reference=w1428:refnum<vi>)  [unwired: 3 in, 1 out]
                n927 = call-by-ref "Start Asynchronous Call"(reference=w1428, "Y(mm)"=w1421, "X(mm)"=w1424) -> ()  [unwired: 10 in, 3 out]
              }
            }
          }
          event "D1": Value Change {
            n928 = event-data() -> ("NewVal"=w1435:bool)  [unwired: 1 in, 5 out]
            n929 = property on="移动" class="Bool (strict)"() -> ("Value"=w1438:bool)  [unwired: 2 in, 2 out]
            n930 = Not(x=w1438) -> (.not. x?=w1437:bool)
            n931 = And(x=w1437, y=w1435) -> (x .and. y?=w1436:bool)
            n932 = case shown="True" w1436 {
              frame False {
              }
              frame True {
                n933 = property on="A1-position-X" class="DigNum (strict)"() -> (error out=w1444:errorcluster, "Value"=w1451:dbl)  [unwired: 2 in, 1 out]
                n934 = property on="A1-position-Y" class="DigNum (strict)"(error in=w1444) -> (error out=w1443:errorcluster, "Value"=w1440:dbl)  [unwired: 1 in, 1 out]
                n935 = Subtract(x=w1440, y=13.5) -> (x-y=w1439:dbl)
                n936 = Subtract(x=w1451, y=0) -> (x-y=w1442:dbl)
                n937 = vi-ref "goto.vi"() -> (w1449:refnum<vi>)
                n938 = property class="VI"(reference=w1449, error in=w1443) -> ("Name"=w1448:string)  [unwired: 2 out]
                n939 = Open VI Reference(type specifier VI Refnum (for type only)=refnum<vi> refnum, vi path=w1448, options=128) -> (vi reference=w1446:refnum<vi>)  [unwired: 3 in, 1 out]
                n940 = call-by-ref "Start Asynchronous Call"(reference=w1446, "Y(mm)"=w1439, "X(mm)"=w1442) -> ()  [unwired: 10 in, 3 out]
              }
            }
          }
          event "D2": Value Change {
            n941 = event-data() -> ("NewVal"=w1453:bool)  [unwired: 1 in, 5 out]
            n942 = property on="移动" class="Bool (strict)"() -> ("Value"=w1456:bool)  [unwired: 2 in, 2 out]
            n943 = Not(x=w1456) -> (.not. x?=w1455:bool)
            n944 = And(x=w1455, y=w1453) -> (x .and. y?=w1454:bool)
            n945 = case shown="True" w1454 {
              frame False {
              }
              frame True {
                n946 = property on="A1-position-X" class="DigNum (strict)"() -> (error out=w1462:errorcluster, "Value"=w1469:dbl)  [unwired: 2 in, 1 out]
                n947 = property on="A1-position-Y" class="DigNum (strict)"(error in=w1462) -> (error out=w1461:errorcluster, "Value"=w1458:dbl)  [unwired: 1 in, 1 out]
                n948 = Subtract(x=w1458, y=13.5) -> (x-y=w1457:dbl)
                n949 = Subtract(x=w1469, y=4.5) -> (x-y=w1460:dbl)
                n950 = vi-ref "goto.vi"() -> (w1467:refnum<vi>)
                n951 = property class="VI"(reference=w1467, error in=w1461) -> ("Name"=w1466:string)  [unwired: 2 out]
                n952 = Open VI Reference(type specifier VI Refnum (for type only)=refnum<vi> refnum, vi path=w1466, options=128) -> (vi reference=w1464:refnum<vi>)  [unwired: 3 in, 1 out]
                n953 = call-by-ref "Start Asynchronous Call"(reference=w1464, "Y(mm)"=w1457, "X(mm)"=w1460) -> ()  [unwired: 10 in, 3 out]
              }
            }
          }
          event "D3": Value Change {
            n954 = event-data() -> ("NewVal"=w1471:bool)  [unwired: 1 in, 5 out]
            n955 = property on="移动" class="Bool (strict)"() -> ("Value"=w1474:bool)  [unwired: 2 in, 2 out]
            n956 = Not(x=w1474) -> (.not. x?=w1473:bool)
            n957 = And(x=w1473, y=w1471) -> (x .and. y?=w1472:bool)
            n958 = case shown="True" w1472 {
              frame False {
              }
              frame True {
                n959 = property on="A1-position-X" class="DigNum (strict)"() -> (error out=w1480:errorcluster, "Value"=w1487:dbl)  [unwired: 2 in, 1 out]
                n960 = property on="A1-position-Y" class="DigNum (strict)"(error in=w1480) -> (error out=w1479:errorcluster, "Value"=w1476:dbl)  [unwired: 1 in, 1 out]
                n961 = Subtract(x=w1476, y=13.5) -> (x-y=w1475:dbl)
                n962 = Subtract(x=w1487, y=9) -> (x-y=w1478:dbl)
                n963 = vi-ref "goto.vi"() -> (w1485:refnum<vi>)
                n964 = property class="VI"(reference=w1485, error in=w1479) -> ("Name"=w1484:string)  [unwired: 2 out]
                n965 = Open VI Reference(type specifier VI Refnum (for type only)=refnum<vi> refnum, vi path=w1484, options=128) -> (vi reference=w1482:refnum<vi>)  [unwired: 3 in, 1 out]
                n966 = call-by-ref "Start Asynchronous Call"(reference=w1482, "Y(mm)"=w1475, "X(mm)"=w1478) -> ()  [unwired: 10 in, 3 out]
              }
            }
          }
          event "D4": Value Change {
            n967 = event-data() -> ("NewVal"=w1489:bool)  [unwired: 1 in, 5 out]
            n968 = property on="移动" class="Bool (strict)"() -> ("Value"=w1492:bool)  [unwired: 2 in, 2 out]
            n969 = Not(x=w1492) -> (.not. x?=w1491:bool)
            n970 = And(x=w1491, y=w1489) -> (x .and. y?=w1490:bool)
            n971 = case shown="True" w1490 {
              frame False {
              }
              frame True {
                n972 = property on="A1-position-X" class="DigNum (strict)"() -> (error out=w1498:errorcluster, "Value"=w1505:dbl)  [unwired: 2 in, 1 out]
                n973 = property on="A1-position-Y" class="DigNum (strict)"(error in=w1498) -> (error out=w1497:errorcluster, "Value"=w1494:dbl)  [unwired: 1 in, 1 out]
                n974 = Subtract(x=w1494, y=13.5) -> (x-y=w1493:dbl)
                n975 = Subtract(x=w1505, y=13.5) -> (x-y=w1496:dbl)
                n976 = vi-ref "goto.vi"() -> (w1503:refnum<vi>)
                n977 = property class="VI"(reference=w1503, error in=w1497) -> ("Name"=w1502:string)  [unwired: 2 out]
                n978 = Open VI Reference(type specifier VI Refnum (for type only)=refnum<vi> refnum, vi path=w1502, options=128) -> (vi reference=w1500:refnum<vi>)  [unwired: 3 in, 1 out]
                n979 = call-by-ref "Start Asynchronous Call"(reference=w1500, "Y(mm)"=w1493, "X(mm)"=w1496) -> ()  [unwired: 10 in, 3 out]
              }
            }
          }
          event "D5": Value Change {
            n980 = event-data() -> ("NewVal"=w1507:bool)  [unwired: 1 in, 5 out]
            n981 = property on="移动" class="Bool (strict)"() -> ("Value"=w1510:bool)  [unwired: 2 in, 2 out]
            n982 = Not(x=w1510) -> (.not. x?=w1509:bool)
            n983 = And(x=w1509, y=w1507) -> (x .and. y?=w1508:bool)
            n984 = case shown="True" w1508 {
              frame False {
              }
              frame True {
                n985 = property on="A1-position-X" class="DigNum (strict)"() -> (error out=w1516:errorcluster, "Value"=w1523:dbl)  [unwired: 2 in, 1 out]
                n986 = property on="A1-position-Y" class="DigNum (strict)"(error in=w1516) -> (error out=w1515:errorcluster, "Value"=w1512:dbl)  [unwired: 1 in, 1 out]
                n987 = Subtract(x=w1512, y=13.5) -> (x-y=w1511:dbl)
                n988 = Subtract(x=w1523, y=18) -> (x-y=w1514:dbl)
                n989 = vi-ref "goto.vi"() -> (w1521:refnum<vi>)
                n990 = property class="VI"(reference=w1521, error in=w1515) -> ("Name"=w1520:string)  [unwired: 2 out]
                n991 = Open VI Reference(type specifier VI Refnum (for type only)=refnum<vi> refnum, vi path=w1520, options=128) -> (vi reference=w1518:refnum<vi>)  [unwired: 3 in, 1 out]
                n992 = call-by-ref "Start Asynchronous Call"(reference=w1518, "Y(mm)"=w1511, "X(mm)"=w1514) -> ()  [unwired: 10 in, 3 out]
              }
            }
          }
          event "D6": Value Change {
            n993 = event-data() -> ("NewVal"=w1525:bool)  [unwired: 1 in, 5 out]
            n994 = property on="移动" class="Bool (strict)"() -> ("Value"=w1528:bool)  [unwired: 2 in, 2 out]
            n995 = Not(x=w1528) -> (.not. x?=w1527:bool)
            n996 = And(x=w1527, y=w1525) -> (x .and. y?=w1526:bool)
            n997 = case shown="True" w1526 {
              frame False {
              }
              frame True {
                n998 = property on="A1-position-X" class="DigNum (strict)"() -> (error out=w1534:errorcluster, "Value"=w1541:dbl)  [unwired: 2 in, 1 out]
                n999 = property on="A1-position-Y" class="DigNum (strict)"(error in=w1534) -> (error out=w1533:errorcluster, "Value"=w1530:dbl)  [unwired: 1 in, 1 out]
                n1000 = Subtract(x=w1530, y=13.5) -> (x-y=w1529:dbl)
                n1001 = Subtract(x=w1541, y=22.5) -> (x-y=w1532:dbl)
                n1002 = vi-ref "goto.vi"() -> (w1539:refnum<vi>)
                n1003 = property class="VI"(reference=w1539, error in=w1533) -> ("Name"=w1538:string)  [unwired: 2 out]
                n1004 = Open VI Reference(type specifier VI Refnum (for type only)=refnum<vi> refnum, vi path=w1538, options=128) -> (vi reference=w1536:refnum<vi>)  [unwired: 3 in, 1 out]
                n1005 = call-by-ref "Start Asynchronous Call"(reference=w1536, "Y(mm)"=w1529, "X(mm)"=w1532) -> ()  [unwired: 10 in, 3 out]
              }
            }
          }
          event "D7": Value Change {
            n1006 = event-data() -> ("NewVal"=w1543:bool)  [unwired: 1 in, 5 out]
            n1007 = property on="移动" class="Bool (strict)"() -> ("Value"=w1546:bool)  [unwired: 2 in, 2 out]
            n1008 = Not(x=w1546) -> (.not. x?=w1545:bool)
            n1009 = And(x=w1545, y=w1543) -> (x .and. y?=w1544:bool)
            n1010 = case shown="True" w1544 {
              frame False {
              }
              frame True {
                n1011 = property on="A1-position-X" class="DigNum (strict)"() -> (error out=w1552:errorcluster, "Value"=w1559:dbl)  [unwired: 2 in, 1 out]
                n1012 = property on="A1-position-Y" class="DigNum (strict)"(error in=w1552) -> (error out=w1551:errorcluster, "Value"=w1548:dbl)  [unwired: 1 in, 1 out]
                n1013 = Subtract(x=w1548, y=13.5) -> (x-y=w1547:dbl)
                n1014 = Subtract(x=w1559, y=27) -> (x-y=w1550:dbl)
                n1015 = vi-ref "goto.vi"() -> (w1557:refnum<vi>)
                n1016 = property class="VI"(reference=w1557, error in=w1551) -> ("Name"=w1556:string)  [unwired: 2 out]
                n1017 = Open VI Reference(type specifier VI Refnum (for type only)=refnum<vi> refnum, vi path=w1556, options=128) -> (vi reference=w1554:refnum<vi>)  [unwired: 3 in, 1 out]
                n1018 = call-by-ref "Start Asynchronous Call"(reference=w1554, "Y(mm)"=w1547, "X(mm)"=w1550) -> ()  [unwired: 10 in, 3 out]
              }
            }
          }
          event "D8": Value Change {
            n1019 = event-data() -> ("NewVal"=w1560:bool)  [unwired: 1 in, 5 out]
            n1020 = property on="移动" class="Bool (strict)"() -> ("Value"=w1563:bool)  [unwired: 2 in, 2 out]
            n1021 = Not(x=w1563) -> (.not. x?=w1562:bool)
            n1022 = And(x=w1562, y=w1560) -> (x .and. y?=w1561:bool)
            n1023 = case shown="True" w1561 {
              frame False {
              }
              frame True {
                n1024 = property on="A1-position-X" class="DigNum (strict)"() -> (error out=w1570:errorcluster, "Value"=w1577:dbl)  [unwired: 2 in, 1 out]
                n1025 = property on="A1-position-Y" class="DigNum (strict)"(error in=w1570) -> (error out=w1569:errorcluster, "Value"=w1566:dbl)  [unwired: 1 in, 1 out]
                n1026 = Subtract(x=w1566, y=13.5) -> (x-y=w1565:dbl)
                n1027 = Subtract(x=w1577, y=31.5) -> (x-y=w1568:dbl)
                n1028 = vi-ref "goto.vi"() -> (w1575:refnum<vi>)
                n1029 = property class="VI"(reference=w1575, error in=w1569) -> ("Name"=w1574:string)  [unwired: 2 out]
                n1030 = Open VI Reference(type specifier VI Refnum (for type only)=refnum<vi> refnum, vi path=w1574, options=128) -> (vi reference=w1572:refnum<vi>)  [unwired: 3 in, 1 out]
                n1031 = call-by-ref "Start Asynchronous Call"(reference=w1572, "Y(mm)"=w1565, "X(mm)"=w1568) -> ()  [unwired: 10 in, 3 out]
              }
            }
          }
          event "D9": Value Change {
            n1032 = event-data() -> ("NewVal"=w1578:bool)  [unwired: 1 in, 5 out]
            n1033 = property on="移动" class="Bool (strict)"() -> ("Value"=w1581:bool)  [unwired: 2 in, 2 out]
            n1034 = Not(x=w1581) -> (.not. x?=w1580:bool)
            n1035 = And(x=w1580, y=w1578) -> (x .and. y?=w1579:bool)
            n1036 = case shown="True" w1579 {
              frame False {
              }
              frame True {
                n1037 = property on="A1-position-X" class="DigNum (strict)"() -> (error out=w1588:errorcluster, "Value"=w1595:dbl)  [unwired: 2 in, 1 out]
                n1038 = property on="A1-position-Y" class="DigNum (strict)"(error in=w1588) -> (error out=w1587:errorcluster, "Value"=w1584:dbl)  [unwired: 1 in, 1 out]
                n1039 = Subtract(x=w1584, y=13.5) -> (x-y=w1583:dbl)
                n1040 = Subtract(x=w1595, y=36) -> (x-y=w1586:dbl)
                n1041 = vi-ref "goto.vi"() -> (w1593:refnum<vi>)
                n1042 = property class="VI"(reference=w1593, error in=w1587) -> ("Name"=w1592:string)  [unwired: 2 out]
                n1043 = Open VI Reference(type specifier VI Refnum (for type only)=refnum<vi> refnum, vi path=w1592, options=128) -> (vi reference=w1590:refnum<vi>)  [unwired: 3 in, 1 out]
                n1044 = call-by-ref "Start Asynchronous Call"(reference=w1590, "Y(mm)"=w1583, "X(mm)"=w1586) -> ()  [unwired: 10 in, 3 out]
              }
            }
          }
          event "D10": Value Change {
            n1045 = event-data() -> ("NewVal"=w1596:bool)  [unwired: 1 in, 5 out]
            n1046 = property on="移动" class="Bool (strict)"() -> ("Value"=w1599:bool)  [unwired: 2 in, 2 out]
            n1047 = Not(x=w1599) -> (.not. x?=w1598:bool)
            n1048 = And(x=w1598, y=w1596) -> (x .and. y?=w1597:bool)
            n1049 = case shown="True" w1597 {
              frame False {
              }
              frame True {
                n1050 = property on="A1-position-X" class="DigNum (strict)"() -> (error out=w1606:errorcluster, "Value"=w1613:dbl)  [unwired: 2 in, 1 out]
                n1051 = property on="A1-position-Y" class="DigNum (strict)"(error in=w1606) -> (error out=w1605:errorcluster, "Value"=w1602:dbl)  [unwired: 1 in, 1 out]
                n1052 = Subtract(x=w1602, y=13.5) -> (x-y=w1601:dbl)
                n1053 = Subtract(x=w1613, y=40.5) -> (x-y=w1604:dbl)
                n1054 = vi-ref "goto.vi"() -> (w1611:refnum<vi>)
                n1055 = property class="VI"(reference=w1611, error in=w1605) -> ("Name"=w1610:string)  [unwired: 2 out]
                n1056 = Open VI Reference(type specifier VI Refnum (for type only)=refnum<vi> refnum, vi path=w1610, options=128) -> (vi reference=w1608:refnum<vi>)  [unwired: 3 in, 1 out]
                n1057 = call-by-ref "Start Asynchronous Call"(reference=w1608, "Y(mm)"=w1601, "X(mm)"=w1604) -> ()  [unwired: 10 in, 3 out]
              }
            }
          }
          event "D11": Value Change {
            n1058 = event-data() -> ("NewVal"=w1614:bool)  [unwired: 1 in, 5 out]
            n1059 = property on="移动" class="Bool (strict)"() -> ("Value"=w1617:bool)  [unwired: 2 in, 2 out]
            n1060 = Not(x=w1617) -> (.not. x?=w1616:bool)
            n1061 = And(x=w1616, y=w1614) -> (x .and. y?=w1615:bool)
            n1062 = case shown="True" w1615 {
              frame False {
              }
              frame True {
                n1063 = property on="A1-position-X" class="DigNum (strict)"() -> (error out=w1624:errorcluster, "Value"=w1631:dbl)  [unwired: 2 in, 1 out]
                n1064 = property on="A1-position-Y" class="DigNum (strict)"(error in=w1624) -> (error out=w1623:errorcluster, "Value"=w1620:dbl)  [unwired: 1 in, 1 out]
                n1065 = Subtract(x=w1620, y=13.5) -> (x-y=w1619:dbl)
                n1066 = Subtract(x=w1631, y=45) -> (x-y=w1622:dbl)
                n1067 = vi-ref "goto.vi"() -> (w1629:refnum<vi>)
                n1068 = property class="VI"(reference=w1629, error in=w1623) -> ("Name"=w1628:string)  [unwired: 2 out]
                n1069 = Open VI Reference(type specifier VI Refnum (for type only)=refnum<vi> refnum, vi path=w1628, options=128) -> (vi reference=w1626:refnum<vi>)  [unwired: 3 in, 1 out]
                n1070 = call-by-ref "Start Asynchronous Call"(reference=w1626, "Y(mm)"=w1619, "X(mm)"=w1622) -> ()  [unwired: 10 in, 3 out]
              }
            }
          }
          event "D12": Value Change {
            n1071 = event-data() -> ("NewVal"=w1632:bool)  [unwired: 1 in, 5 out]
            n1072 = property on="移动" class="Bool (strict)"() -> ("Value"=w1635:bool)  [unwired: 2 in, 2 out]
            n1073 = Not(x=w1635) -> (.not. x?=w1634:bool)
            n1074 = And(x=w1634, y=w1632) -> (x .and. y?=w1633:bool)
            n1075 = case shown="True" w1633 {
              frame False {
              }
              frame True {
                n1076 = property on="A1-position-X" class="DigNum (strict)"() -> (error out=w1642:errorcluster, "Value"=w1649:dbl)  [unwired: 2 in, 1 out]
                n1077 = property on="A1-position-Y" class="DigNum (strict)"(error in=w1642) -> (error out=w1641:errorcluster, "Value"=w1638:dbl)  [unwired: 1 in, 1 out]
                n1078 = Subtract(x=w1638, y=13.5) -> (x-y=w1637:dbl)
                n1079 = Subtract(x=w1649, y=49.5) -> (x-y=w1640:dbl)
                n1080 = vi-ref "goto.vi"() -> (w1647:refnum<vi>)
                n1081 = property class="VI"(reference=w1647, error in=w1641) -> ("Name"=w1646:string)  [unwired: 2 out]
                n1082 = Open VI Reference(type specifier VI Refnum (for type only)=refnum<vi> refnum, vi path=w1646, options=128) -> (vi reference=w1644:refnum<vi>)  [unwired: 3 in, 1 out]
                n1083 = call-by-ref "Start Asynchronous Call"(reference=w1644, "Y(mm)"=w1637, "X(mm)"=w1640) -> ()  [unwired: 10 in, 3 out]
              }
            }
          }
          event "E1": Value Change {
            n1084 = event-data() -> ("NewVal"=w1650:bool)  [unwired: 1 in, 5 out]
            n1085 = property on="移动" class="Bool (strict)"() -> ("Value"=w1653:bool)  [unwired: 2 in, 2 out]
            n1086 = Not(x=w1653) -> (.not. x?=w1652:bool)
            n1087 = And(x=w1652, y=w1650) -> (x .and. y?=w1651:bool)
            n1088 = case shown="True" w1651 {
              frame False {
              }
              frame True {
                n1089 = property on="A1-position-X" class="DigNum (strict)"() -> (error out=w1660:errorcluster, "Value"=w1667:dbl)  [unwired: 2 in, 1 out]
                n1090 = property on="A1-position-Y" class="DigNum (strict)"(error in=w1660) -> (error out=w1659:errorcluster, "Value"=w1656:dbl)  [unwired: 1 in, 1 out]
                n1091 = Subtract(x=w1656, y=18.0) -> (x-y=w1655:dbl)
                n1092 = Subtract(x=w1667, y=0) -> (x-y=w1658:dbl)
                n1093 = vi-ref "goto.vi"() -> (w1665:refnum<vi>)
                n1094 = property class="VI"(reference=w1665, error in=w1659) -> ("Name"=w1664:string)  [unwired: 2 out]
                n1095 = Open VI Reference(type specifier VI Refnum (for type only)=refnum<vi> refnum, vi path=w1664, options=128) -> (vi reference=w1662:refnum<vi>)  [unwired: 3 in, 1 out]
                n1096 = call-by-ref "Start Asynchronous Call"(reference=w1662, "Y(mm)"=w1655, "X(mm)"=w1658) -> ()  [unwired: 10 in, 3 out]
              }
            }
          }
          event "E2": Value Change {
            n1097 = event-data() -> ("NewVal"=w1668:bool)  [unwired: 1 in, 5 out]
            n1098 = property on="移动" class="Bool (strict)"() -> ("Value"=w1671:bool)  [unwired: 2 in, 2 out]
            n1099 = Not(x=w1671) -> (.not. x?=w1670:bool)
            n1100 = And(x=w1670, y=w1668) -> (x .and. y?=w1669:bool)
            n1101 = case shown="True" w1669 {
              frame False {
              }
              frame True {
                n1102 = property on="A1-position-X" class="DigNum (strict)"() -> (error out=w1678:errorcluster, "Value"=w1685:dbl)  [unwired: 2 in, 1 out]
                n1103 = property on="A1-position-Y" class="DigNum (strict)"(error in=w1678) -> (error out=w1677:errorcluster, "Value"=w1674:dbl)  [unwired: 1 in, 1 out]
                n1104 = Subtract(x=w1674, y=18.0) -> (x-y=w1673:dbl)
                n1105 = Subtract(x=w1685, y=4.5) -> (x-y=w1676:dbl)
                n1106 = vi-ref "goto.vi"() -> (w1683:refnum<vi>)
                n1107 = property class="VI"(reference=w1683, error in=w1677) -> ("Name"=w1682:string)  [unwired: 2 out]
                n1108 = Open VI Reference(type specifier VI Refnum (for type only)=refnum<vi> refnum, vi path=w1682, options=128) -> (vi reference=w1680:refnum<vi>)  [unwired: 3 in, 1 out]
                n1109 = call-by-ref "Start Asynchronous Call"(reference=w1680, "Y(mm)"=w1673, "X(mm)"=w1676) -> ()  [unwired: 10 in, 3 out]
              }
            }
          }
          event "E3": Value Change {
            n1110 = event-data() -> ("NewVal"=w1686:bool)  [unwired: 1 in, 5 out]
            n1111 = property on="移动" class="Bool (strict)"() -> ("Value"=w1689:bool)  [unwired: 2 in, 2 out]
            n1112 = Not(x=w1689) -> (.not. x?=w1688:bool)
            n1113 = And(x=w1688, y=w1686) -> (x .and. y?=w1687:bool)
            n1114 = case shown="True" w1687 {
              frame False {
              }
              frame True {
                n1115 = property on="A1-position-X" class="DigNum (strict)"() -> (error out=w1696:errorcluster, "Value"=w1703:dbl)  [unwired: 2 in, 1 out]
                n1116 = property on="A1-position-Y" class="DigNum (strict)"(error in=w1696) -> (error out=w1695:errorcluster, "Value"=w1692:dbl)  [unwired: 1 in, 1 out]
                n1117 = Subtract(x=w1692, y=18.0) -> (x-y=w1691:dbl)
                n1118 = Subtract(x=w1703, y=9) -> (x-y=w1694:dbl)
                n1119 = vi-ref "goto.vi"() -> (w1701:refnum<vi>)
                n1120 = property class="VI"(reference=w1701, error in=w1695) -> ("Name"=w1700:string)  [unwired: 2 out]
                n1121 = Open VI Reference(type specifier VI Refnum (for type only)=refnum<vi> refnum, vi path=w1700, options=128) -> (vi reference=w1698:refnum<vi>)  [unwired: 3 in, 1 out]
                n1122 = call-by-ref "Start Asynchronous Call"(reference=w1698, "Y(mm)"=w1691, "X(mm)"=w1694) -> ()  [unwired: 10 in, 3 out]
              }
            }
          }
          event "E4": Value Change {
            n1123 = event-data() -> ("NewVal"=w1704:bool)  [unwired: 1 in, 5 out]
            n1124 = property on="移动" class="Bool (strict)"() -> ("Value"=w1707:bool)  [unwired: 2 in, 2 out]
            n1125 = Not(x=w1707) -> (.not. x?=w1706:bool)
            n1126 = And(x=w1706, y=w1704) -> (x .and. y?=w1705:bool)
            n1127 = case shown="True" w1705 {
              frame False {
              }
              frame True {
                n1128 = property on="A1-position-X" class="DigNum (strict)"() -> (error out=w1714:errorcluster, "Value"=w1721:dbl)  [unwired: 2 in, 1 out]
                n1129 = property on="A1-position-Y" class="DigNum (strict)"(error in=w1714) -> (error out=w1713:errorcluster, "Value"=w1710:dbl)  [unwired: 1 in, 1 out]
                n1130 = Subtract(x=w1710, y=18.0) -> (x-y=w1709:dbl)
                n1131 = Subtract(x=w1721, y=13.5) -> (x-y=w1712:dbl)
                n1132 = vi-ref "goto.vi"() -> (w1719:refnum<vi>)
                n1133 = property class="VI"(reference=w1719, error in=w1713) -> ("Name"=w1718:string)  [unwired: 2 out]
                n1134 = Open VI Reference(type specifier VI Refnum (for type only)=refnum<vi> refnum, vi path=w1718, options=128) -> (vi reference=w1716:refnum<vi>)  [unwired: 3 in, 1 out]
                n1135 = call-by-ref "Start Asynchronous Call"(reference=w1716, "Y(mm)"=w1709, "X(mm)"=w1712) -> ()  [unwired: 10 in, 3 out]
              }
            }
          }
          event "E5": Value Change {
            n1136 = event-data() -> ("NewVal"=w1722:bool)  [unwired: 1 in, 5 out]
            n1137 = property on="移动" class="Bool (strict)"() -> ("Value"=w1725:bool)  [unwired: 2 in, 2 out]
            n1138 = Not(x=w1725) -> (.not. x?=w1724:bool)
            n1139 = And(x=w1724, y=w1722) -> (x .and. y?=w1723:bool)
            n1140 = case shown="True" w1723 {
              frame False {
              }
              frame True {
                n1141 = property on="A1-position-X" class="DigNum (strict)"() -> (error out=w1732:errorcluster, "Value"=w1739:dbl)  [unwired: 2 in, 1 out]
                n1142 = property on="A1-position-Y" class="DigNum (strict)"(error in=w1732) -> (error out=w1731:errorcluster, "Value"=w1728:dbl)  [unwired: 1 in, 1 out]
                n1143 = Subtract(x=w1728, y=18.0) -> (x-y=w1727:dbl)
                n1144 = Subtract(x=w1739, y=18) -> (x-y=w1730:dbl)
                n1145 = vi-ref "goto.vi"() -> (w1737:refnum<vi>)
                n1146 = property class="VI"(reference=w1737, error in=w1731) -> ("Name"=w1736:string)  [unwired: 2 out]
                n1147 = Open VI Reference(type specifier VI Refnum (for type only)=refnum<vi> refnum, vi path=w1736, options=128) -> (vi reference=w1734:refnum<vi>)  [unwired: 3 in, 1 out]
                n1148 = call-by-ref "Start Asynchronous Call"(reference=w1734, "Y(mm)"=w1727, "X(mm)"=w1730) -> ()  [unwired: 10 in, 3 out]
              }
            }
          }
          event "E6": Value Change {
            n1149 = event-data() -> ("NewVal"=w1740:bool)  [unwired: 1 in, 5 out]
            n1150 = property on="移动" class="Bool (strict)"() -> ("Value"=w1743:bool)  [unwired: 2 in, 2 out]
            n1151 = Not(x=w1743) -> (.not. x?=w1742:bool)
            n1152 = And(x=w1742, y=w1740) -> (x .and. y?=w1741:bool)
            n1153 = case shown="True" w1741 {
              frame False {
              }
              frame True {
                n1154 = property on="A1-position-X" class="DigNum (strict)"() -> (error out=w1750:errorcluster, "Value"=w1757:dbl)  [unwired: 2 in, 1 out]
                n1155 = property on="A1-position-Y" class="DigNum (strict)"(error in=w1750) -> (error out=w1749:errorcluster, "Value"=w1746:dbl)  [unwired: 1 in, 1 out]
                n1156 = Subtract(x=w1746, y=18.0) -> (x-y=w1745:dbl)
                n1157 = Subtract(x=w1757, y=22.5) -> (x-y=w1748:dbl)
                n1158 = vi-ref "goto.vi"() -> (w1755:refnum<vi>)
                n1159 = property class="VI"(reference=w1755, error in=w1749) -> ("Name"=w1754:string)  [unwired: 2 out]
                n1160 = Open VI Reference(type specifier VI Refnum (for type only)=refnum<vi> refnum, vi path=w1754, options=128) -> (vi reference=w1752:refnum<vi>)  [unwired: 3 in, 1 out]
                n1161 = call-by-ref "Start Asynchronous Call"(reference=w1752, "Y(mm)"=w1745, "X(mm)"=w1748) -> ()  [unwired: 10 in, 3 out]
              }
            }
          }
          event "ShutDownSystem": Value Change {
            n1162 = event-data() -> ("NewVal"=w1760:bool)  [unwired: 1 in, 5 out]
            n1163 = case shown="True" w1760 {
              tunnel: w1759 -> [_ w1764]
              frame False {
              }
              frame True {
                n1164 = Unbundle By Name(w1764) -> ("ConfiguredPumpCom"=w1763:refnum<visa-resource-name>, "ConfiguredLaserCom"=w1762:refnum<visa-resource-name>)
                n1165 = VISA Close(VISA resource name=w1763) -> (error out=w1761:errorcluster)  [unwired: 1 in]
                n1166 = VISA Close(VISA resource name=w1762, error in (no error)=w1761) -> ()  [unwired: 1 out]
              }
            }
          }
        }
      }
    }
  }
  n1167 = Unbundle(w22) -> ("tasks"=w3:T13, "interface"=w2:T12, "error out"=w1:errorcluster)
  n1168 = call "USB6343_Control_v1.6.2.vi"("error in"=w1, "interface"=w2, "tasks"=w3) -> ()  [unwired: 9 in]
  n1169 = call <vilib>:"IMAQdx Enumerate Cameras.vi"() -> ("error out"=w12:errorcluster, "Camera Information Array"=w9:T18)  [unwired: 10 in]
  n1170 = Index Array(array=w9, index=0) -> (element=w11:T19)
  n1171 = Unbundle By Name(w11) -> ("InterfaceName"=w19:string)
  n1172 = while {
    tunnel: w24 -> [w1786]
    tunnel: w23 -> [w1784]
    stop <- FALSE stop-if-true
    n1173 = Unbundle By Name(w1786) -> ("pump semaphore"=w1785:T3, "laser semaphore"=w1781:T3)
    n1174 = Unbundle By Name(w1784) -> ("ConfiguredPumpCom"=w1783:refnum<visa-resource-name>, "ConfiguredLaserCom"=w1771:refnum<visa-resource-name>)
    n1175 = call <vilib>:"Acquire Semaphore.vi"("semaphore"=w1785) -> ("error out"=w1770:errorcluster, "semaphore out"=w1782:T3)  [unwired: 4 in, 1 out]
    n1176 = call "pumpStatus.vi"("VISA resource name"=w1783, "error in (no error)"=w1770) -> ("PumpKW"=→"PumpKW":dbl, "PumpTemp"=→"PumpTemp":u16, "PumpAmps"=→"PumpAmps":dbl, "PumpVolts"=→"PumpVolts":dbl, "TurboSpeed"=→"TurboSpeed":dbl, "error out"=w1769:errorcluster)  [unwired: 8 in]
    n1177 = call <vilib>:"Release Semaphore.vi"("error in (no error)"=w1769, "semaphore"=w1782) -> ("error out"=w1767:errorcluster)  [unwired: 4 in, 1 out]
    n1178 = call <vilib>:"Acquire Semaphore.vi"("error in (no error)"=w1767, "semaphore"=w1781) -> ("error out"=w1768:errorcluster, "semaphore out"=w1766:T3)  [unwired: 3 in, 1 out]
    n1179 = call "Laser-Get-Shotstatus.vi"("VISA resource name"=w1771, "error in (no error)"=w1768) -> ("cluster"=→"cluster":T7, "error out"=w1765:errorcluster)  [unwired: 1 out]
    n1180 = call <vilib>:"Release Semaphore.vi"("error in (no error)"=w1765, "semaphore"=w1766) -> ("error out"=w1780:errorcluster)  [unwired: 4 in, 1 out]
    n1181 = call "Time Delay2"("error in (no error)"=w1780, "Delay Time (s)"=1.0) -> ()  [unwired: 9 in, 1 out]
  }
  n1182 = call <vilib>:"IMAQdx Open Camera.vi"("error in"=w12, "Session In"=w19) -> ("error out"=w6:errorcluster, "Session Out"=w7:T20)  [unwired: 8 in]
  n1183 = property class="IMAQdx" props=["VideoMode", "Width", "Height"](reference=w7, error in=w6, "VideoMode"=u32 13) -> (reference out=w5:T20, error out=w4:errorcluster)  [unwired: 2 out]
  n1184 = call "IMAQ Create"("Image Name"=w19) -> ("New Image"=w14:T2)  [unwired: 4 in, 1 out]
  n1185 = call <vilib>:"IMAQdx Configure Grab.vi"("error in"=w4, "Session In"=w5) -> ("error out"=w18:errorcluster, "Session Out"=w13:T20)  [unwired: 8 in]
  n1186 = while {
    tunnel: w18 -> [w1793]
    tunnel: w13 -> [w1792]
    tunnel: w14 -> [w1791]
    tunnel: [w1790] -> w15
    tunnel: [w1789] -> w16
    tunnel: [w1788] -> w17
    stop <- FALSE stop-if-true
    n1187 = call <vilib>:"IMAQdx Grab.vi"("error in"=w1793, "Image In"=w1791, "Session In"=w1792) -> ("error out"=w1790:errorcluster, "Image Out"=w1788:T2, "Session Out"=w1789:T20)  [unwired: 5 in, 1 out]
    "Image" <- w1788
  }
  n1188 = call "IMAQ Dispose"("Image"=w17) -> ()  [unwired: 5 in, 1 out]
  n1189 = call <vilib>:"IMAQdx Close Camera.vi"("error in"=w15, "Session In"=w16) -> ()  [unwired: 9 in, 1 out]
